vi "Copy of Copy of Sievert_auto_RLC-2.vi"() -> ()   [LabVIEW 2011]
uses:
  <vilib>/Utility/error.llb/DialogType.ctl
  <vilib>/DAQmx/write.llb/DAQmx Write (Digital Bool 1Line 1Point).vi
  <vilib>/DAQmx/create/channels.llb/DAQmx Create Channel (DO-Digital Output).vi
  <vilib>/DAQmx/miscellaneous.llb/DAQmx Fill In Error Info.vi
  <vilib>/Analysis/Matrix/Numeric/Conversions/Array To Matrix - RA.vi
  <vilib>/Analysis/Matrix/Numeric/Conversions/Matrix To Array - RM.vi
  <vilib>/Analysis/NI_AALPro.lvlib
  <vilib>/Analysis/Matrix/NI_Matrix.lvlib
  <vilib>/Analysis/NI_AALBase.lvlib
panel:
  out "Boolean 4":bool
  out "tempo carga":dbl[](array[numeric])
  out "PCh1":dbl[](array[numeric])
  out "output array 2":u32[](array[numeric])
  out "MEASURE C [F ]":dbl
  out "Automatico 2":dynamicdata(graph)
  out "termopar K 2":dbl format="%.3g"
  out "termopar K":string
  out "output NTC":dbl
  out "termopar K":dbl format="%.3g"
  out "path RLC_mean":path
  out "estagio 5":i32
  out "FIM":bool=TRUE
  out "limpo":i32
  in  "N fit":i32=5
  in  "ATM wait":u32
  in  "SET":i32
  in  "time subarray":dbl[](array[numeric])
  out "P cinetica mean 2":dbl format="%0.2f"
  out "T cinetica mean 3":dbl format="%0.2f"
  out "Time cinetica":dbl format="%0.2f"
  in  "T subarray 3":dbl[](array[numeric])
  in  "P T  index 2":i32
  in  "P subarray 2":dbl[](array[numeric])
  in  "Numeric":dbl=4.0
  in  "T subarray 2":dbl[](array[numeric])
  out "T cinetica mean 2":dbl format="%0.2f"
  out "P cinetica mean":dbl format="%0.2f"
  in  "P subarray":dbl[](array[numeric])
  in  "P T  index":i32
  out "T string":string
  out "P string":string
  out "path 2_cinetica":path
  out "Polynomial Coefficients 2":dbl[](array[numeric])
  out "Polynomial Coefficients":dbl[](array[numeric])
  in  "Count SET":i32=-1
  out "Set atual":i32
  out "mean pressure":dbl format="%.4p"
  out "Set number":i32
  in  "Tab Control":T1(tab)
  out "T":bool
  out "ZPf2":bool
  out "Pf2":bool
  out "Pit":bool
  out "ZPit":bool
  out "Camara":dbl(slide) scale=0.0..59.5 scale format="%#_3g"
  in  "Save manual":bool
  in  "Open Button":bool
  out "String 2":string
  in  "ATM":bool
  in  "Câmara":bool
  in  "Vácuo":bool
  in  "Entrada Gás":bool
  in  "Manual Ctrl":bool
  in  "stop":bool
  out "P-manual":dynamicdata(graph)
  in  "Clear":bool
  out "path":path
  in  "Nota":string
  in  "Sample name":string
  in  "File name":string
  out "Linear Model Graph":dbl[][](graph)
  out "Linear Model Graph 2":dbl[][](graph)
  in  "N to fit":i32=60
  out "N":i32
  out "Vácuo":bool
  out "Atm":bool
  out "Câmara":bool
  out "String_cinetica":string
  out "Vol Ref":dbl(slide) scale=0.0..60.0 scale format="%#_4f"
  out "Entrada gás":bool
  in  "Guardar\nCinetica":bool
  out "p fit":dbl format="%#_4g"
  out "T fit":dbl format="%#_4g"
  in  "Open Button 2":bool
  out "x >= y?":bool
  in  "seconds":dbl
  out "Elapsed Time (sec)":dbl format="%.1f"
  out "bar/N":dbl format="%#_4p"
  in  "correção NTC":dbl
  out "mean H2 sensor (V)":dbl format="%#_4p"
  out "Boolean 3":bool
  out "String 3":string
  out "T 2":bool
  out "ZPit 2":bool
  out "Pit 2":bool
  out "Pf2 2":bool
  out "ZPf2 2":bool
  out "Camara 2":dbl(slide) scale=0.0..25.0 scale format="%#_3g"
  out "Vácuo 2":bool
  out "Atm 2":bool
  out "Câmara 2":bool
  out "Vol Ref 3":dbl(slide) scale=0.0..25.0 scale format="%#_4f"
  out "Entrada gás 2":bool
  in  "Auto Ctrl":bool
  in  "Play Button":bool
  out "time stamp":timestamp format="%<%.2X>T"
  out "Time (sec)":dbl format="%.1f"
  in  "clear":bool
  out "Automatico":dynamicdata(graph)
  out "Linear P":T2(graph)
  out "Linear T":T2(graph)
  out "Contador":i32
  in  "STOP (bar/s)":dbl format="%#_5p"
  out "P (bar/s)":dbl format="%#_5p"
  out "bar/s":dbl format="%#_4p"
  out "P fit":dbl format="%#_4g"
  out "T fit":dbl format="%#_4g"
  out "x = y?":bool
  out "teste slope":i32
  in  "Set P auto":dbl
  in  "Step P":dbl=2.0
  in  "P_max":dbl=2.0
  in  "P_max camara":dbl=2.0
  out "Carga":bool=TRUE
  out "Descarga":bool
  out "String":string
  in  "P_min descarga":dbl
  in  "Boolean":bool
  in  "Array":dbl[](array[numeric])
  out "Boolean 2":bool
  out "Desc SET":i32
  in  "ZPf2 time":dbl=24.0
  in  "Ciclos":dbl
  out "Efetuados":dbl
  in  "patamar milliseconds to wait":u32=500
  in  "N fit patamar":i32=100
  in  "Step ZPit":dbl
  out "Read ZPit":bool
  in  "Estagio auto":i32
  out "mean H2 sensor":dbl format="%#_4p"
  in  "Ntest":i32=5
  in  "N fit 2":i32=100
  in  "C50L":bool
  in  "C50N":bool
  in  "C100L":bool
  in  "C100N":bool
  in  "C1KL":bool
  in  "C1KN":bool
  in  "C10KL":bool
  in  "C10KN":bool
  out "String 4":string
  in  "Combo Box":string(combo)
  in  "Refresh Button":bool
  in  "Close RLC 2":bool
  in  "RLC on/off":bool
  out "mean 16":dbl format="%.3p"
  out "mean 15":dbl format="%.3p"
  out "mean 14":dbl format="%.3p"
  out "mean 13":dbl format="%.3p"
  out "mean 12":dbl format="%.3p"
  out "mean 11":dbl format="%.3p"
  out "mean 10":dbl format="%.3p"
  out "mean 9":dbl format="%.3p"
  out "mean 8":dbl format="%.3p"
  out "mean 7":dbl format="%.3p"
  out "mean 6":dbl format="%.3p"
  out "mean 5":dbl format="%.3p"
  out "mean 4":dbl format="%.3p"
  out "mean 3":dbl format="%.3p"
  out "mean 2":dbl format="%.3p"
  out "mean":dbl format="%.3p"
  out "SET 2":dbl
  out "C-50-L":bool
  out "MEASURE B":dbl
  out "MEASURE A":dbl
  out "C-50-N":bool
  out "MEASURE B 2":dbl
  out "MEASURE A 2":dbl
  out "C-100-L":bool
  out "MEASURE B 3":dbl
  out "MEASURE A 3":dbl
  out "C-100-N":bool
  out "MEASURE B 4":dbl
  out "MEASURE A 4":dbl
  out "C-1K-L":bool
  out "MEASURE B 5":dbl
  out "MEASURE A 5":dbl
  out "C-1K-N":bool
  out "MEASURE B 6":dbl
  out "MEASURE A 6":dbl
  out "C-10K-L":bool
  out "MEASURE B 7":dbl
  out "MEASURE A 7":dbl
  out "C-10K-N":bool
  out "MEASURE B 8":dbl
  out "MEASURE A 8":dbl
  out "Z-50-L":bool
  out "MEASURE B 9":dbl
  out "MEASURE A 9":dbl
  out "Z-50-N":bool
  out "MEASURE B 10":dbl
  out "MEASURE A 10":dbl
  out "Z-100-L":bool
  out "MEASURE B 11":dbl
  out "MEASURE A 11":dbl
  out "Z-100-N":bool
  out "MEASURE B 12":dbl
  out "MEASURE A 12":dbl
  out "Z-1K-L":bool
  out "MEASURE B 13":dbl
  out "MEASURE A 13":dbl
  out "Z-1K-N":bool
  out "MEASURE B 14":dbl
  out "MEASURE A 14":dbl
  out "Z-10K-L":bool
  out "MEASURE B 15":dbl
  out "MEASURE A 15":dbl
  out "Z-10K-N":bool
  out "MEASURE B 16":dbl
  out "MEASURE A 16":dbl
  out "RLC300 - digimess":string
  in  "Time RLC":u32=5000
  in  "Ligar RLC":bool
  out "path RLC_completo":path
  out "Waveform Chart P 2":dbl[][](graph)
  out "Waveform Chart":dynamicdata(graph)
  in  "graph RLC":bool
  in  "Refresh Button 2":bool
  in  "Z50L":bool
  in  "Z50N":bool
  in  "Z100L":bool
  in  "Z100N":bool
  in  "Z1KL":bool
  in  "Z1KN":bool
  in  "Z10KL":bool
  in  "Z10KN":bool
  out "Waveform Chart 2":dynamicdata(graph)
  out "XY Graph 2":cluster{"Value":dbl[], "Value":dbl[]}[](graph)
  in  "t-sivert01(s)":dbl
  out "dP/dt (bar/s)":dbl format="%#_5p"
  in  "read - Sievert 01":bool
  # "P vol ref"
  # "P Câmara"
  # "P vol ref"
  # "P Câmara"
  # "C ( F )"
  # "R ( Ohm )"
  # "Z ( Ohm )"
  # "Phase ( deg)"
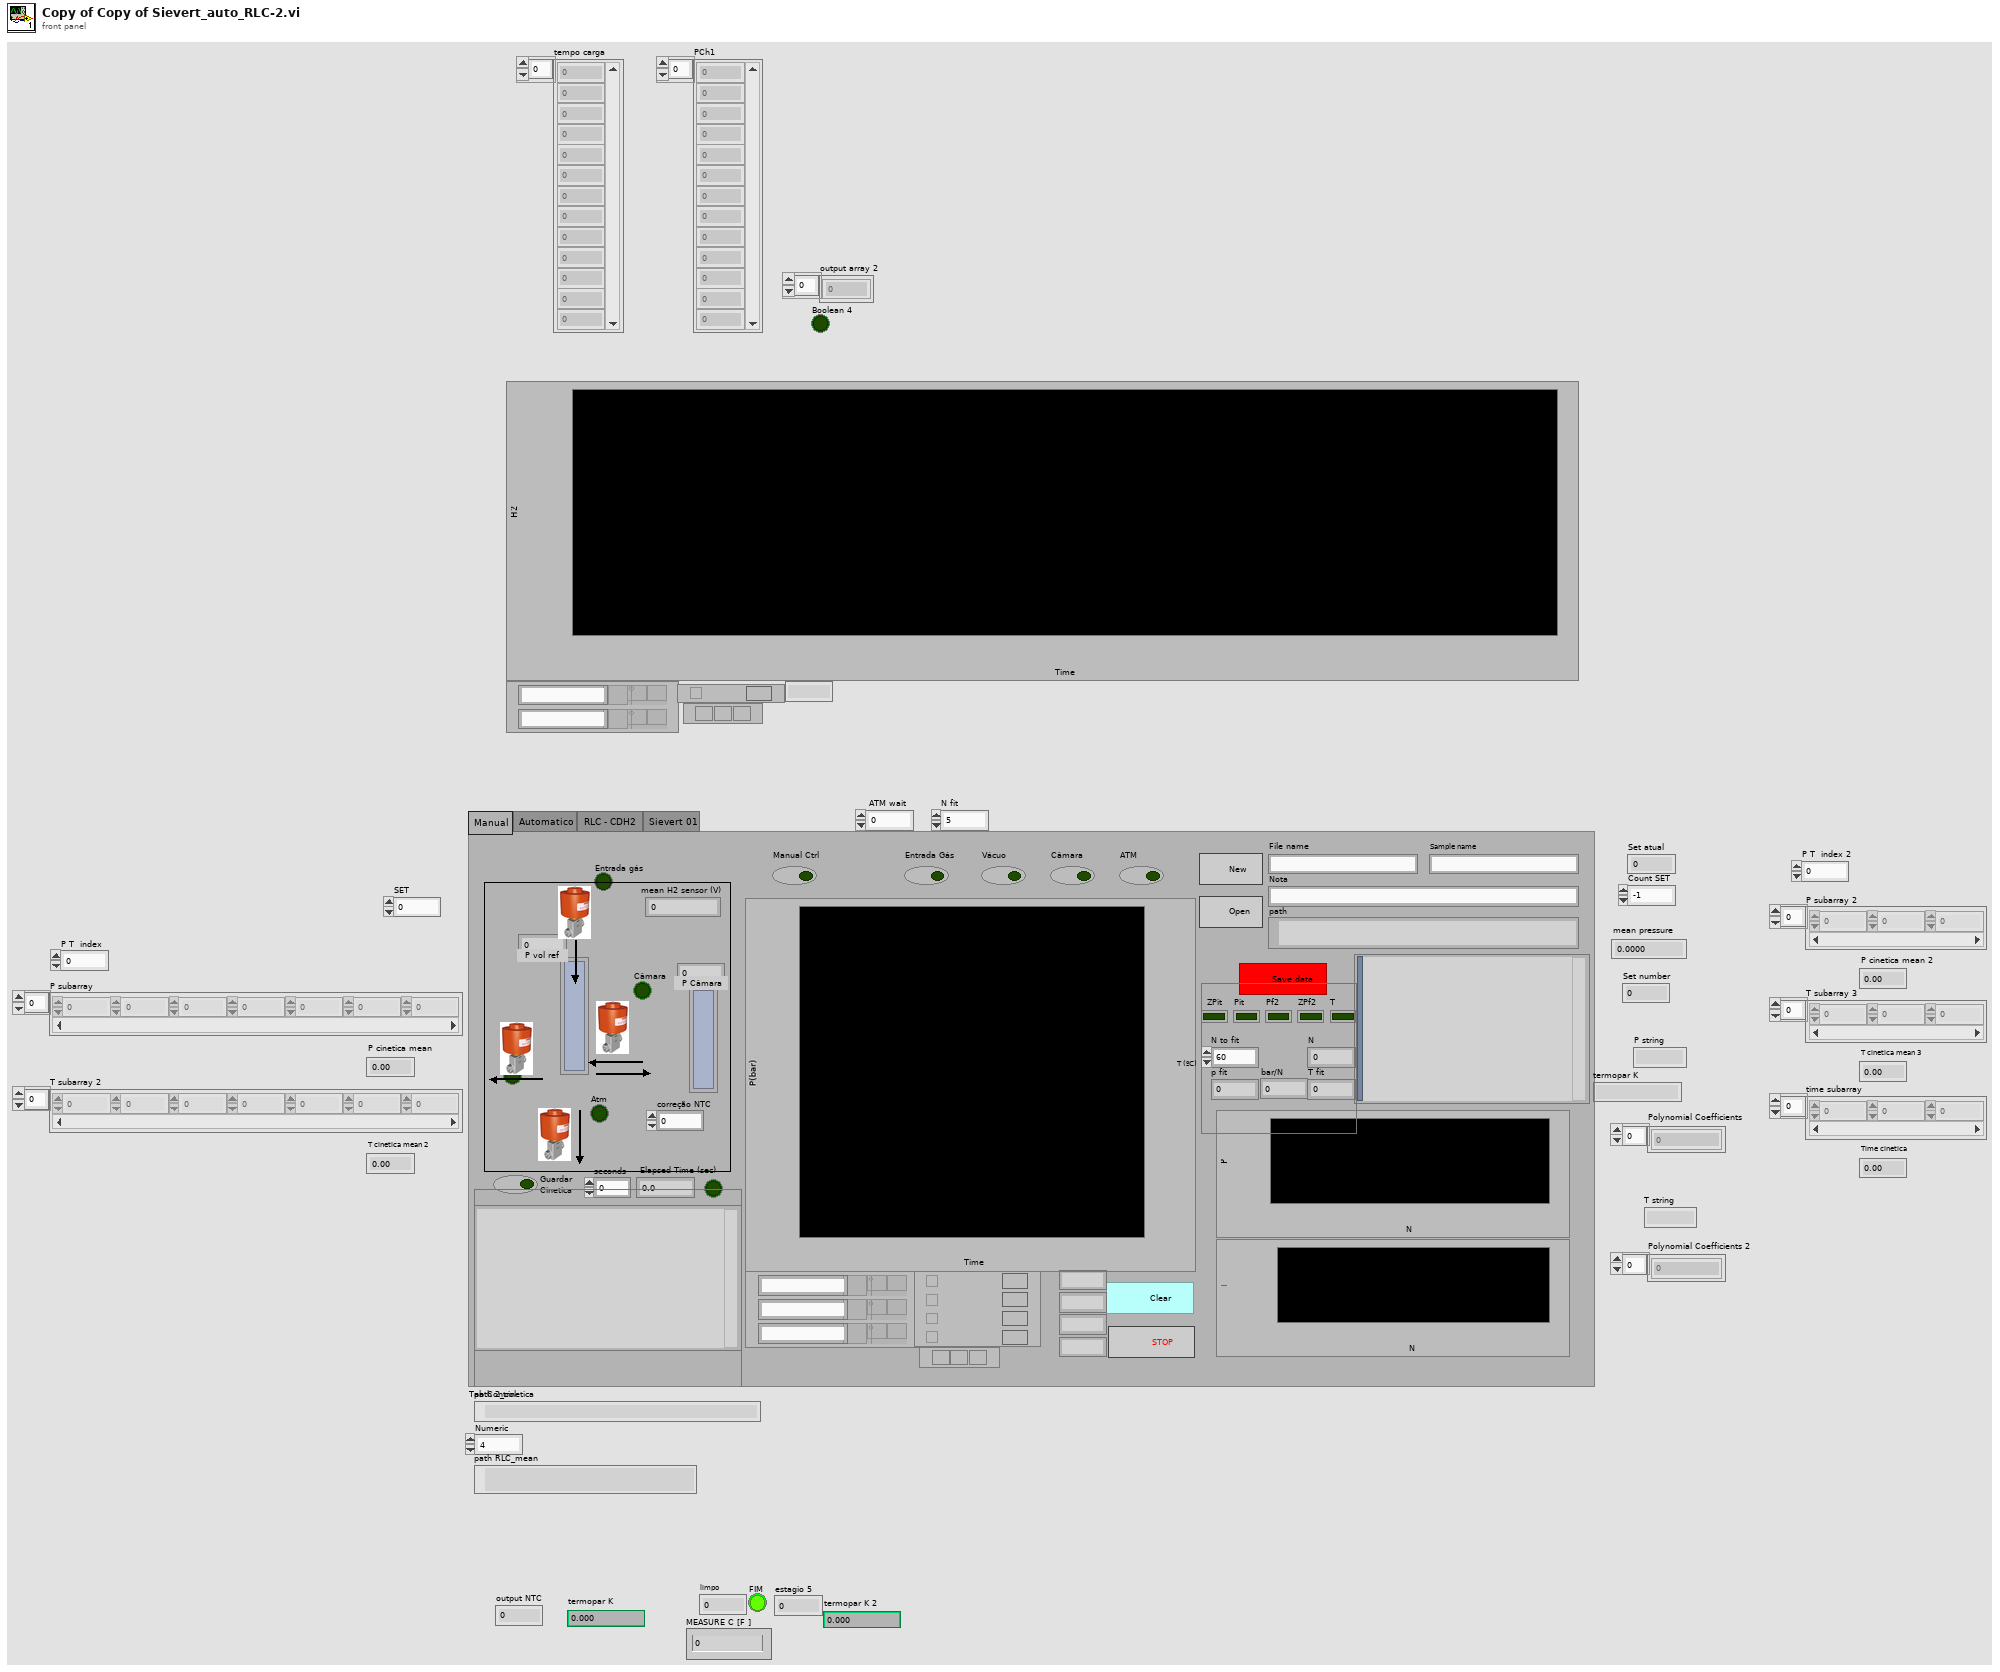
[diagram p1: front panel]
types:
  T1 = enum32{"Manual", "Automatico", "RLC - CDH2", "Sievert 01"}
  T2 = cluster{"Real 2D Array":dbl[], "Best Linear Fit":dbl[]}[]
  T3 = enum16{"open", "replace", "create", "open or create", "replace or create", "replace or create with confirmation"}
  T4 = cluster{"Value":dbl[], "Best Linear Fit":dbl[]}[]
  T5 = typedef "NI_Matrix.lvlib/RealMatrix.ctl" = dbl[][]
  T6 = cluster{"Real 2D Array":dbl[], "Real 2D Array":dbl[]}
  T7 = typedef "DialogType.ctl" = u16
  T8 = cluster{"Real 2D Array":dbl[], "Best Linear Fit":dbl[]}
  T9 = cluster{"Real 2D Array":dbl[], "Best Polynomial Fit":dbl[]}
  T10 = cluster{"Real 2D Array":dbl[], "Best Polynomial Fit":dbl[]}[]
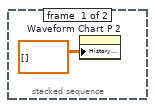
[diagram p5: hidden frame]
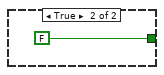
[diagram p10: hidden frame]
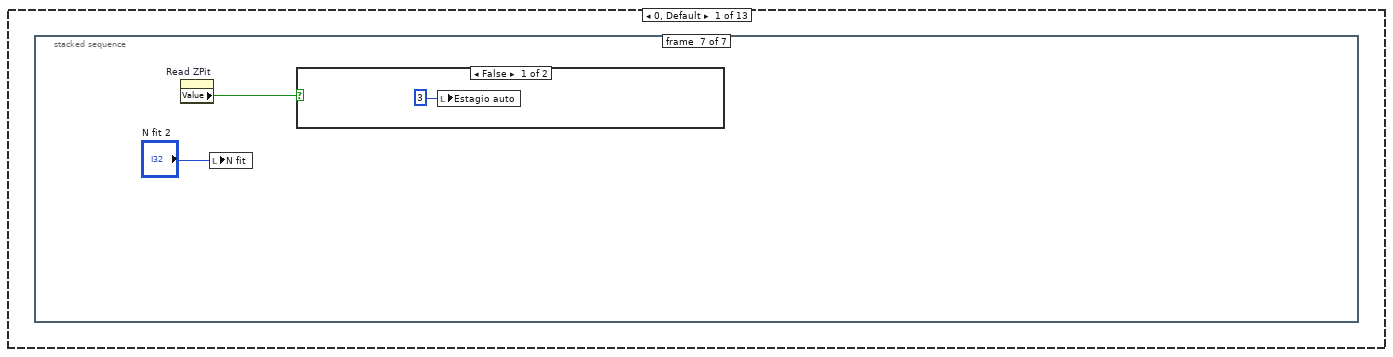
[diagram p15: hidden frame]
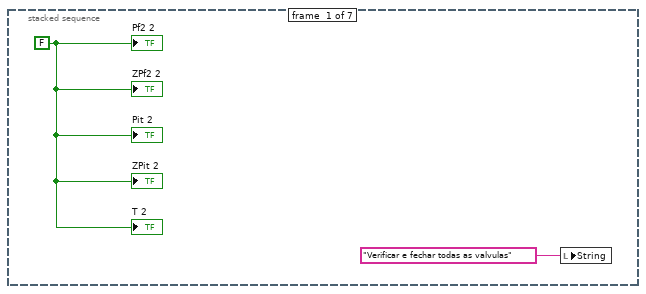
[diagram p16: hidden frame]
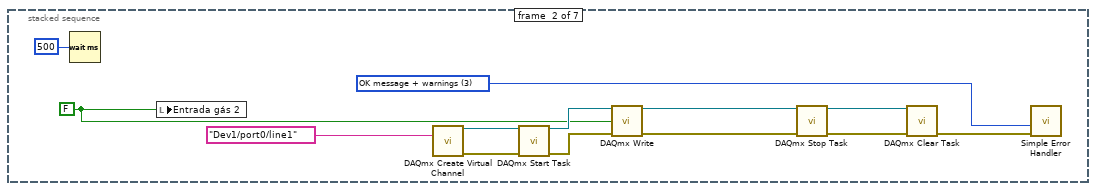
[diagram p17: hidden frame]
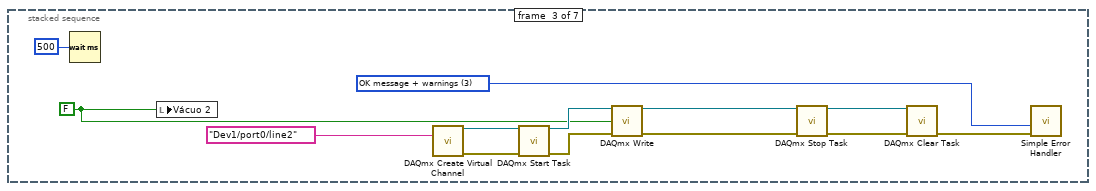
[diagram p18: hidden frame]
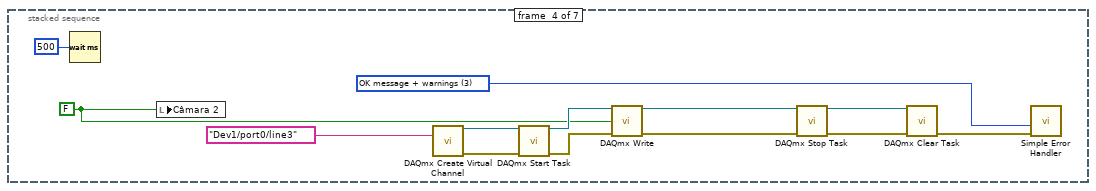
[diagram p19: hidden frame]
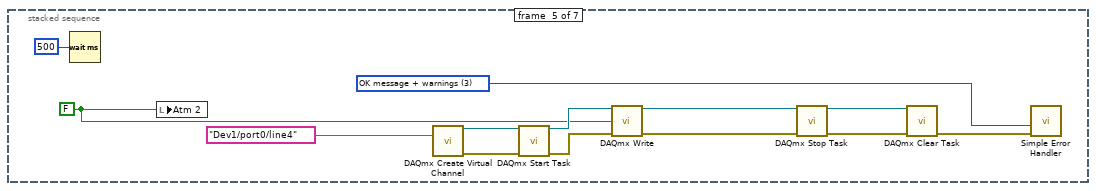
[diagram p20: hidden frame]
diagram:
  w1 = TRUE ("C1KN")
  (unwired) dbl[] [0.5, 1.0, 2.0, 3.0, 4.0, 5.0, 6.0, 7.0, 8.0, 9.0, 10.0, 11.0, 12.0, 13.0, 14.0, 15.0, 16.0, 17.0, 18.0, 19.0, 20.0, 30.0, 40.0, 50.0, 60.0, 70.0] ("Array")
  n1 = local write "N to fit"(5 ("Numeric")) -> ()
  n2 = local write "correção NTC"(0.5 ("correção NTC")) -> ()
  n3 = local write "Step ZPit"(5.0 ("Step ZPit")) -> ()
  n4 = local write "Time RLC"(u32 5 ("Time RLC")) -> ()
  n5 = local write "Ciclos"(0.0 ("Ciclos")) -> ()
  n6 = local write "Desc SET"(0 ("Desc SET")) -> ()
  n7 = local write "Efetuados"(0.0 ("Efetuados")) -> ()
  n8 = local write "estagio 5"(0 ("estagio 5")) -> ()
  n9 = local write "teste slope"(0 ("teste slope")) -> ()
  n10 = local write "SET"(0 ("SET auto")) -> ()
  n11 = local write "limpo"(0 ("limpo")) -> ()
  n12 = local write "N fit"(5 ("N fit")) -> ()
  n13 = local write "ATM wait"(u32 4 ("ATM wait")) -> ()
  n14 = local write "Estagio auto"(0 ("Estagio auto")) -> ()
  n15 = local write "P T  index"(0 ("index")) -> ()
  n16 = local write "seconds"(2.0 ("seconds")) -> ()
  n17 = local write "Read ZPit"(TRUE ("Read ZPit")) -> ()
  n18 = local write "Descarga"(FALSE ("Descarga")) -> ()
  n19 = local write "Carga"(TRUE ("Carga")) -> ()
  n20 = local write "FIM"(FALSE ("FIM")) -> ()
  n21 = local write "P_max"(50.0 ("P_max")) -> ()
  n22 = local write "P_max camara"(25.0 ("P_max camara")) -> ()
  n23 = local write "Set P auto"(0.5 ("Set P auto")) -> ()
  n24 = local write "P_min descarga"(0.025 ("P_min descarga")) -> ()
  n25 = local write "P subarray"(dbl[] [0.0, 1.0] ("subarray")) -> ()
  n26 = local write "T subarray 2"(dbl[] [0.0, 1.0] ("subarray")) -> ()
  n27 = local write "C1KN"(w1) -> ()
  n28 = local write "Z1KN"(w1) -> ()
  n29 = local write "Combo Box"("rlc_read_cCN.py" ("Combo Box")) -> ()
  n30 = local write "t-sivert01(s)"(10.0 ("t-sivert01(s)")) -> ()
  n31 = while {
    tunnel: path "C:/H2_Painel/painel_auto/RLC_CDH" ("Path") -> [w37]
    stop <- w49 stop-if-true
    n32 = property on="FIM" class="Bool (strict)"() -> ("Value"=w47:bool)  [unwired: 2 in, 2 out]
    n33 = property on="path" class="Path"() -> ("Value"=w44:path)  [unwired: 2 in, 2 out]
    n34 = case shown="True" "Ligar RLC" {
      tunnel: w37 -> [_ w224]
      frame False {
      }
      frame True {
        n35 = call "RLC_open.vi"("Path"=w224) -> ("String 2"=w225:string)  [unwired: 9 in, 1 out]
        n36 = local write "RLC300 - digimess"(w225) -> ()
      }
    }
    n37 = case shown="True" "Auto Ctrl" {
      tunnel: w37 -> [_ w230]
      tunnel: "RLC on/off" -> [_ w229]
      tunnel: [_ w228] -> w40
      frame False {
      }
      frame True {
        n38 = local write "P T  index 2"(0 ("P T  index")) -> ()
        n39 = for {
          N: "N fit" -> [w257]
          tunnel: w230 -> [w248]
          tunnel: w229 -> [w247]
          tunnel: [w246] -> w228
          i -> [w259]
          w263 = 0 ("polynomial order")
          w254 = 0 ("polynomial order")
          n40 = case shown="True" "clear" {
            frame False {
            }
            frame True {
              n41 = property on="Automatico 2" class="WFChart (strict)"("History Data"=dynamicdata[] []) -> ()  [unwired: 2 in, 2 out]
              n42 = property on="Linear P" class="XYGraph (strict)"("Value"=T2 [] ("Linear P")) -> ()  [unwired: 2 in, 2 out]
              n43 = property on="Linear T" class="XYGraph (strict)"("Value"=T2 [] ("Linear T")) -> ()  [unwired: 2 in, 2 out]
              n44 = property on="Automatico" class="WFChart (strict)"("History Data"=dynamicdata[] []) -> ()  [unwired: 2 in, 2 out]
            }
          }
          n45 = property on="path 2_cinetica" class="Path"() -> ("Value"=w251:path)  [unwired: 2 in, 2 out]
          n46 = call "Read P T.vi"("correção NTC"="correção NTC") -> ("Sievert01"=w238:dbl, "mean H2 sensor"=w243:dbl, "termopar K"=w240:dbl, "output NTC"=w241:dbl, "P Set 2 Output 2"=w242:dbl)  [unwired: 3 in, 7 out]
          "termopar K 2" <- w240
          "mean H2 sensor" <- w243
          n47 = Increment(x=w259) -> (x+1=w258:i32)
          n48 = Equal?(x=w258, y=w257) -> (x = y?=w260:bool)
          "x = y?" <- w260
          n49 = Merge Signals(w243) -> (→"Automatico 2":dynamicdata)
          n50 = Multiply(x=w242, y=10.0) -> (x*y=w253:dbl)
          n51 = Multiply(x=w238, y=10.0) -> (x*y=w237:dbl)
          n52 = case shown="True" "read - Sievert 01" {
            tunnel: w237 -> [_ w286]
            frame False {
            }
            frame True {
              n53 = Merge Signals(w286) -> (→"Waveform Chart 2":dynamicdata)
              n54 = flat-sequence {
                tunnel: w286 -> [w303]
                tunnel: [w301] -> w288
                frame #0 {
                  n55 = property on="Boolean 4" class="Bool (strict)"() -> ("Value"=w289:bool)  [unwired: 2 in, 2 out]
                  n56 = case shown="True" w289 {
                    frame False {
                    }
                    frame True {
                      n57 = local write "PCh1"(dbl[] [] ("PCh1")) -> ()
                      n58 = local write "tempo carga"(dbl[] [] ("tempo carga")) -> ()
                      n59 = local write "output array 2"(u32[] [] ("output array 2")) -> ()
                    }
                  }
                }
                frame #1 {
                  n60 = Tick Count (ms)() -> (millisecond timer value=w314:u32)
                  n61 = property on="output array 2" class="Arr (strict)"() -> ("Value"=w315:u32[])  [unwired: 2 in, 2 out]
                  n62 = Build Array(w314) -> (w308:u32[])
                  n63 = Insert Into Array(array=w315, new element=w308) -> (w309:u32[])  [unwired: 1 in]
                  "output array 2" <- w309
                  n64 = Array Max & Min(array=w309) -> (max value=w313:u32, min value=w312:u32)  [unwired: 2 out]
                  n65 = Subtract(x=w313, y=w312) -> (x-y=w310:u32)
                  n66 = Divide(x=w310, y=1000.0) -> (x/y=w300:dbl)
                  n67 = property on="PCh1" class="Arr (strict)"() -> ("Value"=w305:dbl[])  [unwired: 2 in, 2 out]
                  n68 = property on="tempo carga" class="Arr (strict)"() -> ("Value"=w306:dbl[])  [unwired: 2 in, 2 out]
                  n69 = Greater?(x=w300, y="t-sivert01(s)") -> (0:w301:bool)
                  n70 = Build Array(w300) -> (w307:dbl[])
                  n71 = Build Array(w303) -> (w304:dbl[])
                  n72 = Insert Into Array(array=w306, new element=w307) -> (w295:dbl[])  [unwired: 1 in]
                  "tempo carga" <- w295
                  n73 = Insert Into Array(array=w305, new element=w304) -> (w294:dbl[])  [unwired: 1 in]
                  "PCh1" <- w294
                  n74 = call <vilib>:"Linear Fit.vi"("Y"=w294, "X"=w295) -> ("Best Linear Fit"=w293:dbl[], "slope"=→"dP/dt (bar/s)":dbl)  [unwired: 9 in, 3 out]
                  n75 = Bundle("Value"=w295, "Value"=w294) -> (w298:cluster{"Value":dbl[], "Value":dbl[]})  [unwired: 1 in]
                  n76 = Bundle("Value"=w295, "Best Linear Fit"=w293) -> (w297:cluster{"Value":dbl[], "Best Linear Fit":dbl[]})  [unwired: 1 in]
                  n77 = Build Array(w298, w297) -> (→"XY Graph 2":T4)
                }
              }
              "Boolean 4" <- w288
            }
          }
          n78 = local write "Vol Ref 3"(w253) -> ()
          n79 = Merge Signals(w253, w241, w240, w237) -> (→"Automatico":dynamicdata)
          n80 = call "Elapsed Time2"("Reset"=w260) -> ("Elapsed Time (s)"=w274:dbl)  [unwired: 11 in, 7 out]
          "Time (sec)" <- w274
          n81 = stacked-sequence {
            tunnel: w253 -> [w1727 _]
            tunnel: w241 -> [w1713 _]
            tunnel: [w1694 _] -> w272
            tunnel: [w1710 _] -> w271
            tunnel: w274 -> [w1697 _]
            tunnel: [w1695 _] -> w268
            tunnel: [w1693 _] -> w250
            tunnel: [w1692 _] -> w249
            frame #0 {
              w1696 = 2 ("y")
              n82 = property on="P subarray 2" class="Arr (strict)"() -> ("Value"=w1729:dbl[])  [unwired: 2 in, 2 out]
              n83 = property on="T subarray 3" class="Arr (strict)"() -> ("Value"=w1719:dbl[])  [unwired: 2 in, 2 out]
              n84 = property on="time subarray" class="Arr (strict)"() -> ("Value"=w1706:dbl[])  [unwired: 2 in, 2 out]
              n85 = property on="P T  index 2" class="DigNum (strict)"() -> ("Value"=w1698:i32)  [unwired: 2 in, 2 out]
              n86 = Replace Array Subset(array=w1706, new element=w1697, index=w1698) -> (w1699:dbl[])
              n87 = Replace Array Subset(array=w1729, new element=w1727, index=w1698) -> (w1712:dbl[])
              n88 = Replace Array Subset(array=w1719, new element=w1713, index=w1698) -> (w1711:dbl[])
              n89 = call-poly <vilib>:"Array To Matrix.vi"("Real 1D Array"=w1699) -> ("Real Matrix (Column Vector)"=w1709:T5)
              n90 = call-poly <vilib>:"Array To Matrix.vi"("Real 1D Array"=w1712) -> ("Real Matrix (Column Vector)"=w1732:T5)
              n91 = call-poly <vilib>:"Array To Matrix.vi"("Real 1D Array"=w1711) -> ("Real Matrix (Column Vector)"=w1722:T5)
              n92 = Matrix Size(0:w1709) -> (1:w1708:i32, 2:w1707:i32)
              n93 = Matrix Size(0:w1732) -> (1:w1731:i32, 2:w1730:i32)
              n94 = Matrix Size(0:w1722) -> (1:w1721:i32, 2:w1720:i32)
              n95 = Increment(x=w1708) -> (x+1=w1700:i32)
              n96 = Increment(x=w1731) -> (x+1=w1723:i32)
              n97 = Increment(x=w1721) -> (x+1=w1714:i32)
              n98 = Subtract(x=w1700, y=w1696) -> (x-y=w1701:i32)
              n99 = Subtract(x=w1723, y=w1696) -> (x-y=w1724:i32)
              n100 = Subtract(x=w1714, y=w1696) -> (x-y=w1715:i32)
              n101 = Resize Matrix(1:w1707, 2:w1700, 4:w1709) -> (0:w1705:T5)
              n102 = Resize Matrix(1:w1730, 2:w1723, 4:w1732) -> (0:w1728:T5)
              n103 = Resize Matrix(1:w1720, 2:w1714, 4:w1722) -> (0:w1718:T5)
              n104 = call-poly <vilib>:"Matrix To Array.vi"("Real Matrix"=w1705) -> ("Real 2D Array"=w1703:dbl[][])
              n105 = call-poly <vilib>:"Matrix To Array.vi"("Real Matrix"=w1728) -> ("Real 2D Array"=w1726:dbl[][])
              n106 = call-poly <vilib>:"Matrix To Array.vi"("Real Matrix"=w1718) -> ("Real 2D Array"=w1717:dbl[][])
              n107 = Reshape Array(w1703, w1700) -> (w1702:dbl[])
              n108 = Reshape Array(w1726, w1723) -> (w1725:dbl[])
              n109 = Reshape Array(w1717, w1714) -> (w1716:dbl[])
              n110 = local write "time subarray"(w1702) -> ()
              n111 = local write "P subarray 2"(w1725) -> ()
              n112 = local write "T subarray 3"(w1716) -> ()
              n113 = Reshape Array(w1702, w1701) -> (w1695:dbl[])
              n114 = Reshape Array(w1725, w1724) -> (w1694:dbl[])
              n115 = Reshape Array(w1716, w1715) -> (w1710:dbl[])
              n116 = call <vilib>:"Mean.vi"("X"=w1695) -> ("mean"=→"Time cinetica":dbl)  [unwired: 1 out]
              n117 = call <vilib>:"Mean.vi"("X"=w1694) -> ("mean"=w1693:dbl)  [unwired: 1 out]
              "P cinetica mean 2" <- w1693
              n118 = call <vilib>:"Mean.vi"("X"=w1710) -> ("mean"=w1692:dbl)  [unwired: 1 out]
              "T cinetica mean 3" <- w1692
            }
            frame #1 {
              n119 = property on="P T  index 2" class="DigNum (strict)"() -> ("Value"=w1734:i32)  [unwired: 2 in, 2 out]
              n120 = Increment(x=w1734) -> (x+1=w1733:i32)
              n121 = local write "P T  index 2"(w1733) -> ()
            }
          }
          n122 = To Time Stamp(1:w274) -> (0:→"time stamp":timestamp)
          n123 = call <vilib>:"Linear Fit.vi"("Y"=w271, "X"=w268) -> ("Best Linear Fit"=w280:dbl[])  [unwired: 9 in, 4 out]
          n124 = Bundle("Real 2D Array"=w268, "Real 2D Array"=w271) -> (w278:T6)  [unwired: 1 in]
          n125 = Bundle("Real 2D Array"=w268, "Real 2D Array"=w272) -> (w277:T6)  [unwired: 1 in]
          n126 = call <vilib>:"General Polynomial Fit.vi"("Y"=w271, "polynomial order"=w254, "X"=w268) -> ("Best Polynomial Fit"=w269:dbl[], "Polynomial Coefficients"=w264:dbl[])  [unwired: 9 in, 2 out]
          n127 = call <vilib>:"General Polynomial Fit.vi"("Y"=w272, "polynomial order"=w254, "X"=w268) -> ("Best Polynomial Fit"=w270:dbl[], "Polynomial Coefficients"=w265:dbl[])  [unwired: 9 in, 2 out]
          n128 = call <vilib>:"Linear Fit.vi"("Y"=w272, "X"=w268) -> ("Best Linear Fit"=w275:dbl[], "slope"=w255:dbl)  [unwired: 9 in, 3 out]
          "bar/s" <- w255
          n129 = property on="path" class="Path"() -> ("Value"=w252:path)  [unwired: 2 in, 2 out]
          n130 = case shown="True" "Play Button" {
            tunnel: w252 -> [_ w324]
            tunnel: w253 -> [_ w323]
            tunnel: w251 -> [_ w322]
            tunnel: w250 -> [_ w321]
            tunnel: w249 -> [_ w320]
            tunnel: w248 -> [_ w319]
            tunnel: w247 -> [_ w318]
            tunnel: [_ w317] -> w246
            tunnel: w240 -> [_ w316]
            frame False {
            }
            frame True {
              n131 = case shown="8" "Estagio auto" {
                tunnel: w324 -> [_ _ _ w416 _ _ w569 _ w725 _ _ w1533 w1602]
                tunnel: w323 -> [_ w390 _ _ w465 w516 _ _ _ w1451 _ _ _]
                tunnel: w322 -> [_ _ _ _ _ _ _ w611 _ _ _ _ _]
                tunnel: w321 -> [_ _ _ _ _ _ _ w610 _ _ _ _ _]
                tunnel: w320 -> [_ _ _ _ _ _ _ w609 _ _ _ _ _]
                tunnel: w319 -> [_ _ _ _ _ _ _ _ w704 _ _ _ _]
                tunnel: w318 -> [_ _ _ _ _ _ _ _ w721 _ _ _ _]
                tunnel: [_ _ _ _ _ _ _ _ w703 _ _ _ _] -> w317
                tunnel: w316 -> [_ _ _ _ _ _ _ _ _ _ _ w1529 _]
                frame 0, Default {
                  n132 = stacked-sequence {
                    frame #0 {
                      w326 = FALSE ("Pit")
                      n133 = local write "String"("Verificar e fechar todas as valvulas" ("String")) -> ()
                      "ZPf2 2" <- w326
                      "Pf2 2" <- w326
                      "Pit 2" <- w326
                      "ZPit 2" <- w326
                      "T 2" <- w326
                    }
                    frame #1 {
                      w329 = FALSE ("Boolean 4")
                      w334 = T7 3 items=["no dialog", "OK message", "continue or stop message", "OK message + warnings", "continue/stop + warnings"] ("type of dialog (OK msg:1)")
                      n134 = Wait (ms)(milliseconds to wait=u32 500) -> ()  [unwired: 1 out]
                      n135 = local write "Entrada gás 2"(w329) -> ()
                      n136 = call-poly <vilib>:"DAQmx Create Virtual Channel.vi"("lines"=tag "Dev1/port0/line1") -> ("task out"=w332:refnum<k21>, "error out"=w333:errorcluster)  [unwired: 13 in]
                      n137 = call <vilib>:"DAQmx Start Task.vi"("task/channels in"=w332, "error in"=w333) -> ("task out"=w335:refnum<k21>, "error out"=w336:errorcluster)  [unwired: 12 in]
                      n138 = call-poly <vilib>:"DAQmx Write.vi"("task/channels in"=w335, "data"=w329, "error in"=w336) -> ("task out"=w340:refnum<k21>, "error out"=w337:errorcluster)  [unwired: 10 in, 1 out]
                      n139 = call <vilib>:"DAQmx Stop Task.vi"("task/channels in"=w340, "error in"=w337) -> ("task out"=w339:refnum<k21>, "error out"=w338:errorcluster)  [unwired: 12 in]
                      n140 = call <vilib>:"DAQmx Clear Task.vi"("task in"=w339, "error in"=w338) -> ("error out"=w331:errorcluster)  [unwired: 13 in]
                      n141 = call <vilib>:"Simple Error Handler.vi"("type of dialog (OK msg:1)"=w334, "error in (no error)"=w331) -> ()  [unwired: 3 in, 5 out]
                    }
                    frame #2 {
                      w342 = FALSE ("Boolean 4")
                      w347 = T7 3 items=["no dialog", "OK message", "continue or stop message", "OK message + warnings", "continue/stop + warnings"] ("type of dialog (OK msg:1)")
                      n142 = Wait (ms)(milliseconds to wait=u32 500) -> ()  [unwired: 1 out]
                      n143 = local write "Vácuo 2"(w342) -> ()
                      n144 = call-poly <vilib>:"DAQmx Create Virtual Channel.vi"("lines"=tag "Dev1/port0/line2") -> ("task out"=w345:refnum<k21>, "error out"=w346:errorcluster)  [unwired: 13 in]
                      n145 = call <vilib>:"DAQmx Start Task.vi"("task/channels in"=w345, "error in"=w346) -> ("task out"=w348:refnum<k21>, "error out"=w349:errorcluster)  [unwired: 12 in]
                      n146 = call-poly <vilib>:"DAQmx Write.vi"("task/channels in"=w348, "data"=w342, "error in"=w349) -> ("task out"=w353:refnum<k21>, "error out"=w350:errorcluster)  [unwired: 10 in, 1 out]
                      n147 = call <vilib>:"DAQmx Stop Task.vi"("task/channels in"=w353, "error in"=w350) -> ("task out"=w352:refnum<k21>, "error out"=w351:errorcluster)  [unwired: 12 in]
                      n148 = call <vilib>:"DAQmx Clear Task.vi"("task in"=w352, "error in"=w351) -> ("error out"=w344:errorcluster)  [unwired: 13 in]
                      n149 = call <vilib>:"Simple Error Handler.vi"("type of dialog (OK msg:1)"=w347, "error in (no error)"=w344) -> ()  [unwired: 3 in, 5 out]
                    }
                    frame #3 {
                      w355 = FALSE ("Boolean 4")
                      w360 = T7 3 items=["no dialog", "OK message", "continue or stop message", "OK message + warnings", "continue/stop + warnings"] ("type of dialog (OK msg:1)")
                      n150 = Wait (ms)(milliseconds to wait=u32 500) -> ()  [unwired: 1 out]
                      n151 = local write "Câmara 2"(w355) -> ()
                      n152 = call-poly <vilib>:"DAQmx Create Virtual Channel.vi"("lines"=tag "Dev1/port0/line3") -> ("task out"=w358:refnum<k21>, "error out"=w359:errorcluster)  [unwired: 13 in]
                      n153 = call <vilib>:"DAQmx Start Task.vi"("task/channels in"=w358, "error in"=w359) -> ("task out"=w361:refnum<k21>, "error out"=w362:errorcluster)  [unwired: 12 in]
                      n154 = call-poly <vilib>:"DAQmx Write.vi"("task/channels in"=w361, "data"=w355, "error in"=w362) -> ("task out"=w366:refnum<k21>, "error out"=w363:errorcluster)  [unwired: 10 in, 1 out]
                      n155 = call <vilib>:"DAQmx Stop Task.vi"("task/channels in"=w366, "error in"=w363) -> ("task out"=w365:refnum<k21>, "error out"=w364:errorcluster)  [unwired: 12 in]
                      n156 = call <vilib>:"DAQmx Clear Task.vi"("task in"=w365, "error in"=w364) -> ("error out"=w357:errorcluster)  [unwired: 13 in]
                      n157 = call <vilib>:"Simple Error Handler.vi"("type of dialog (OK msg:1)"=w360, "error in (no error)"=w357) -> ()  [unwired: 3 in, 5 out]
                    }
                    frame #4 {
                      w368 = FALSE ("Boolean 4")
                      w373 = T7 3 items=["no dialog", "OK message", "continue or stop message", "OK message + warnings", "continue/stop + warnings"] ("type of dialog (OK msg:1)")
                      n158 = Wait (ms)(milliseconds to wait=u32 500) -> ()  [unwired: 1 out]
                      n159 = local write "Atm 2"(w368) -> ()
                      n160 = call-poly <vilib>:"DAQmx Create Virtual Channel.vi"("lines"=tag "Dev1/port0/line4") -> ("task out"=w371:refnum<k21>, "error out"=w372:errorcluster)  [unwired: 13 in]
                      n161 = call <vilib>:"DAQmx Start Task.vi"("task/channels in"=w371, "error in"=w372) -> ("task out"=w374:refnum<k21>, "error out"=w375:errorcluster)  [unwired: 12 in]
                      n162 = call-poly <vilib>:"DAQmx Write.vi"("task/channels in"=w374, "data"=w368, "error in"=w375) -> ("task out"=w379:refnum<k21>, "error out"=w376:errorcluster)  [unwired: 10 in, 1 out]
                      n163 = call <vilib>:"DAQmx Stop Task.vi"("task/channels in"=w379, "error in"=w376) -> ("task out"=w378:refnum<k21>, "error out"=w377:errorcluster)  [unwired: 12 in]
                      n164 = call <vilib>:"DAQmx Clear Task.vi"("task in"=w378, "error in"=w377) -> ("error out"=w370:errorcluster)  [unwired: 13 in]
                      n165 = call <vilib>:"Simple Error Handler.vi"("type of dialog (OK msg:1)"=w373, "error in (no error)"=w370) -> ()  [unwired: 3 in, 5 out]
                    }
                    frame #5 {
                      n166 = Wait (ms)(milliseconds to wait=u32 500) -> ()  [unwired: 1 out]
                    }
                    frame #6 {
                      n167 = property on="Read ZPit" class="Bool (strict)"() -> ("Value"=w382:bool)  [unwired: 2 in, 2 out]
                      n168 = local write "N fit"("N fit 2") -> ()
                      n169 = case shown="False" w382 {
                        frame False {
                          n170 = local write "Estagio auto"(3 ("Estagio auto")) -> ()
                        }
                        frame True {
                          n171 = local write "Estagio auto"(1 ("Estagio auto")) -> ()
                        }
                      }
                    }
                  }
                }
                frame 1 {
                  n172 = Greater?(x=w390, y=1.0) -> (0:w389:bool)
                  n173 = case shown="True" w389 {
                    tunnel: [FALSE ("Boolean") TRUE ("Boolean")] -> w386
                    frame False {
                      w402 = TRUE ("Boolean")
                      n174 = local write "Vácuo 2"(w402) -> ()
                      n175 = call "Controle_vacuo.vi"("time (s) to wait vacuo"=u32 5, "Boolean"=w402) -> ("Vacuo"=w403:bool)  [unwired: 9 in]
                      n176 = local write "Vácuo 2"(w403) -> ()
                      n177 = local write "String"("Limpar volume referencia" ("String")) -> ()
                    }
                    frame True {
                      n178 = call "Controle_ATM.vi"("seconds to wait"="ATM wait") -> ("String 2"=w407:string, "Atm"=w406:bool)  [unwired: 9 in]
                      n179 = local write "Atm 2"(w406) -> ()
                      n180 = local write "String"(w407) -> ()
                    }
                  }
                  n181 = for {
                    N: 1 -> [_]
                    tunnel: [w392] -> w387
                    tunnel: w386 -> [w392]
                    n182 = Wait (ms)(milliseconds to wait=u32 500 ("x")) -> ()  [unwired: 1 out]
                  }
                  n183 = case shown="True" w387 {
                    frame False {
                      n184 = local write "Estagio auto"(2 ("Estagio auto")) -> ()
                    }
                    frame True {
                      w397 = TRUE ("Boolean")
                      n185 = local write "Estagio auto"(2 ("Estagio auto")) -> ()
                      n186 = local write "Vácuo 2"(w397) -> ()
                      n187 = call "Controle_vacuo.vi"("time (s) to wait vacuo"=u32 5, "Boolean"=w397) -> ("Vacuo"=w398:bool)  [unwired: 9 in]
                      n188 = local write "Vácuo 2"(w398) -> ()
                      n189 = local write "String"("Limpar volume referencia" ("String")) -> ()
                    }
                  }
                }
                frame 2 {
                  n190 = property on="Contador" class="DigNum (strict)"() -> ("Value"=w411:i32)  [unwired: 2 in, 2 out]
                  n191 = local write "String"("Ler ZPit" ("String")) -> ()
                  n192 = Increment(x=w411) -> (x+1=w410:i32)
                  n193 = property on="N fit 2" class="DigNum (strict)"() -> ("Value"=w408:i32)  [unwired: 2 in, 2 out]
                  n194 = Equal?(x=w410, y=w408) -> (x = y?=w409:bool)
                  n195 = case shown="True" w409 {
                    frame False {
                    }
                    frame True {
                      n196 = local write "Estagio auto"(3 ("Estagio auto")) -> ()
                    }
                  }
                }
                frame 3 {
                  w419 = "\t"
                  n197 = property on="SET" class="DigNum (strict)"() -> ("Value"=w415:i32)  [unwired: 2 in, 2 out]
                  n198 = property on="Read ZPit" class="Bool (strict)"() -> ("Value"=w414:bool)  [unwired: 2 in, 2 out]
                  n199 = case shown="False" w414 {
                    tunnel: ["  ==>" w426] -> w420
                    frame False {
                    }
                    frame True {
                      n200 = property on="P fit" class="DigNum (strict)"() -> ("Value"=w425:dbl)  [unwired: 2 in, 2 out]
                      n201 = Number To Fractional String(number=w425, precision (6)=i16 3) -> (F-format string=w426:string)  [unwired: 2 in]
                    }
                  }
                  n202 = Number To Decimal String(number=w415) -> (decimal integer string=w418:string)  [unwired: 1 in]
                  n203 = Concatenate Strings(w418, w419, w420, w419) -> (w417:string)
                  n204 = flat-sequence {
                    tunnel: [w430] -> w422
                    tunnel: [w429] -> w421
                    tunnel: w417 -> [w428]
                    tunnel: w416 -> [w427]
                    tunnel: w422 -> [w446]
                    tunnel: w421 -> [w445]
                    frame #0 {
                      n205 = Open/Create/Replace File(file path (use dialog)=w427, operation (0:open)=T3."open") -> (refnum out=w436:refnum<file>, error out=w437:errorcluster)  [unwired: 2 in, 3 out]
                      n206 = Set File Position(refnum=w436, from (0:start)=enum16{"start", "end", "current"}."end", error in=w437) -> (refnum out=w434:refnum<file>, error out=w433:errorcluster)  [unwired: 1 in]
                      n207 = Write to Text File(file (use dialog)=w434, text=w428, error in=w433) -> (refnum out=w438:refnum<file>, error out=w439:errorcluster)  [unwired: 2 out]
                      n208 = Close File(refnum=w438, error in=w439) -> (path=w430:path, error out=w431:errorcluster)
                      n209 = call <vilib>:"Simple Error Handler.vi"("error in (no error)"=w431) -> ("error out"=w429:errorcluster)  [unwired: 1 in, 7 out]
                    }
                    frame #1 {
                      w440 = 0 ("limpo")
                      n210 = local write "Estagio auto"(4 ("Estagio auto")) -> ()
                      n211 = local write "ZPit 2"(TRUE ("ZPit")) -> ()
                      n212 = Wait (ms)(milliseconds to wait=u32 500) -> ()  [unwired: 1 out]
                      n213 = local write "limpo"(w440) -> ()
                      n214 = Read from Text File(file (use dialog)=w446, count=-1 ("Count  3"), error in=w445) -> (refnum out=w447:refnum<file>, text=w451:string, error out=w448:errorcluster)  [unwired: 1 in, 1 out]
                      n215 = local write "String 3"(w451) -> ()
                      n216 = local write "estagio 5"(w440) -> ()
                      n217 = Close File(refnum=w447, error in=w448) -> (error out=w449:errorcluster)  [unwired: 1 out]
                      n218 = call <vilib>:"Simple Error Handler.vi"("error in (no error)"=w449) -> ()  [unwired: 1 in, 8 out]
                      n219 = local write "String"("abrir valvula entrada gas" ("String")) -> ()
                    }
                    frame #2 {
                      w452 = T7 3 items=["no dialog", "OK message", "continue or stop message", "OK message + warnings", "continue/stop + warnings"] ("type of dialog (OK msg:1)")
                      w458 = TRUE ("Boolean 4")
                      n220 = local write "Entrada gás 2"(w458) -> ()
                      n221 = call-poly <vilib>:"DAQmx Create Virtual Channel.vi"("lines"=tag "Dev1/port0/line1") -> ("task out"=w460:refnum<k21>, "error out"=w461:errorcluster)  [unwired: 13 in]
                      n222 = call <vilib>:"DAQmx Start Task.vi"("task/channels in"=w460, "error in"=w461) -> ("task out"=w462:refnum<k21>, "error out"=w463:errorcluster)  [unwired: 12 in]
                      n223 = call-poly <vilib>:"DAQmx Write.vi"("task/channels in"=w462, "data"=w458, "error in"=w463) -> ("task out"=w455:refnum<k21>, "error out"=w454:errorcluster)  [unwired: 10 in, 1 out]
                      n224 = call <vilib>:"DAQmx Stop Task.vi"("task/channels in"=w455, "error in"=w454) -> ("task out"=w456:refnum<k21>, "error out"=w457:errorcluster)  [unwired: 12 in]
                      n225 = call <vilib>:"DAQmx Clear Task.vi"("task in"=w456, "error in"=w457) -> ("error out"=w453:errorcluster)  [unwired: 13 in]
                      n226 = call <vilib>:"Simple Error Handler.vi"("type of dialog (OK msg:1)"=w452, "error in (no error)"=w453) -> ()  [unwired: 3 in, 5 out]
                    }
                  }
                }
                frame 4 {
                  n227 = Greater Or Equal?(x=w465, y="Set P auto") -> (x >= y?=w466:bool)
                  n228 = case shown="True" w466 {
                    tunnel: "Set P auto" -> [_ w481]
                    frame False {
                      w474 = T7 3 items=["no dialog", "OK message", "continue or stop message", "OK message + warnings", "continue/stop + warnings"] ("type of dialog (OK msg:1)")
                      w480 = TRUE ("data")
                      n229 = local write "Estagio auto"(5 ("Estagio auto")) -> ()
                      n230 = Wait (ms)(milliseconds to wait=u32 500) -> ()  [unwired: 1 out]
                      n231 = local write "Entrada gás 2"(w480) -> ()
                      n232 = call-poly <vilib>:"DAQmx Create Virtual Channel.vi"("lines"=tag "Dev1/port0/line1") -> ("task out"=w471:refnum<k21>, "error out"=w470:errorcluster)  [unwired: 13 in]
                      n233 = call <vilib>:"DAQmx Start Task.vi"("task/channels in"=w471, "error in"=w470) -> ("task out"=w469:refnum<k21>, "error out"=w468:errorcluster)  [unwired: 12 in]
                      n234 = call-poly <vilib>:"DAQmx Write.vi"("task/channels in"=w469, "data"=w480, "error in"=w468) -> ("task out"=w477:refnum<k21>, "error out"=w476:errorcluster)  [unwired: 10 in, 1 out]
                      n235 = call <vilib>:"DAQmx Stop Task.vi"("task/channels in"=w477, "error in"=w476) -> ("task out"=w479:refnum<k21>, "error out"=w478:errorcluster)  [unwired: 12 in]
                      n236 = call <vilib>:"DAQmx Clear Task.vi"("task in"=w479, "error in"=w478) -> ("error out"=w475:errorcluster)  [unwired: 13 in]
                      n237 = call <vilib>:"Simple Error Handler.vi"("type of dialog (OK msg:1)"=w474, "error in (no error)"=w475) -> ()  [unwired: 3 in, 5 out]
                    }
                    frame True {
                      n238 = flat-sequence {
                        tunnel: [w484] -> w482
                        tunnel: w481 -> [w484]
                        tunnel: [w499] -> w483
                        tunnel: w482 -> [w498]
                        tunnel: w483 -> [w513]
                        frame #0 {
                          w490 = T7 3 items=["no dialog", "OK message", "continue or stop message", "OK message + warnings", "continue/stop + warnings"] ("type of dialog (OK msg:1)")
                          w497 = FALSE ("data")
                          n239 = Wait (ms)(milliseconds to wait=u32 500) -> ()  [unwired: 1 out]
                          n240 = local write "Entrada gás 2"(w497) -> ()
                          n241 = call-poly <vilib>:"DAQmx Create Virtual Channel.vi"("lines"=tag "Dev1/port0/line1") -> ("task out"=w488:refnum<k21>, "error out"=w489:errorcluster)  [unwired: 13 in]
                          n242 = call <vilib>:"DAQmx Start Task.vi"("task/channels in"=w488, "error in"=w489) -> ("task out"=w486:refnum<k21>, "error out"=w485:errorcluster)  [unwired: 12 in]
                          n243 = call-poly <vilib>:"DAQmx Write.vi"("task/channels in"=w486, "data"=w497, "error in"=w485) -> ("task out"=w494:refnum<k21>, "error out"=w493:errorcluster)  [unwired: 10 in, 1 out]
                          n244 = call <vilib>:"DAQmx Stop Task.vi"("task/channels in"=w494, "error in"=w493) -> ("task out"=w496:refnum<k21>, "error out"=w495:errorcluster)  [unwired: 12 in]
                          n245 = call <vilib>:"DAQmx Clear Task.vi"("task in"=w496, "error in"=w495) -> ("error out"=w491:errorcluster)  [unwired: 13 in]
                          n246 = call <vilib>:"Simple Error Handler.vi"("type of dialog (OK msg:1)"=w490, "error in (no error)"=w491) -> ()  [unwired: 3 in, 5 out]
                        }
                        frame #1 {
                          n247 = stacked-sequence {
                            tunnel: [_ _ _ w510] -> w499
                            tunnel: w498 -> [_ _ w503 _]
                            frame #0 {
                              n248 = call "Controle_ATM.vi"("seconds to wait"=2.0) -> ("Atm"=w501:bool)  [unwired: 9 in, 1 out]
                              n249 = local write "Atm 2"(w501) -> ()
                            }
                            frame #1 {
                              n250 = Wait (ms)(milliseconds to wait=u32 1000) -> ()  [unwired: 1 out]
                            }
                            frame #2 {
                              n251 = Less Or Equal?(x=w503, y=1.5) -> (x <= y?=w505:bool)
                              n252 = case shown="True" w505 {
                                frame False {
                                n253 = call "Controle_ATM.vi"("seconds to wait"=2.0) -> ()  [unwired: 9 in, 2 out]
                                }
                                frame True {
                                w508 = TRUE ("Vácuo")
                                n254 = local write "Vácuo 2"(w508) -> ()
                                n255 = call "Controle_vacuo.vi"("time (s) to wait vacuo"=3.0, "Boolean"=w508) -> ("Vacuo"=w509:bool)  [unwired: 9 in]
                                n256 = local write "Vácuo 2"(w509) -> ()
                                }
                              }
                            }
                            frame #3 {
                              n257 = property on="limpo" class="DigNum (strict)"() -> ("Value"=w511:i32)  [unwired: 2 in, 2 out]
                              n258 = Wait (ms)(milliseconds to wait=u32 1000) -> ()  [unwired: 1 out]
                              n259 = Increment(x=w511) -> (x+1=w510:i32)
                            }
                          }
                        }
                        frame #2 {
                          "limpo" <- w513
                        }
                      }
                    }
                  }
                }
                frame 5 {
                  n260 = property on="Set P auto" class="DigNum (strict)"() -> ("Value"=w515:dbl)  [unwired: 2 in, 2 out]
                  n261 = Greater Or Equal?(x=w516, y=w515) -> (x >= y?=w514:bool)
                  n262 = case shown="True" w514 {
                    selector: w514 -> [_ w538]
                    frame False {
                      n263 = flat-sequence {
                        tunnel: [w518] -> w517
                        tunnel: w517 -> [w534]
                        frame #0 {
                          w521 = T7 3 items=["no dialog", "OK message", "continue or stop message", "OK message + warnings", "continue/stop + warnings"] ("type of dialog (OK msg:1)")
                          w531 = TRUE ("Boolean 4")
                          n264 = property on="estagio 5" class="DigNum (strict)"() -> ("Value"=w519:i32)  [unwired: 2 in, 2 out]
                          n265 = local write "Entrada gás 2"(w531) -> ()
                          n266 = Increment(x=w519) -> (x+1=w518:i32)
                          n267 = call-poly <vilib>:"DAQmx Create Virtual Channel.vi"("lines"=tag "Dev1/port0/line1") -> ("task out"=w525:refnum<k21>, "error out"=w524:errorcluster)  [unwired: 13 in]
                          n268 = call <vilib>:"DAQmx Start Task.vi"("task/channels in"=w525, "error in"=w524) -> ("task out"=w523:refnum<k21>, "error out"=w522:errorcluster)  [unwired: 12 in]
                          n269 = call-poly <vilib>:"DAQmx Write.vi"("task/channels in"=w523, "data"=w531, "error in"=w522) -> ("task out"=w528:refnum<k21>, "error out"=w527:errorcluster)  [unwired: 10 in, 1 out]
                          n270 = call <vilib>:"DAQmx Stop Task.vi"("task/channels in"=w528, "error in"=w527) -> ("task out"=w529:refnum<k21>, "error out"=w530:errorcluster)  [unwired: 12 in]
                          n271 = call <vilib>:"DAQmx Clear Task.vi"("task in"=w529, "error in"=w530) -> ("error out"=w520:errorcluster)  [unwired: 13 in]
                          n272 = call <vilib>:"Simple Error Handler.vi"("type of dialog (OK msg:1)"=w521, "error in (no error)"=w520) -> ()  [unwired: 3 in, 5 out]
                        }
                        frame #1 {
                          n273 = Less?(x=w534, y=6) -> (x < y?=w532:bool)
                          n274 = case shown="False" w532 {
                            frame False {
                              n275 = local write "Estagio auto"(5 ("Estagio auto")) -> ()
                            }
                            frame True {
                              n276 = local write "Estagio auto"(4 ("Estagio auto")) -> ()
                            }
                          }
                          "estagio 5" <- w534
                        }
                      }
                    }
                    frame True {
                      n277 = flat-sequence {
                        tunnel: w538 -> [w539]
                        tunnel: [w539] -> w537
                        tunnel: w537 -> [w555]
                        frame #0 {
                          w540 = FALSE ("Boolean 4")
                          w545 = T7 3 items=["no dialog", "OK message", "continue or stop message", "OK message + warnings", "continue/stop + warnings"] ("type of dialog (OK msg:1)")
                          n278 = local write "Entrada gás 2"(w540) -> ()
                          n279 = call-poly <vilib>:"DAQmx Create Virtual Channel.vi"("lines"=tag "Dev1/port0/line1") -> ("task out"=w543:refnum<k21>, "error out"=w544:errorcluster)  [unwired: 13 in]
                          n280 = call <vilib>:"DAQmx Start Task.vi"("task/channels in"=w543, "error in"=w544) -> ("task out"=w546:refnum<k21>, "error out"=w547:errorcluster)  [unwired: 12 in]
                          n281 = call-poly <vilib>:"DAQmx Write.vi"("task/channels in"=w546, "data"=w540, "error in"=w547) -> ("task out"=w551:refnum<k21>, "error out"=w548:errorcluster)  [unwired: 10 in, 1 out]
                          n282 = call <vilib>:"DAQmx Stop Task.vi"("task/channels in"=w551, "error in"=w548) -> ("task out"=w550:refnum<k21>, "error out"=w549:errorcluster)  [unwired: 12 in]
                          n283 = call <vilib>:"DAQmx Clear Task.vi"("task in"=w550, "error in"=w549) -> ("error out"=w542:errorcluster)  [unwired: 13 in]
                          n284 = call <vilib>:"Simple Error Handler.vi"("type of dialog (OK msg:1)"=w545, "error in (no error)"=w542) -> ()  [unwired: 3 in, 5 out]
                        }
                        frame #1 {
                          n285 = property on="estagio 5" class="DigNum (strict)"() -> ("Value"=w553:i32)  [unwired: 2 in, 2 out]
                          n286 = Greater?(x=w553, y=5) -> (0:w556:bool)
                          n287 = And(x=w555, y=w556) -> (x .and. y?=w554:bool)
                          n288 = case shown="True" w554 {
                            frame False {
                              n289 = local write "Estagio auto"(4 ("Estagio auto")) -> ()
                              n290 = Wait (ms)(milliseconds to wait=u32 500) -> ()  [unwired: 1 out]
                            }
                            frame True {
                              n291 = property on="Contador" class="DigNum (strict)"() -> ("Value"=w560:i32)  [unwired: 2 in, 2 out]
                              n292 = local write "String"("Ler Pit" ("String")) -> ()
                              n293 = Increment(x=w560) -> (x+1=w562:i32)
                              n294 = property on="N fit 2" class="DigNum (strict)"() -> ("Value"=w559:i32)  [unwired: 2 in, 2 out]
                              n295 = Equal?(x=w562, y=w559) -> (x = y?=w561:bool)
                              n296 = case shown="True" w561 {
                                frame False {
                                }
                                frame True {
                                n297 = local write "Estagio auto"(6 ("Estagio auto")) -> ()
                                }
                              }
                            }
                          }
                        }
                      }
                    }
                  }
                }
                frame 6 {
                  n298 = property on="Contador" class="DigNum (strict)"() -> ("Value"=w566:i32)  [unwired: 2 in, 2 out]
                  n299 = Increment(x=w566) -> (x+1=w568:i32)
                  n300 = property on="N fit 2" class="DigNum (strict)"() -> ("Value"=w565:i32)  [unwired: 2 in, 2 out]
                  n301 = Equal?(x=w568, y=w565) -> (x = y?=w567:bool)
                  n302 = case shown="True" w567 {
                    tunnel: w569 -> [_ w570]
                    frame False {
                    }
                    frame True {
                      n303 = property on="P fit" class="DigNum (strict)"() -> ("Value"=w571:dbl)  [unwired: 2 in, 2 out]
                      n304 = Number To Fractional String(number=w571, precision (6)=i16 3) -> (F-format string=w575:string)  [unwired: 2 in]
                      n305 = Concatenate Strings(w575, "\t") -> (w573:string)
                      n306 = flat-sequence {
                        tunnel: [w581] -> w577
                        tunnel: [w580] -> w576
                        tunnel: w573 -> [w579]
                        tunnel: w570 -> [w578]
                        tunnel: w577 -> [w597]
                        tunnel: w576 -> [w596]
                        frame #0 {
                          n307 = Open/Create/Replace File(file path (use dialog)=w578, operation (0:open)=T3."open") -> (refnum out=w587:refnum<file>, error out=w588:errorcluster)  [unwired: 2 in, 3 out]
                          n308 = Set File Position(refnum=w587, from (0:start)=enum16{"start", "end", "current"}."end", error in=w588) -> (refnum out=w585:refnum<file>, error out=w584:errorcluster)  [unwired: 1 in]
                          n309 = Write to Text File(file (use dialog)=w585, text=w579, error in=w584) -> (refnum out=w589:refnum<file>, error out=w590:errorcluster)  [unwired: 2 out]
                          n310 = Close File(refnum=w589, error in=w590) -> (path=w581:path, error out=w582:errorcluster)
                          n311 = call <vilib>:"Simple Error Handler.vi"("error in (no error)"=w582) -> ("error out"=w580:errorcluster)  [unwired: 1 in, 7 out]
                        }
                        frame #1 {
                          n312 = local write "Estagio auto"(7 ("Estagio auto")) -> ()
                          n313 = local write "teste slope"(0 ("teste slope")) -> ()
                          n314 = local write "Pit 2"(TRUE ("ZPit")) -> ()
                          n315 = Wait (ms)(milliseconds to wait=u32 500) -> ()  [unwired: 1 out]
                          n316 = Read from Text File(file (use dialog)=w597, count=-1 ("Count  3"), error in=w596) -> (refnum out=w598:refnum<file>, text=w602:string, error out=w599:errorcluster)  [unwired: 1 in, 1 out]
                          n317 = local write "String 3"(w602) -> ()
                          n318 = Close File(refnum=w598, error in=w599) -> (error out=w600:errorcluster)  [unwired: 1 out]
                          n319 = call <vilib>:"Simple Error Handler.vi"("error in (no error)"=w600) -> ()  [unwired: 1 in, 8 out]
                          n320 = local write "String"("abrir valvula entrada camara" ("String")) -> ()
                        }
                      }
                    }
                  }
                }
                frame 7 {
                  n321 = flat-sequence {
                    tunnel: w609 -> [w613]
                    tunnel: w610 -> [w614]
                    tunnel: w611 -> [w615]
                    tunnel: [w615] -> w608
                    tunnel: [w614] -> w606
                    tunnel: [w613] -> w604
                    tunnel: w608 -> [w618]
                    tunnel: [w618] -> w607
                    tunnel: w606 -> [w616]
                    tunnel: [w616] -> w605
                    tunnel: w604 -> [w617]
                    tunnel: [w617] -> w603
                    tunnel: w607 -> [_]
                    tunnel: w605 -> [_]
                    tunnel: w603 -> [_]
                    frame #0 {
                      n322 = local write "N fit"("N fit patamar") -> ()
                    }
                    frame #1 {
                      n323 = flat-sequence {
                        tunnel: w618 -> [w623]
                        tunnel: w616 -> [w622]
                        tunnel: w617 -> [w621]
                        frame #0 {
                          (unwired) i16 6 ("precision (6)")
                          w620 = "\t"
                          w640 = i16 4 ("precision (6)")
                          n324 = Number To Fractional String(number=w622, precision (6)=w640) -> (F-format string=w635:string)  [unwired: 2 in]
                          n325 = Number To Fractional String(number=w621, precision (6)=w640) -> (F-format string=w634:string)  [unwired: 2 in]
                          n326 = Get Date/Time String(date format (0)=enum16{"short", "long", "abbreviated"}."short", want seconds? (F)=TRUE) -> (date string=w637:string, time string=w636:string)  [unwired: 1 in]
                          n327 = Open/Create/Replace File(file path (use dialog)=w623, operation (0:open)=T3."open") -> (refnum out=w631:refnum<file>, error out=w624:errorcluster)  [unwired: 2 in, 3 out]
                          n328 = Concatenate Strings(w637, w620, w636, w620, w635, w620, w634, w620, w620, "\r\n") -> (w625:string)
                          n329 = Set File Position(refnum=w631, from (0:start)=enum16{"start", "end", "current"}."end", error in=w624) -> (refnum out=w629:refnum<file>, error out=w628:errorcluster)  [unwired: 1 in]
                          n330 = Write to Text File(file (use dialog)=w629, text=w625, error in=w628) -> (refnum out=w632:refnum<file>, error out=w633:errorcluster)  [unwired: 2 out]
                          n331 = Close File(refnum=w632, error in=w633) -> (error out=w626:errorcluster)  [unwired: 1 out]
                          n332 = call <vilib>:"Simple Error Handler.vi"("error in (no error)"=w626) -> ()  [unwired: 1 in, 8 out]
                        }
                      }
                    }
                    frame #2 {
                      n333 = property on="Contador" class="DigNum (strict)"() -> ("Value"=w649:i32)  [unwired: 2 in, 2 out]
                      n334 = Increment(x=w649) -> (x+1=w648:i32)
                      n335 = property on="N fit patamar" class="DigNum (strict)"() -> ("Value"=w641:i32)  [unwired: 2 in, 2 out]
                      n336 = Equal?(x=w648, y=w641) -> (x = y?=w650:bool)
                      n337 = case shown="True" w650 {
                        tunnel: [FALSE w655] -> w647
                        tunnel: [_ w654] -> w646
                        frame False {
                        }
                        frame True {
                          n338 = property on="P (bar/s)" class="DigNum (strict)"() -> ("Value"=w657:dbl)  [unwired: 2 in, 2 out]
                          n339 = Absolute Value(x=w657) -> (abs(x)=w656:dbl)
                          n340 = Less Or Equal?(x=w656, y="STOP (bar/s)") -> (x <= y?=w655:bool)
                          n341 = case shown="True" w655 {
                            tunnel: [_ w659] -> w654
                            frame False {
                            }
                            frame True {
                              n342 = property on="teste slope" class="DigNum (strict)"() -> ("Value"=w660:i32)  [unwired: 2 in, 2 out]
                              n343 = local write "Estagio auto"(7 ("Estagio auto")) -> ()
                              n344 = Increment(x=w660) -> (x+1=w659:i32)
                              "teste slope" <- w659
                            }
                          }
                        }
                      }
                      n345 = Greater Or Equal?(x=w646, y="Ntest") -> (x >= y?=w644:bool)
                      n346 = And(x=w650, y=w644) -> (x .and. y?=w643:bool)
                      n347 = case shown="True" w643 {
                        tunnel: [TRUE ("Boolean") FALSE ("Boolean")] -> w642
                        frame False {
                        }
                        frame True {
                        }
                      }
                      n348 = case shown="True" w643 {
                        frame False {
                        }
                        frame True {
                          n349 = flat-sequence {
                            frame #0 {
                              n350 = property on="N fit 2" class="DigNum (strict)"() -> ("Value"=w694:i32)  [unwired: 2 in, 2 out]
                              n351 = Wait (ms)(milliseconds to wait=u32 500) -> ()  [unwired: 1 out]
                              n352 = local write "N fit"(w694) -> ()
                            }
                            frame #1 {
                              n353 = local write "Estagio auto"(8 ("Estagio auto")) -> ()
                            }
                          }
                        }
                      }
                      n354 = case shown="False" w647 {
                        tunnel: w642 -> [_ w678]
                        frame False {
                          w674 = T7 3 items=["no dialog", "OK message", "continue or stop message", "OK message + warnings", "continue/stop + warnings"] ("type of dialog (OK msg:1)")
                          w662 = TRUE ("Boolean")
                          n355 = call-poly <vilib>:"DAQmx Create Virtual Channel.vi"("lines"=tag "Dev1/port0/line3") -> ("task out"=w664:refnum<k21>, "error out"=w665:errorcluster)  [unwired: 13 in]
                          n356 = Wait (ms)(milliseconds to wait="patamar milliseconds to wait") -> ()  [unwired: 1 out]
                          n357 = local write "Câmara 2"(w662) -> ()
                          n358 = call <vilib>:"DAQmx Start Task.vi"("task/channels in"=w664, "error in"=w665) -> ("task out"=w666:refnum<k21>, "error out"=w667:errorcluster)  [unwired: 12 in]
                          n359 = call-poly <vilib>:"DAQmx Write.vi"("task/channels in"=w666, "data"=w662, "error in"=w667) -> ("task out"=w671:refnum<k21>, "error out"=w672:errorcluster)  [unwired: 10 in, 1 out]
                          n360 = case shown="True" w662 {
                            frame False {
                            }
                            frame True {
                              n361 = property on="Vol Ref 3" class="Slide (strict)"() -> ("Value"=w675:dbl)  [unwired: 2 in, 2 out]
                              n362 = local write "Camara 2"(w675) -> ()
                            }
                          }
                          n363 = call <vilib>:"DAQmx Stop Task.vi"("task/channels in"=w671, "error in"=w672) -> ("task out"=w669:refnum<k21>, "error out"=w668:errorcluster)  [unwired: 12 in]
                          n364 = call <vilib>:"DAQmx Clear Task.vi"("task in"=w669, "error in"=w668) -> ("error out"=w673:errorcluster)  [unwired: 13 in]
                          n365 = call <vilib>:"Simple Error Handler.vi"("type of dialog (OK msg:1)"=w674, "error in (no error)"=w673) -> ()  [unwired: 3 in, 5 out]
                        }
                        frame True {
                          n366 = flat-sequence {
                            tunnel: w678 -> [w679]
                            tunnel: [w679] -> w676
                            tunnel: [w680] -> w677
                            tunnel: w676 -> [w680]
                            tunnel: w677 -> [w681]
                            frame #0 {
                            }
                            frame #1 {
                            }
                            frame #2 {
                              w683 = T7 3 items=["no dialog", "OK message", "continue or stop message", "OK message + warnings", "continue/stop + warnings"] ("type of dialog (OK msg:1)")
                              n367 = local write "Câmara 2"(w681) -> ()
                              n368 = call-poly <vilib>:"DAQmx Create Virtual Channel.vi"("lines"=tag "Dev1/port0/line3") -> ("task out"=w692:refnum<k21>, "error out"=w691:errorcluster)  [unwired: 13 in]
                              n369 = call <vilib>:"DAQmx Start Task.vi"("task/channels in"=w692, "error in"=w691) -> ("task out"=w690:refnum<k21>, "error out"=w689:errorcluster)  [unwired: 12 in]
                              n370 = call-poly <vilib>:"DAQmx Write.vi"("task/channels in"=w690, "data"=w681, "error in"=w689) -> ("task out"=w685:refnum<k21>, "error out"=w684:errorcluster)  [unwired: 10 in, 1 out]
                              n371 = call <vilib>:"DAQmx Stop Task.vi"("task/channels in"=w685, "error in"=w684) -> ("task out"=w687:refnum<k21>, "error out"=w688:errorcluster)  [unwired: 12 in]
                              n372 = call <vilib>:"DAQmx Clear Task.vi"("task in"=w687, "error in"=w688) -> ("error out"=w682:errorcluster)  [unwired: 13 in]
                              n373 = call <vilib>:"Simple Error Handler.vi"("type of dialog (OK msg:1)"=w683, "error in (no error)"=w682) -> ()  [unwired: 3 in, 5 out]
                            }
                            frame #3 {
                              n374 = Wait (ms)(milliseconds to wait=u32 2000) -> ()  [unwired: 1 out]
                            }
                          }
                        }
                      }
                    }
                  }
                }
                frame 8 {
                  n375 = property on="Contador" class="DigNum (strict)"() -> ("Value"=w723:i32)  [unwired: 2 in, 2 out]
                  n376 = Increment(x=w723) -> (x+1=w724:i32)
                  n377 = property on="N fit 2" class="DigNum (strict)"() -> ("Value"=w697:i32)  [unwired: 2 in, 2 out]
                  n378 = Equal?(x=w724, y=w697) -> (x = y?=w722:bool)
                  n379 = case shown="False" w721 {
                    tunnel: [FALSE ("Save manual") w1414] -> w701
                    tunnel: w722 -> [_ w1414]
                    frame False {
                    }
                    frame True {
                    }
                  }
                  n380 = case shown="True" w722 {
                    tunnel: w725 -> [_ w1415]
                    frame False {
                    }
                    frame True {
                      n381 = property on="P fit" class="DigNum (strict)"() -> ("Value"=w1416:dbl)  [unwired: 2 in, 2 out]
                      n382 = Number To Fractional String(number=w1416, precision (6)=i16 3) -> (F-format string=w1420:string)  [unwired: 2 in]
                      n383 = Concatenate Strings(w1420, "\t") -> (w1418:string)
                      n384 = flat-sequence {
                        tunnel: [w1427] -> w1422
                        tunnel: [w1426] -> w1421
                        tunnel: w1418 -> [w1425]
                        tunnel: w1415 -> [w1424]
                        tunnel: w1422 -> [w1442]
                        tunnel: w1421 -> [w1441]
                        frame #0 {
                          n385 = Wait (ms)(milliseconds to wait=u32 500) -> ()  [unwired: 1 out]
                          n386 = Open/Create/Replace File(file path (use dialog)=w1424, operation (0:open)=T3."open") -> (refnum out=w1433:refnum<file>, error out=w1434:errorcluster)  [unwired: 2 in, 3 out]
                          n387 = Set File Position(refnum=w1433, from (0:start)=enum16{"start", "end", "current"}."end", error in=w1434) -> (refnum out=w1431:refnum<file>, error out=w1430:errorcluster)  [unwired: 1 in]
                          n388 = Write to Text File(file (use dialog)=w1431, text=w1425, error in=w1430) -> (refnum out=w1435:refnum<file>, error out=w1436:errorcluster)  [unwired: 2 out]
                          n389 = Close File(refnum=w1435, error in=w1436) -> (path=w1427:path, error out=w1428:errorcluster)
                          n390 = call <vilib>:"Simple Error Handler.vi"("error in (no error)"=w1428) -> ("error out"=w1426:errorcluster)  [unwired: 1 in, 7 out]
                        }
                        frame #1 {
                          n391 = local write "Estagio auto"(9 ("Estagio auto")) -> ()
                          n392 = local write "Pf2 2"(TRUE ("ZPit")) -> ()
                          n393 = Wait (ms)(milliseconds to wait=u32 500) -> ()  [unwired: 1 out]
                          n394 = Read from Text File(file (use dialog)=w1442, count=-1 ("Count  3"), error in=w1441) -> (refnum out=w1443:refnum<file>, text=w1447:string, error out=w1444:errorcluster)  [unwired: 1 in, 1 out]
                          n395 = local write "String 3"(w1447) -> ()
                          n396 = Close File(refnum=w1443, error in=w1444) -> (error out=w1445:errorcluster)  [unwired: 1 out]
                          n397 = local write "String"("abrir valvula vacuo" ("String")) -> ()
                          n398 = call <vilib>:"Simple Error Handler.vi"("error in (no error)"=w1445) -> ()  [unwired: 1 in, 8 out]
                        }
                      }
                    }
                  }
                  n399 = flat-sequence {
                    tunnel: w701 -> [w727]
                    tunnel: w704 -> [w728]
                    tunnel: [w728] -> w699
                    tunnel: [w727] -> w698
                    tunnel: [w730] -> w720
                    tunnel: [w732] -> w719
                    tunnel: [w733] -> w718
                    tunnel: [w734] -> w717
                    tunnel: [w735] -> w716
                    tunnel: [w736] -> w715
                    tunnel: [w737] -> w714
                    tunnel: [w738] -> w713
                    tunnel: [w739] -> w712
                    tunnel: [w740] -> w711
                    tunnel: [w741] -> w710
                    tunnel: [w742] -> w709
                    tunnel: [w743] -> w708
                    tunnel: [w744] -> w707
                    tunnel: [w745] -> w706
                    tunnel: [w731] -> w705
                    tunnel: [w729] -> w702
                    tunnel: w699 -> [w747]
                    tunnel: w698 -> [w746]
                    tunnel: w720 -> [w1364]
                    tunnel: w719 -> [w1363]
                    tunnel: w718 -> [w1362]
                    tunnel: w717 -> [w1361]
                    tunnel: w716 -> [w1360]
                    tunnel: w715 -> [w1359]
                    tunnel: w714 -> [w1358]
                    tunnel: w713 -> [w1357]
                    tunnel: w712 -> [w1356]
                    tunnel: w711 -> [w1355]
                    tunnel: w710 -> [w1354]
                    tunnel: w709 -> [w1353]
                    tunnel: w708 -> [w1352]
                    tunnel: w707 -> [w1351]
                    tunnel: w706 -> [w1350]
                    tunnel: w705 -> [w1349]
                    tunnel: [w1347] -> w703
                    tunnel: w702 -> [w1347]
                    tunnel: [TRUE ("graph RLC")] -> w700
                    frame #0 {
                      n400 = local write "graph RLC"(FALSE) -> ()
                    }
                    frame #1 {
                      n401 = case shown="True" w746 {
                        tunnel: [FALSE w784] -> w729
                        tunnel: w747 -> [_ w766]
                        tunnel: [_ w764] -> w730
                        tunnel: [_ w763] -> w731
                        tunnel: [_ w762] -> w732
                        tunnel: [_ w761] -> w733
                        tunnel: [_ w760] -> w734
                        tunnel: [_ w759] -> w735
                        tunnel: [_ w758] -> w736
                        tunnel: [_ w757] -> w737
                        tunnel: [_ w756] -> w738
                        tunnel: [_ w755] -> w739
                        tunnel: [_ w754] -> w740
                        tunnel: [_ w753] -> w741
                        tunnel: [_ w752] -> w742
                        tunnel: [_ w751] -> w743
                        tunnel: [_ w750] -> w744
                        tunnel: [_ w749] -> w745
                        frame False {
                        }
                        frame True {
                          n402 = property on="path RLC_completo" class="Path"() -> ("Value"=w765:path)  [unwired: 2 in, 2 out]
                          n403 = for {
                            N: 5 -> [_]
                            tunnel: TRUE -> [w807]
                            tunnel: FALSE -> [w806]
                            tunnel: [w805] -> w784
                            tunnel: [w804] -> w782 mode=indexing
                            tunnel: [w803] -> w781 mode=indexing
                            tunnel: [w802] -> w780 mode=indexing
                            tunnel: [w801] -> w779 mode=indexing
                            tunnel: [w800] -> w778 mode=indexing
                            tunnel: [w799] -> w777 mode=indexing
                            tunnel: [w798] -> w776 mode=indexing
                            tunnel: [w797] -> w775 mode=indexing
                            tunnel: [w796] -> w774 mode=indexing
                            tunnel: [w795] -> w773 mode=indexing
                            tunnel: [w794] -> w772 mode=indexing
                            tunnel: [w793] -> w771 mode=indexing
                            tunnel: [w792] -> w770 mode=indexing
                            tunnel: [w791] -> w769 mode=indexing
                            tunnel: [w790] -> w768 mode=indexing
                            tunnel: [w789] -> w767 mode=indexing
                            tunnel: w766 -> [w788]
                            tunnel: w765 -> [w787]
                            n404 = stacked-sequence {
                              tunnel: w807 -> [_ w834 w868 w900 w932 w964 w996 w1028 w1060 w1092 w1124 w1156 w1188 w1220 w1252 w1284 w1316 _]
                              tunnel: w806 -> [w829 _ _ _ _ _ _ _ _ _ _ _ _ _ _ _ _ w1346]
                              tunnel: [_ _ _ _ _ _ _ _ _ _ _ _ _ _ _ _ _ TRUE] -> w805
                              tunnel: [_ w833 _ _ _ _ _ _ _ _ _ _ _ _ _ _ _ _] -> w804
                              tunnel: [_ _ w867 _ _ _ _ _ _ _ _ _ _ _ _ _ _ _] -> w803
                              tunnel: [_ _ _ w899 _ _ _ _ _ _ _ _ _ _ _ _ _ _] -> w802
                              tunnel: [_ _ _ _ w931 _ _ _ _ _ _ _ _ _ _ _ _ _] -> w801
                              tunnel: [_ _ _ _ _ w963 _ _ _ _ _ _ _ _ _ _ _ _] -> w800
                              tunnel: [_ _ _ _ _ _ w995 _ _ _ _ _ _ _ _ _ _ _] -> w799
                              tunnel: [_ _ _ _ _ _ _ w1027 _ _ _ _ _ _ _ _ _ _] -> w798
                              tunnel: [_ _ _ _ _ _ _ _ w1059 _ _ _ _ _ _ _ _ _] -> w797
                              tunnel: [_ _ _ _ _ _ _ _ _ w1091 _ _ _ _ _ _ _ _] -> w796
                              tunnel: [_ _ _ _ _ _ _ _ _ _ w1123 _ _ _ _ _ _ _] -> w795
                              tunnel: [_ _ _ _ _ _ _ _ _ _ _ w1155 _ _ _ _ _ _] -> w794
                              tunnel: [_ _ _ _ _ _ _ _ _ _ _ _ w1187 _ _ _ _ _] -> w793
                              tunnel: [_ _ _ _ _ _ _ _ _ _ _ _ _ w1219 _ _ _ _] -> w792
                              tunnel: [_ _ _ _ _ _ _ _ _ _ _ _ _ _ w1251 _ _ _] -> w791
                              tunnel: [_ _ _ _ _ _ _ _ _ _ _ _ _ _ _ w1283 _ _] -> w790
                              tunnel: [_ _ _ _ _ _ _ _ _ _ _ _ _ _ _ _ w1315 _] -> w789
                              tunnel: w788 -> [_ w832 w866 w898 w930 w962 w994 w1026 w1058 w1090 w1122 w1154 w1186 w1218 w1250 w1282 w1314 _]
                              tunnel: w787 -> [w808 w831 w865 w897 w929 w961 w993 w1025 w1057 w1089 w1121 w1153 w1185 w1217 w1249 w1281 w1313 _]
                              frame #0 {
                                w809 = "\t"
                                n405 = local write "C-50-L"(w829) -> ()
                                n406 = local write "C-50-N"(w829) -> ()
                                n407 = local write "Z-50-L"(w829) -> ()
                                n408 = local write "C-1K-N"(w829) -> ()
                                n409 = local write "C-1K-L"(w829) -> ()
                                n410 = local write "Z-50-N"(w829) -> ()
                                n411 = local write "Z-1K-N"(w829) -> ()
                                n412 = local write "Z-1K-L"(w829) -> ()
                                n413 = local write "C-10K-L"(w829) -> ()
                                n414 = local write "C-100-N"(w829) -> ()
                                n415 = local write "C-10K-N"(w829) -> ()
                                n416 = local write "Z-100-L"(w829) -> ()
                                n417 = local write "Z-10K-L"(w829) -> ()
                                n418 = local write "Z-100-N"(w829) -> ()
                                n419 = local write "Z-10K-N"(w829) -> ()
                                n420 = local write "C-100-L"(w829) -> ()
                                n421 = Open/Create/Replace File(file path (use dialog)=w808, operation (0:open)=T3."open") -> (refnum out=w823:refnum<file>, error out=w822:errorcluster)  [unwired: 2 in, 3 out]
                                n422 = Get Date/Time String(date format (0)=enum16{"short", "long", "abbreviated"}."short", want seconds? (F)=TRUE) -> (date string=w815:string, time string=w814:string)  [unwired: 1 in]
                                n423 = feedback #1() -> (w813:dbl)  [unwired: 1 in]
                                "SET 2" <- w813
                                n424 = Set File Position(refnum=w823, from (0:start)=enum16{"start", "end", "current"}."end", error in=w822) -> (refnum out=w825:refnum<file>, error out=w826:errorcluster)  [unwired: 1 in]
                                n425 = Number To Fractional String(number=w813, precision (6)=i16 2) -> (F-format string=w812:string)  [unwired: 2 in]
                                n426 = Add(x=w813, y=0.2) -> (x+y=w819:dbl)
                                n427 = feedback-in #1(w819) -> ()
                                n428 = Concatenate Strings(w812, w809, w815, w809, w814, w809) -> (w811:string)
                                n429 = Write to Text File(file (use dialog)=w825, text=w811, error in=w826) -> (refnum out=w821:refnum<file>, error out=w820:errorcluster)  [unwired: 1 in, 1 out]
                                n430 = Close File(refnum=w821, error in=w820) -> (error out=w828:errorcluster)  [unwired: 1 out]
                                n431 = call <vilib>:"Simple Error Handler.vi"("error in (no error)"=w828) -> ()  [unwired: 1 in, 8 out]
                              }
                              frame #1 {
                                n432 = case shown="False" "C50L" {
                                tunnel: w834 -> [_ w861]
                                tunnel: [0.0 ("MEASURE A") w841] -> w833
                                tunnel: w832 -> [_ w840]
                                tunnel: w831 -> [_ w836]
                                frame False {
                                }
                                frame True {
                                w842 = "\t"
                                w860 = i16 4 ("width (-)")
                                n433 = Open/Create/Replace File(file path (use dialog)=w836, operation (0:open)=T3."open") -> (refnum out=w851:refnum<file>, error out=w850:errorcluster)  [unwired: 2 in, 3 out]
                                n434 = Multiply(x="Time RLC", y=u32 1000) -> (x*y=w839:u32)
                                n435 = Wait (ms)(milliseconds to wait=w839) -> ()  [unwired: 1 out]
                                n436 = Set File Position(refnum=w851, from (0:start)=enum16{"start", "end", "current"}."end", error in=w850) -> (refnum out=w853:refnum<file>, error out=w854:errorcluster)  [unwired: 1 in]
                                n437 = call "RLC_read.vi"("Path"=w840, "String"="cmd /c rlc_read_cAL.py") -> ("MEASURE A"=w841:dbl, "MEASURE V [V]"=w858:dbl, "concatenated string"=w862:string, "MEASURE B"=w859:dbl, "MEASURE I [A]"=w857:dbl)  [unwired: 1 out]
                                "MEASURE A" <- w841
                                "MEASURE B" <- w859
                                n438 = Number To Engineering String(2:w860, 4:w857) -> (0:w843:string)  [unwired: 2 in]
                                n439 = local write "RLC300 - digimess"(w862) -> ()
                                n440 = Number To Engineering String(2:w860, 4:w858) -> (0:w844:string)  [unwired: 2 in]
                                n441 = Number To Engineering String(2:w860, 4:w841) -> (0:w846:string)  [unwired: 2 in]
                                n442 = Number To Engineering String(2:w860, 4:w859) -> (0:w845:string)  [unwired: 2 in]
                                n443 = Concatenate Strings(w846, w842, w845, w842, w844, w842, w843, w842) -> (w847:string)
                                n444 = Write to Text File(file (use dialog)=w853, text=w847, error in=w854) -> (refnum out=w849:refnum<file>, error out=w848:errorcluster)  [unwired: 1 in, 1 out]
                                n445 = Close File(refnum=w849, error in=w848) -> (error out=w856:errorcluster)  [unwired: 1 out]
                                n446 = call <vilib>:"Simple Error Handler.vi"("error in (no error)"=w856) -> ()  [unwired: 1 in, 8 out]
                                "C-50-L" <- w861
                                }
                                }
                              }
                              frame #2 {
                                n447 = case shown="False" "C50N" {
                                tunnel: w868 -> [_ w893]
                                tunnel: [0.0 ("MEASURE A") w873] -> w867
                                tunnel: w866 -> [_ w872]
                                tunnel: w865 -> [_ w870]
                                frame False {
                                }
                                frame True {
                                w877 = "\t"
                                w892 = i16 4 ("width (-)")
                                n448 = property on="Time RLC" class="DigNum (strict)"() -> ("Value"=w871:u32)  [unwired: 2 in, 2 out]
                                n449 = Wait (ms)(milliseconds to wait=w871) -> ()  [unwired: 1 out]
                                n450 = Open/Create/Replace File(file path (use dialog)=w870, operation (0:open)=T3."open") -> (refnum out=w886:refnum<file>, error out=w885:errorcluster)  [unwired: 2 in, 3 out]
                                n451 = Set File Position(refnum=w886, from (0:start)=enum16{"start", "end", "current"}."end", error in=w885) -> (refnum out=w888:refnum<file>, error out=w889:errorcluster)  [unwired: 1 in]
                                n452 = call "RLC_read.vi"("Path"=w872, "String"="cmd /c rlc_read_cAN.py") -> ("MEASURE A"=w873:dbl, "MEASURE V [V]"=w875:dbl, "concatenated string"=w895:string, "MEASURE B"=w876:dbl, "MEASURE I [A]"=w874:dbl)  [unwired: 1 out]
                                "MEASURE A 2" <- w873
                                "MEASURE B 2" <- w876
                                n453 = Number To Engineering String(2:w892, 4:w874) -> (0:w878:string)  [unwired: 2 in]
                                n454 = local write "RLC300 - digimess"(w895) -> ()
                                n455 = Number To Engineering String(2:w892, 4:w875) -> (0:w879:string)  [unwired: 2 in]
                                n456 = Number To Engineering String(2:w892, 4:w873) -> (0:w881:string)  [unwired: 2 in]
                                n457 = Number To Engineering String(2:w892, 4:w876) -> (0:w880:string)  [unwired: 2 in]
                                n458 = Concatenate Strings(w881, w877, w880, w877, w879, w877, w878, w877) -> (w882:string)
                                n459 = Write to Text File(file (use dialog)=w888, text=w882, error in=w889) -> (refnum out=w884:refnum<file>, error out=w883:errorcluster)  [unwired: 1 in, 1 out]
                                n460 = Close File(refnum=w884, error in=w883) -> (error out=w891:errorcluster)  [unwired: 1 out]
                                n461 = call <vilib>:"Simple Error Handler.vi"("error in (no error)"=w891) -> ()  [unwired: 1 in, 8 out]
                                "C-50-N" <- w893
                                }
                                }
                              }
                              frame #3 {
                                n462 = case shown="False" "C100L" {
                                tunnel: w900 -> [_ w926]
                                tunnel: [0.0 ("MEASURE A") w905] -> w899
                                tunnel: w898 -> [_ w904]
                                tunnel: w897 -> [_ w902]
                                frame False {
                                }
                                frame True {
                                w909 = "\t"
                                w924 = i16 4 ("width (-)")
                                n463 = property on="Time RLC" class="DigNum (strict)"() -> ("Value"=w903:u32)  [unwired: 2 in, 2 out]
                                n464 = Wait (ms)(milliseconds to wait=w903) -> ()  [unwired: 1 out]
                                n465 = Open/Create/Replace File(file path (use dialog)=w902, operation (0:open)=T3."open") -> (refnum out=w918:refnum<file>, error out=w917:errorcluster)  [unwired: 2 in, 3 out]
                                n466 = Set File Position(refnum=w918, from (0:start)=enum16{"start", "end", "current"}."end", error in=w917) -> (refnum out=w920:refnum<file>, error out=w921:errorcluster)  [unwired: 1 in]
                                n467 = call "RLC_read.vi"("Path"=w904, "String"="cmd /c rlc_read_cBL.py") -> ("MEASURE A"=w905:dbl, "MEASURE V [V]"=w907:dbl, "concatenated string"=w927:string, "MEASURE B"=w908:dbl, "MEASURE I [A]"=w906:dbl)  [unwired: 1 out]
                                "MEASURE A 3" <- w905
                                "MEASURE B 3" <- w908
                                n468 = Number To Engineering String(2:w924, 4:w906) -> (0:w910:string)  [unwired: 2 in]
                                n469 = local write "RLC300 - digimess"(w927) -> ()
                                n470 = Number To Engineering String(2:w924, 4:w907) -> (0:w911:string)  [unwired: 2 in]
                                n471 = Number To Engineering String(2:w924, 4:w905) -> (0:w913:string)  [unwired: 2 in]
                                n472 = Number To Engineering String(2:w924, 4:w908) -> (0:w912:string)  [unwired: 2 in]
                                n473 = Concatenate Strings(w913, w909, w912, w909, w911, w909, w910, w909) -> (w914:string)
                                n474 = Write to Text File(file (use dialog)=w920, text=w914, error in=w921) -> (refnum out=w916:refnum<file>, error out=w915:errorcluster)  [unwired: 1 in, 1 out]
                                n475 = Close File(refnum=w916, error in=w915) -> (error out=w923:errorcluster)  [unwired: 1 out]
                                n476 = call <vilib>:"Simple Error Handler.vi"("error in (no error)"=w923) -> ()  [unwired: 1 in, 8 out]
                                "C-100-L" <- w926
                                }
                                }
                              }
                              frame #4 {
                                n477 = case shown="False" "C100N" {
                                tunnel: w932 -> [_ w957]
                                tunnel: [0.0 ("MEASURE A") w937] -> w931
                                tunnel: w930 -> [_ w936]
                                tunnel: w929 -> [_ w934]
                                frame False {
                                }
                                frame True {
                                w941 = "\t"
                                w956 = i16 4 ("width (-)")
                                n478 = property on="Time RLC" class="DigNum (strict)"() -> ("Value"=w935:u32)  [unwired: 2 in, 2 out]
                                n479 = Wait (ms)(milliseconds to wait=w935) -> ()  [unwired: 1 out]
                                n480 = Open/Create/Replace File(file path (use dialog)=w934, operation (0:open)=T3."open") -> (refnum out=w950:refnum<file>, error out=w949:errorcluster)  [unwired: 2 in, 3 out]
                                n481 = Set File Position(refnum=w950, from (0:start)=enum16{"start", "end", "current"}."end", error in=w949) -> (refnum out=w952:refnum<file>, error out=w953:errorcluster)  [unwired: 1 in]
                                n482 = call "RLC_read.vi"("Path"=w936, "String"="cmd /c rlc_read_cBN.py") -> ("MEASURE A"=w937:dbl, "MEASURE V [V]"=w939:dbl, "concatenated string"=w959:string, "MEASURE B"=w940:dbl, "MEASURE I [A]"=w938:dbl)  [unwired: 1 out]
                                "MEASURE A 4" <- w937
                                "MEASURE B 4" <- w940
                                n483 = Number To Engineering String(2:w956, 4:w938) -> (0:w942:string)  [unwired: 2 in]
                                n484 = local write "RLC300 - digimess"(w959) -> ()
                                n485 = Number To Engineering String(2:w956, 4:w939) -> (0:w943:string)  [unwired: 2 in]
                                n486 = Number To Engineering String(2:w956, 4:w937) -> (0:w945:string)  [unwired: 2 in]
                                n487 = Number To Engineering String(2:w956, 4:w940) -> (0:w944:string)  [unwired: 2 in]
                                n488 = Concatenate Strings(w945, w941, w944, w941, w943, w941, w942, w941) -> (w946:string)
                                n489 = Write to Text File(file (use dialog)=w952, text=w946, error in=w953) -> (refnum out=w948:refnum<file>, error out=w947:errorcluster)  [unwired: 1 in, 1 out]
                                n490 = Close File(refnum=w948, error in=w947) -> (error out=w955:errorcluster)  [unwired: 1 out]
                                n491 = call <vilib>:"Simple Error Handler.vi"("error in (no error)"=w955) -> ()  [unwired: 1 in, 8 out]
                                "C-100-N" <- w957
                                }
                                }
                              }
                              frame #5 {
                                n492 = case shown="False" "C1KL" {
                                tunnel: w964 -> [_ w990]
                                tunnel: [0.0 ("MEASURE A") w969] -> w963
                                tunnel: w962 -> [_ w968]
                                tunnel: w961 -> [_ w966]
                                frame False {
                                }
                                frame True {
                                w988 = "\t"
                                w973 = i16 4 ("width (-)")
                                n493 = property on="Time RLC" class="DigNum (strict)"() -> ("Value"=w967:u32)  [unwired: 2 in, 2 out]
                                n494 = Wait (ms)(milliseconds to wait=w967) -> ()  [unwired: 1 out]
                                n495 = Open/Create/Replace File(file path (use dialog)=w966, operation (0:open)=T3."open") -> (refnum out=w979:refnum<file>, error out=w980:errorcluster)  [unwired: 2 in, 3 out]
                                n496 = Set File Position(refnum=w979, from (0:start)=enum16{"start", "end", "current"}."end", error in=w980) -> (refnum out=w977:refnum<file>, error out=w976:errorcluster)  [unwired: 1 in]
                                n497 = call "RLC_read.vi"("Path"=w968, "String"="cmd /c rlc_read_cCL.py") -> ("MEASURE A"=w969:dbl, "MEASURE V [V]"=w971:dbl, "concatenated string"=w991:string, "MEASURE B"=w972:dbl, "MEASURE I [A]"=w970:dbl)  [unwired: 1 out]
                                "MEASURE A 5" <- w969
                                "MEASURE B 5" <- w972
                                n498 = Number To Engineering String(2:w973, 4:w970) -> (0:w987:string)  [unwired: 2 in]
                                n499 = local write "RLC300 - digimess"(w991) -> ()
                                n500 = Number To Engineering String(2:w973, 4:w971) -> (0:w986:string)  [unwired: 2 in]
                                n501 = Number To Engineering String(2:w973, 4:w969) -> (0:w984:string)  [unwired: 2 in]
                                n502 = Number To Engineering String(2:w973, 4:w972) -> (0:w985:string)  [unwired: 2 in]
                                n503 = Concatenate Strings(w984, w988, w985, w988, w986, w988, w987, w988) -> (w983:string)
                                n504 = Write to Text File(file (use dialog)=w977, text=w983, error in=w976) -> (refnum out=w981:refnum<file>, error out=w982:errorcluster)  [unwired: 1 in, 1 out]
                                n505 = Close File(refnum=w981, error in=w982) -> (error out=w974:errorcluster)  [unwired: 1 out]
                                n506 = call <vilib>:"Simple Error Handler.vi"("error in (no error)"=w974) -> ()  [unwired: 1 in, 8 out]
                                "C-1K-L" <- w990
                                }
                                }
                              }
                              frame #6 {
                                n507 = case shown="True" "C1KN" {
                                tunnel: w996 -> [_ w1021]
                                tunnel: [0.0 ("MEASURE A") w1001] -> w995
                                tunnel: w994 -> [_ w1000]
                                tunnel: w993 -> [_ w998]
                                frame False {
                                }
                                frame True {
                                w1020 = "\t"
                                w1005 = i16 4 ("width (-)")
                                n508 = property on="Time RLC" class="DigNum (strict)"() -> ("Value"=w999:u32)  [unwired: 2 in, 2 out]
                                n509 = Wait (ms)(milliseconds to wait=w999) -> ()  [unwired: 1 out]
                                n510 = Open/Create/Replace File(file path (use dialog)=w998, operation (0:open)=T3."open") -> (refnum out=w1011:refnum<file>, error out=w1012:errorcluster)  [unwired: 2 in, 3 out]
                                n511 = Set File Position(refnum=w1011, from (0:start)=enum16{"start", "end", "current"}."end", error in=w1012) -> (refnum out=w1009:refnum<file>, error out=w1008:errorcluster)  [unwired: 1 in]
                                n512 = call "RLC_read.vi"("Path"=w1000, "String"="cmd /c rlc_read_cCN.py") -> ("MEASURE A"=w1001:dbl, "MEASURE V [V]"=w1003:dbl, "concatenated string"=w1023:string, "MEASURE B"=w1004:dbl, "MEASURE I [A]"=w1002:dbl)  [unwired: 1 out]
                                "MEASURE A 6" <- w1001
                                "MEASURE B 6" <- w1004
                                n513 = Number To Engineering String(2:w1005, 4:w1002) -> (0:w1019:string)  [unwired: 2 in]
                                n514 = local write "RLC300 - digimess"(w1023) -> ()
                                n515 = Number To Engineering String(2:w1005, 4:w1003) -> (0:w1018:string)  [unwired: 2 in]
                                n516 = Number To Engineering String(2:w1005, 4:w1001) -> (0:w1016:string)  [unwired: 2 in]
                                n517 = Number To Engineering String(2:w1005, 4:w1004) -> (0:w1017:string)  [unwired: 2 in]
                                n518 = Concatenate Strings(w1016, w1020, w1017, w1020, w1018, w1020, w1019, w1020) -> (w1015:string)
                                n519 = Write to Text File(file (use dialog)=w1009, text=w1015, error in=w1008) -> (refnum out=w1013:refnum<file>, error out=w1014:errorcluster)  [unwired: 1 in, 1 out]
                                n520 = Close File(refnum=w1013, error in=w1014) -> (error out=w1006:errorcluster)  [unwired: 1 out]
                                n521 = call <vilib>:"Simple Error Handler.vi"("error in (no error)"=w1006) -> ()  [unwired: 1 in, 8 out]
                                "C-1K-N" <- w1021
                                }
                                }
                              }
                              frame #7 {
                                n522 = case shown="False" "C10KL" {
                                tunnel: w1028 -> [_ w1054]
                                tunnel: [0.0 ("MEASURE A") w1033] -> w1027
                                tunnel: w1026 -> [_ w1032]
                                tunnel: w1025 -> [_ w1030]
                                frame False {
                                }
                                frame True {
                                w1037 = "\t"
                                w1052 = i16 4 ("width (-)")
                                n523 = property on="Time RLC" class="DigNum (strict)"() -> ("Value"=w1031:u32)  [unwired: 2 in, 2 out]
                                n524 = Wait (ms)(milliseconds to wait=w1031) -> ()  [unwired: 1 out]
                                n525 = Open/Create/Replace File(file path (use dialog)=w1030, operation (0:open)=T3."open") -> (refnum out=w1046:refnum<file>, error out=w1045:errorcluster)  [unwired: 2 in, 3 out]
                                n526 = Set File Position(refnum=w1046, from (0:start)=enum16{"start", "end", "current"}."end", error in=w1045) -> (refnum out=w1048:refnum<file>, error out=w1049:errorcluster)  [unwired: 1 in]
                                n527 = call "RLC_read.vi"("Path"=w1032, "String"="cmd /c rlc_read_cDL.py") -> ("MEASURE A"=w1033:dbl, "MEASURE V [V]"=w1035:dbl, "concatenated string"=w1055:string, "MEASURE B"=w1036:dbl, "MEASURE I [A]"=w1034:dbl)  [unwired: 1 out]
                                "MEASURE A 7" <- w1033
                                "MEASURE B 7" <- w1036
                                n528 = Number To Engineering String(2:w1052, 4:w1034) -> (0:w1038:string)  [unwired: 2 in]
                                n529 = local write "RLC300 - digimess"(w1055) -> ()
                                n530 = Number To Engineering String(2:w1052, 4:w1035) -> (0:w1039:string)  [unwired: 2 in]
                                n531 = Number To Engineering String(2:w1052, 4:w1033) -> (0:w1041:string)  [unwired: 2 in]
                                n532 = Number To Engineering String(2:w1052, 4:w1036) -> (0:w1040:string)  [unwired: 2 in]
                                n533 = Concatenate Strings(w1041, w1037, w1040, w1037, w1039, w1037, w1038, w1037) -> (w1042:string)
                                n534 = Write to Text File(file (use dialog)=w1048, text=w1042, error in=w1049) -> (refnum out=w1044:refnum<file>, error out=w1043:errorcluster)  [unwired: 1 in, 1 out]
                                n535 = Close File(refnum=w1044, error in=w1043) -> (error out=w1051:errorcluster)  [unwired: 1 out]
                                n536 = call <vilib>:"Simple Error Handler.vi"("error in (no error)"=w1051) -> ()  [unwired: 1 in, 8 out]
                                "C-10K-L" <- w1054
                                }
                                }
                              }
                              frame #8 {
                                n537 = case shown="False" "C10KN" {
                                tunnel: w1060 -> [_ w1086]
                                tunnel: [0.0 ("MEASURE A") w1065] -> w1059
                                tunnel: w1058 -> [_ w1064]
                                tunnel: w1057 -> [_ w1062]
                                frame False {
                                }
                                frame True {
                                w1069 = "\t"
                                w1084 = i16 4 ("width (-)")
                                n538 = property on="Time RLC" class="DigNum (strict)"() -> ("Value"=w1063:u32)  [unwired: 2 in, 2 out]
                                n539 = Wait (ms)(milliseconds to wait=w1063) -> ()  [unwired: 1 out]
                                n540 = Open/Create/Replace File(file path (use dialog)=w1062, operation (0:open)=T3."open") -> (refnum out=w1078:refnum<file>, error out=w1077:errorcluster)  [unwired: 2 in, 3 out]
                                n541 = Set File Position(refnum=w1078, from (0:start)=enum16{"start", "end", "current"}."end", error in=w1077) -> (refnum out=w1080:refnum<file>, error out=w1081:errorcluster)  [unwired: 1 in]
                                n542 = call "RLC_read.vi"("Path"=w1064, "String"="cmd /c rlc_read_cDN.py") -> ("MEASURE A"=w1065:dbl, "MEASURE V [V]"=w1067:dbl, "concatenated string"=w1087:string, "MEASURE B"=w1068:dbl, "MEASURE I [A]"=w1066:dbl)  [unwired: 1 out]
                                "MEASURE A 8" <- w1065
                                "MEASURE B 8" <- w1068
                                n543 = Number To Engineering String(2:w1084, 4:w1066) -> (0:w1070:string)  [unwired: 2 in]
                                n544 = local write "RLC300 - digimess"(w1087) -> ()
                                n545 = Number To Engineering String(2:w1084, 4:w1067) -> (0:w1071:string)  [unwired: 2 in]
                                n546 = Number To Engineering String(2:w1084, 4:w1065) -> (0:w1073:string)  [unwired: 2 in]
                                n547 = Number To Engineering String(2:w1084, 4:w1068) -> (0:w1072:string)  [unwired: 2 in]
                                n548 = Concatenate Strings(w1073, w1069, w1072, w1069, w1071, w1069, w1070, w1069) -> (w1074:string)
                                n549 = Write to Text File(file (use dialog)=w1080, text=w1074, error in=w1081) -> (refnum out=w1076:refnum<file>, error out=w1075:errorcluster)  [unwired: 1 in, 1 out]
                                n550 = Close File(refnum=w1076, error in=w1075) -> (error out=w1083:errorcluster)  [unwired: 1 out]
                                n551 = call <vilib>:"Simple Error Handler.vi"("error in (no error)"=w1083) -> ()  [unwired: 1 in, 8 out]
                                "C-10K-N" <- w1086
                                }
                                }
                              }
                              frame #9 {
                                n552 = case shown="False" "Z50L" {
                                tunnel: w1092 -> [_ w1117]
                                tunnel: [0.0 ("MEASURE A") w1097] -> w1091
                                tunnel: w1090 -> [_ w1096]
                                tunnel: w1089 -> [_ w1094]
                                frame False {
                                }
                                frame True {
                                w1101 = "\t"
                                w1116 = i16 4 ("width (-)")
                                n553 = property on="Time RLC" class="DigNum (strict)"() -> ("Value"=w1095:u32)  [unwired: 2 in, 2 out]
                                n554 = Wait (ms)(milliseconds to wait=w1095) -> ()  [unwired: 1 out]
                                n555 = Open/Create/Replace File(file path (use dialog)=w1094, operation (0:open)=T3."open") -> (refnum out=w1110:refnum<file>, error out=w1109:errorcluster)  [unwired: 2 in, 3 out]
                                n556 = Set File Position(refnum=w1110, from (0:start)=enum16{"start", "end", "current"}."end", error in=w1109) -> (refnum out=w1112:refnum<file>, error out=w1113:errorcluster)  [unwired: 1 in]
                                n557 = call "RLC_read.vi"("Path"=w1096, "String"="cmd /c rlc_read_ZAL.py") -> ("MEASURE A"=w1097:dbl, "MEASURE V [V]"=w1099:dbl, "concatenated string"=w1118:string, "MEASURE B"=w1100:dbl, "MEASURE I [A]"=w1098:dbl)  [unwired: 1 out]
                                "MEASURE A 9" <- w1097
                                "MEASURE B 9" <- w1100
                                n558 = Number To Engineering String(2:w1116, 4:w1098) -> (0:w1102:string)  [unwired: 2 in]
                                n559 = local write "RLC300 - digimess"(w1118) -> ()
                                n560 = Number To Engineering String(2:w1116, 4:w1099) -> (0:w1103:string)  [unwired: 2 in]
                                n561 = Number To Engineering String(2:w1116, 4:w1097) -> (0:w1105:string)  [unwired: 2 in]
                                n562 = Number To Engineering String(2:w1116, 4:w1100) -> (0:w1104:string)  [unwired: 2 in]
                                n563 = Concatenate Strings(w1105, w1101, w1104, w1101, w1103, w1101, w1102, w1101) -> (w1106:string)
                                n564 = Write to Text File(file (use dialog)=w1112, text=w1106, error in=w1113) -> (refnum out=w1108:refnum<file>, error out=w1107:errorcluster)  [unwired: 1 in, 1 out]
                                n565 = Close File(refnum=w1108, error in=w1107) -> (error out=w1115:errorcluster)  [unwired: 1 out]
                                n566 = call <vilib>:"Simple Error Handler.vi"("error in (no error)"=w1115) -> ()  [unwired: 1 in, 8 out]
                                "Z-50-L" <- w1117
                                }
                                }
                              }
                              frame #10 {
                                n567 = case shown="False" "Z50N" {
                                tunnel: w1124 -> [_ w1149]
                                tunnel: [0.0 ("MEASURE A") w1129] -> w1123
                                tunnel: w1122 -> [_ w1128]
                                tunnel: w1121 -> [_ w1126]
                                frame False {
                                }
                                frame True {
                                w1133 = "\t"
                                w1148 = i16 4 ("width (-)")
                                n568 = property on="Time RLC" class="DigNum (strict)"() -> ("Value"=w1127:u32)  [unwired: 2 in, 2 out]
                                n569 = Wait (ms)(milliseconds to wait=w1127) -> ()  [unwired: 1 out]
                                n570 = Open/Create/Replace File(file path (use dialog)=w1126, operation (0:open)=T3."open") -> (refnum out=w1142:refnum<file>, error out=w1141:errorcluster)  [unwired: 2 in, 3 out]
                                n571 = Set File Position(refnum=w1142, from (0:start)=enum16{"start", "end", "current"}."end", error in=w1141) -> (refnum out=w1144:refnum<file>, error out=w1145:errorcluster)  [unwired: 1 in]
                                n572 = call "RLC_read.vi"("Path"=w1128, "String"="cmd /c rlc_read_ZAN.py") -> ("MEASURE A"=w1129:dbl, "MEASURE V [V]"=w1131:dbl, "concatenated string"=w1150:string, "MEASURE B"=w1132:dbl, "MEASURE I [A]"=w1130:dbl)  [unwired: 1 out]
                                "MEASURE A 10" <- w1129
                                "MEASURE B 10" <- w1132
                                n573 = Number To Engineering String(2:w1148, 4:w1130) -> (0:w1134:string)  [unwired: 2 in]
                                n574 = local write "RLC300 - digimess"(w1150) -> ()
                                n575 = Number To Engineering String(2:w1148, 4:w1131) -> (0:w1135:string)  [unwired: 2 in]
                                n576 = Number To Engineering String(2:w1148, 4:w1129) -> (0:w1137:string)  [unwired: 2 in]
                                n577 = Number To Engineering String(2:w1148, 4:w1132) -> (0:w1136:string)  [unwired: 2 in]
                                n578 = Concatenate Strings(w1137, w1133, w1136, w1133, w1135, w1133, w1134, w1133) -> (w1138:string)
                                n579 = Write to Text File(file (use dialog)=w1144, text=w1138, error in=w1145) -> (refnum out=w1140:refnum<file>, error out=w1139:errorcluster)  [unwired: 1 in, 1 out]
                                n580 = Close File(refnum=w1140, error in=w1139) -> (error out=w1147:errorcluster)  [unwired: 1 out]
                                n581 = call <vilib>:"Simple Error Handler.vi"("error in (no error)"=w1147) -> ()  [unwired: 1 in, 8 out]
                                "Z-50-N" <- w1149
                                }
                                }
                              }
                              frame #11 {
                                n582 = case shown="False" "Z100L" {
                                tunnel: w1156 -> [_ w1181]
                                tunnel: [0.0 ("MEASURE A") w1161] -> w1155
                                tunnel: w1154 -> [_ w1160]
                                tunnel: w1153 -> [_ w1158]
                                frame False {
                                }
                                frame True {
                                w1165 = "\t"
                                w1180 = i16 4 ("width (-)")
                                n583 = property on="Time RLC" class="DigNum (strict)"() -> ("Value"=w1159:u32)  [unwired: 2 in, 2 out]
                                n584 = Wait (ms)(milliseconds to wait=w1159) -> ()  [unwired: 1 out]
                                n585 = Open/Create/Replace File(file path (use dialog)=w1158, operation (0:open)=T3."open") -> (refnum out=w1174:refnum<file>, error out=w1173:errorcluster)  [unwired: 2 in, 3 out]
                                n586 = Set File Position(refnum=w1174, from (0:start)=enum16{"start", "end", "current"}."end", error in=w1173) -> (refnum out=w1176:refnum<file>, error out=w1177:errorcluster)  [unwired: 1 in]
                                n587 = call "RLC_read.vi"("Path"=w1160, "String"="cmd /c rlc_read_ZBL.py") -> ("MEASURE A"=w1161:dbl, "MEASURE V [V]"=w1163:dbl, "concatenated string"=w1182:string, "MEASURE B"=w1164:dbl, "MEASURE I [A]"=w1162:dbl)  [unwired: 1 out]
                                "MEASURE A 11" <- w1161
                                "MEASURE B 11" <- w1164
                                n588 = Number To Engineering String(2:w1180, 4:w1162) -> (0:w1166:string)  [unwired: 2 in]
                                n589 = local write "RLC300 - digimess"(w1182) -> ()
                                n590 = Number To Engineering String(2:w1180, 4:w1163) -> (0:w1167:string)  [unwired: 2 in]
                                n591 = Number To Engineering String(2:w1180, 4:w1161) -> (0:w1169:string)  [unwired: 2 in]
                                n592 = Number To Engineering String(2:w1180, 4:w1164) -> (0:w1168:string)  [unwired: 2 in]
                                n593 = Concatenate Strings(w1169, w1165, w1168, w1165, w1167, w1165, w1166, w1165) -> (w1170:string)
                                n594 = Write to Text File(file (use dialog)=w1176, text=w1170, error in=w1177) -> (refnum out=w1172:refnum<file>, error out=w1171:errorcluster)  [unwired: 1 in, 1 out]
                                n595 = Close File(refnum=w1172, error in=w1171) -> (error out=w1179:errorcluster)  [unwired: 1 out]
                                n596 = call <vilib>:"Simple Error Handler.vi"("error in (no error)"=w1179) -> ()  [unwired: 1 in, 8 out]
                                "Z-100-L" <- w1181
                                }
                                }
                              }
                              frame #12 {
                                n597 = case shown="False" "Z100N" {
                                tunnel: w1188 -> [_ w1213]
                                tunnel: [0.0 ("MEASURE A") w1193] -> w1187
                                tunnel: w1186 -> [_ w1192]
                                tunnel: w1185 -> [_ w1190]
                                frame False {
                                }
                                frame True {
                                w1197 = "\t"
                                w1212 = i16 4 ("width (-)")
                                n598 = property on="Time RLC" class="DigNum (strict)"() -> ("Value"=w1191:u32)  [unwired: 2 in, 2 out]
                                n599 = Wait (ms)(milliseconds to wait=w1191) -> ()  [unwired: 1 out]
                                n600 = Open/Create/Replace File(file path (use dialog)=w1190, operation (0:open)=T3."open") -> (refnum out=w1206:refnum<file>, error out=w1205:errorcluster)  [unwired: 2 in, 3 out]
                                n601 = Set File Position(refnum=w1206, from (0:start)=enum16{"start", "end", "current"}."end", error in=w1205) -> (refnum out=w1208:refnum<file>, error out=w1209:errorcluster)  [unwired: 1 in]
                                n602 = call "RLC_read.vi"("Path"=w1192, "String"="cmd /c rlc_read_ZBN.py") -> ("MEASURE A"=w1193:dbl, "MEASURE V [V]"=w1195:dbl, "concatenated string"=w1214:string, "MEASURE B"=w1196:dbl, "MEASURE I [A]"=w1194:dbl)  [unwired: 1 out]
                                "MEASURE A 12" <- w1193
                                "MEASURE B 12" <- w1196
                                n603 = Number To Engineering String(2:w1212, 4:w1194) -> (0:w1198:string)  [unwired: 2 in]
                                n604 = local write "RLC300 - digimess"(w1214) -> ()
                                n605 = Number To Engineering String(2:w1212, 4:w1195) -> (0:w1199:string)  [unwired: 2 in]
                                n606 = Number To Engineering String(2:w1212, 4:w1193) -> (0:w1201:string)  [unwired: 2 in]
                                n607 = Number To Engineering String(2:w1212, 4:w1196) -> (0:w1200:string)  [unwired: 2 in]
                                n608 = Concatenate Strings(w1201, w1197, w1200, w1197, w1199, w1197, w1198, w1197) -> (w1202:string)
                                n609 = Write to Text File(file (use dialog)=w1208, text=w1202, error in=w1209) -> (refnum out=w1204:refnum<file>, error out=w1203:errorcluster)  [unwired: 1 in, 1 out]
                                n610 = Close File(refnum=w1204, error in=w1203) -> (error out=w1211:errorcluster)  [unwired: 1 out]
                                n611 = call <vilib>:"Simple Error Handler.vi"("error in (no error)"=w1211) -> ()  [unwired: 1 in, 8 out]
                                "Z-100-N" <- w1213
                                }
                                }
                              }
                              frame #13 {
                                n612 = case shown="False" "Z1KL" {
                                tunnel: w1220 -> [_ w1245]
                                tunnel: [0.0 ("MEASURE A") w1225] -> w1219
                                tunnel: w1218 -> [_ w1224]
                                tunnel: w1217 -> [_ w1222]
                                frame False {
                                }
                                frame True {
                                w1229 = "\t"
                                w1244 = i16 4 ("width (-)")
                                n613 = property on="Time RLC" class="DigNum (strict)"() -> ("Value"=w1223:u32)  [unwired: 2 in, 2 out]
                                n614 = Wait (ms)(milliseconds to wait=w1223) -> ()  [unwired: 1 out]
                                n615 = Open/Create/Replace File(file path (use dialog)=w1222, operation (0:open)=T3."open") -> (refnum out=w1238:refnum<file>, error out=w1237:errorcluster)  [unwired: 2 in, 3 out]
                                n616 = Set File Position(refnum=w1238, from (0:start)=enum16{"start", "end", "current"}."end", error in=w1237) -> (refnum out=w1240:refnum<file>, error out=w1241:errorcluster)  [unwired: 1 in]
                                n617 = call "RLC_read.vi"("Path"=w1224, "String"="cmd /c rlc_read_ZCL.py") -> ("MEASURE A"=w1225:dbl, "MEASURE V [V]"=w1227:dbl, "concatenated string"=w1246:string, "MEASURE B"=w1228:dbl, "MEASURE I [A]"=w1226:dbl)  [unwired: 1 out]
                                "MEASURE A 13" <- w1225
                                "MEASURE B 13" <- w1228
                                n618 = Number To Engineering String(2:w1244, 4:w1226) -> (0:w1230:string)  [unwired: 2 in]
                                n619 = local write "RLC300 - digimess"(w1246) -> ()
                                n620 = Number To Engineering String(2:w1244, 4:w1227) -> (0:w1231:string)  [unwired: 2 in]
                                n621 = Number To Engineering String(2:w1244, 4:w1225) -> (0:w1233:string)  [unwired: 2 in]
                                n622 = Number To Engineering String(2:w1244, 4:w1228) -> (0:w1232:string)  [unwired: 2 in]
                                n623 = Concatenate Strings(w1233, w1229, w1232, w1229, w1231, w1229, w1230, w1229) -> (w1234:string)
                                n624 = Write to Text File(file (use dialog)=w1240, text=w1234, error in=w1241) -> (refnum out=w1236:refnum<file>, error out=w1235:errorcluster)  [unwired: 1 in, 1 out]
                                n625 = Close File(refnum=w1236, error in=w1235) -> (error out=w1243:errorcluster)  [unwired: 1 out]
                                n626 = call <vilib>:"Simple Error Handler.vi"("error in (no error)"=w1243) -> ()  [unwired: 1 in, 8 out]
                                "Z-1K-L" <- w1245
                                }
                                }
                              }
                              frame #14 {
                                n627 = case shown="False" "Z1KN" {
                                tunnel: w1252 -> [_ w1277]
                                tunnel: [0.0 ("MEASURE A") w1257] -> w1251
                                tunnel: w1250 -> [_ w1256]
                                tunnel: w1249 -> [_ w1254]
                                frame False {
                                }
                                frame True {
                                w1261 = "\t"
                                w1276 = i16 4 ("width (-)")
                                n628 = property on="Time RLC" class="DigNum (strict)"() -> ("Value"=w1255:u32)  [unwired: 2 in, 2 out]
                                n629 = Wait (ms)(milliseconds to wait=w1255) -> ()  [unwired: 1 out]
                                n630 = Open/Create/Replace File(file path (use dialog)=w1254, operation (0:open)=T3."open") -> (refnum out=w1270:refnum<file>, error out=w1269:errorcluster)  [unwired: 2 in, 3 out]
                                n631 = Set File Position(refnum=w1270, from (0:start)=enum16{"start", "end", "current"}."end", error in=w1269) -> (refnum out=w1272:refnum<file>, error out=w1273:errorcluster)  [unwired: 1 in]
                                n632 = call "RLC_read.vi"("Path"=w1256, "String"="cmd /c rlc_read_ZCN.py") -> ("MEASURE A"=w1257:dbl, "MEASURE V [V]"=w1259:dbl, "concatenated string"=w1278:string, "MEASURE B"=w1260:dbl, "MEASURE I [A]"=w1258:dbl)  [unwired: 1 out]
                                "MEASURE A 14" <- w1257
                                "MEASURE B 14" <- w1260
                                n633 = Number To Engineering String(2:w1276, 4:w1258) -> (0:w1262:string)  [unwired: 2 in]
                                n634 = local write "RLC300 - digimess"(w1278) -> ()
                                n635 = Number To Engineering String(2:w1276, 4:w1259) -> (0:w1263:string)  [unwired: 2 in]
                                n636 = Number To Engineering String(2:w1276, 4:w1257) -> (0:w1265:string)  [unwired: 2 in]
                                n637 = Number To Engineering String(2:w1276, 4:w1260) -> (0:w1264:string)  [unwired: 2 in]
                                n638 = Concatenate Strings(w1265, w1261, w1264, w1261, w1263, w1261, w1262, w1261) -> (w1266:string)
                                n639 = Write to Text File(file (use dialog)=w1272, text=w1266, error in=w1273) -> (refnum out=w1268:refnum<file>, error out=w1267:errorcluster)  [unwired: 1 in, 1 out]
                                n640 = Close File(refnum=w1268, error in=w1267) -> (error out=w1275:errorcluster)  [unwired: 1 out]
                                n641 = call <vilib>:"Simple Error Handler.vi"("error in (no error)"=w1275) -> ()  [unwired: 1 in, 8 out]
                                "Z-1K-N" <- w1277
                                }
                                }
                              }
                              frame #15 {
                                n642 = case shown="False" "Z10KL" {
                                tunnel: w1284 -> [_ w1309]
                                tunnel: [0.0 ("MEASURE A") w1289] -> w1283
                                tunnel: w1282 -> [_ w1288]
                                tunnel: w1281 -> [_ w1286]
                                frame False {
                                }
                                frame True {
                                w1293 = "\t"
                                w1308 = i16 4 ("width (-)")
                                n643 = property on="Time RLC" class="DigNum (strict)"() -> ("Value"=w1287:u32)  [unwired: 2 in, 2 out]
                                n644 = Wait (ms)(milliseconds to wait=w1287) -> ()  [unwired: 1 out]
                                n645 = Open/Create/Replace File(file path (use dialog)=w1286, operation (0:open)=T3."open") -> (refnum out=w1302:refnum<file>, error out=w1301:errorcluster)  [unwired: 2 in, 3 out]
                                n646 = Set File Position(refnum=w1302, from (0:start)=enum16{"start", "end", "current"}."end", error in=w1301) -> (refnum out=w1304:refnum<file>, error out=w1305:errorcluster)  [unwired: 1 in]
                                n647 = call "RLC_read.vi"("Path"=w1288, "String"="cmd /c rlc_read_ZDL.py") -> ("MEASURE A"=w1289:dbl, "MEASURE V [V]"=w1291:dbl, "concatenated string"=w1310:string, "MEASURE B"=w1292:dbl, "MEASURE I [A]"=w1290:dbl)  [unwired: 1 out]
                                "MEASURE A 15" <- w1289
                                "MEASURE B 15" <- w1292
                                n648 = Number To Engineering String(2:w1308, 4:w1290) -> (0:w1294:string)  [unwired: 2 in]
                                n649 = local write "RLC300 - digimess"(w1310) -> ()
                                n650 = Number To Engineering String(2:w1308, 4:w1291) -> (0:w1295:string)  [unwired: 2 in]
                                n651 = Number To Engineering String(2:w1308, 4:w1289) -> (0:w1297:string)  [unwired: 2 in]
                                n652 = Number To Engineering String(2:w1308, 4:w1292) -> (0:w1296:string)  [unwired: 2 in]
                                n653 = Concatenate Strings(w1297, w1293, w1296, w1293, w1295, w1293, w1294, w1293) -> (w1298:string)
                                n654 = Write to Text File(file (use dialog)=w1304, text=w1298, error in=w1305) -> (refnum out=w1300:refnum<file>, error out=w1299:errorcluster)  [unwired: 1 in, 1 out]
                                n655 = Close File(refnum=w1300, error in=w1299) -> (error out=w1307:errorcluster)  [unwired: 1 out]
                                n656 = call <vilib>:"Simple Error Handler.vi"("error in (no error)"=w1307) -> ()  [unwired: 1 in, 8 out]
                                "Z-10K-L" <- w1309
                                }
                                }
                              }
                              frame #16 {
                                n657 = case shown="False" "Z10KN" {
                                tunnel: w1316 -> [_ w1342]
                                tunnel: [0.0 ("MEASURE A") w1321] -> w1315
                                tunnel: w1314 -> [_ w1320]
                                tunnel: w1313 -> [_ w1318]
                                frame False {
                                }
                                frame True {
                                w1326 = "\t"
                                w1341 = i16 4 ("width (-)")
                                n658 = property on="Time RLC" class="DigNum (strict)"() -> ("Value"=w1319:u32)  [unwired: 2 in, 2 out]
                                n659 = Wait (ms)(milliseconds to wait=w1319) -> ()  [unwired: 1 out]
                                n660 = Open/Create/Replace File(file path (use dialog)=w1318, operation (0:open)=T3."open") -> (refnum out=w1335:refnum<file>, error out=w1334:errorcluster)  [unwired: 2 in, 3 out]
                                n661 = Set File Position(refnum=w1335, from (0:start)=enum16{"start", "end", "current"}."end", error in=w1334) -> (refnum out=w1337:refnum<file>, error out=w1338:errorcluster)  [unwired: 1 in]
                                n662 = call "RLC_read.vi"("Path"=w1320, "String"="cmd /c rlc_read_ZDN.py") -> ("MEASURE A"=w1321:dbl, "MEASURE V [V]"=w1324:dbl, "concatenated string"=w1343:string, "MEASURE B"=w1325:dbl, "MEASURE I [A]"=w1323:dbl)  [unwired: 1 out]
                                "MEASURE A 16" <- w1321
                                "MEASURE B 16" <- w1325
                                n663 = Number To Engineering String(2:w1341, 4:w1323) -> (0:w1327:string)  [unwired: 2 in]
                                n664 = local write "RLC300 - digimess"(w1343) -> ()
                                n665 = Number To Engineering String(2:w1341, 4:w1324) -> (0:w1328:string)  [unwired: 2 in]
                                n666 = Number To Engineering String(2:w1341, 4:w1321) -> (0:w1330:string)  [unwired: 2 in]
                                n667 = Number To Engineering String(2:w1341, 4:w1325) -> (0:w1329:string)  [unwired: 2 in]
                                n668 = Concatenate Strings(w1330, w1326, w1329, w1326, w1328, w1326, w1327, w1326, "\r\n") -> (w1331:string)
                                n669 = Write to Text File(file (use dialog)=w1337, text=w1331, error in=w1338) -> (refnum out=w1333:refnum<file>, error out=w1332:errorcluster)  [unwired: 1 in, 1 out]
                                n670 = Close File(refnum=w1333, error in=w1332) -> (error out=w1340:errorcluster)  [unwired: 1 out]
                                n671 = call <vilib>:"Simple Error Handler.vi"("error in (no error)"=w1340) -> ()  [unwired: 1 in, 8 out]
                                "Z-10K-N" <- w1342
                                }
                                }
                              }
                              frame #17 {
                                n672 = local write "Z-50-L"(w1346) -> ()
                                n673 = local write "Z-1K-L"(w1346) -> ()
                                n674 = local write "Z-1K-N"(w1346) -> ()
                                n675 = local write "C-50-N"(w1346) -> ()
                                n676 = local write "C-50-L"(w1346) -> ()
                                n677 = local write "Z-50-N"(w1346) -> ()
                                n678 = local write "C-1K-N"(w1346) -> ()
                                n679 = local write "C-1K-L"(w1346) -> ()
                                n680 = local write "Z-100-L"(w1346) -> ()
                                n681 = local write "Z-100-N"(w1346) -> ()
                                n682 = local write "Z-10K-L"(w1346) -> ()
                                n683 = local write "Z-10K-N"(w1346) -> ()
                                n684 = local write "C-10K-N"(w1346) -> ()
                                n685 = local write "C-10K-L"(w1346) -> ()
                                n686 = local write "C-100-N"(w1346) -> ()
                                n687 = local write "C-100-L"(w1346) -> ()
                              }
                            }
                          }
                          n688 = call <vilib>:"Mean.vi"("X"=w781) -> ("mean"=w763:dbl)  [unwired: 1 out]
                          "mean 2" <- w763
                          n689 = call <vilib>:"Mean.vi"("X"=w780) -> ("mean"=w762:dbl)  [unwired: 1 out]
                          "mean 3" <- w762
                          n690 = call <vilib>:"Mean.vi"("X"=w779) -> ("mean"=w761:dbl)  [unwired: 1 out]
                          "mean 4" <- w761
                          n691 = call <vilib>:"Mean.vi"("X"=w778) -> ("mean"=w760:dbl)  [unwired: 1 out]
                          "mean 5" <- w760
                          n692 = call <vilib>:"Mean.vi"("X"=w777) -> ("mean"=w759:dbl)  [unwired: 1 out]
                          "mean 6" <- w759
                          n693 = call <vilib>:"Mean.vi"("X"=w776) -> ("mean"=w758:dbl)  [unwired: 1 out]
                          "mean 7" <- w758
                          n694 = call <vilib>:"Mean.vi"("X"=w775) -> ("mean"=w757:dbl)  [unwired: 1 out]
                          "mean 8" <- w757
                          n695 = call <vilib>:"Mean.vi"("X"=w774) -> ("mean"=w756:dbl)  [unwired: 1 out]
                          "mean 9" <- w756
                          n696 = call <vilib>:"Mean.vi"("X"=w773) -> ("mean"=w755:dbl)  [unwired: 1 out]
                          "mean 10" <- w755
                          n697 = call <vilib>:"Mean.vi"("X"=w772) -> ("mean"=w754:dbl)  [unwired: 1 out]
                          "mean 11" <- w754
                          n698 = call <vilib>:"Mean.vi"("X"=w771) -> ("mean"=w753:dbl)  [unwired: 1 out]
                          "mean 12" <- w753
                          n699 = call <vilib>:"Mean.vi"("X"=w770) -> ("mean"=w752:dbl)  [unwired: 1 out]
                          "mean 13" <- w752
                          n700 = call <vilib>:"Mean.vi"("X"=w769) -> ("mean"=w751:dbl)  [unwired: 1 out]
                          "mean 14" <- w751
                          n701 = call <vilib>:"Mean.vi"("X"=w768) -> ("mean"=w750:dbl)  [unwired: 1 out]
                          "mean 15" <- w750
                          n702 = call <vilib>:"Mean.vi"("X"=w782) -> ("mean"=w764:dbl)  [unwired: 1 out]
                          "mean" <- w764
                          n703 = call <vilib>:"Mean.vi"("X"=w767) -> ("mean"=w749:dbl)  [unwired: 1 out]
                          "mean 16" <- w749
                        }
                      }
                    }
                    frame #2 {
                      n704 = case shown="True" w1347 {
                        tunnel: w1364 -> [_ w1380]
                        tunnel: w1363 -> [_ w1379]
                        tunnel: w1362 -> [_ w1378]
                        tunnel: w1361 -> [_ w1377]
                        tunnel: w1360 -> [_ w1376]
                        tunnel: w1359 -> [_ w1375]
                        tunnel: w1358 -> [_ w1374]
                        tunnel: w1357 -> [_ w1373]
                        tunnel: w1356 -> [_ w1372]
                        tunnel: w1355 -> [_ w1371]
                        tunnel: w1354 -> [_ w1370]
                        tunnel: w1353 -> [_ w1369]
                        tunnel: w1352 -> [_ w1368]
                        tunnel: w1351 -> [_ w1367]
                        tunnel: w1350 -> [_ w1366]
                        tunnel: w1349 -> [_ w1365]
                        frame False {
                        }
                        frame True {
                          w1394 = "\t"
                          w1411 = i16 4 ("precision (6)")
                          n705 = property on="SET" class="DigNum (strict)"() -> ("Value"=w1412:i32)  [unwired: 2 in, 2 out]
                          n706 = Number To Engineering String(2:w1411, 4:w1365) -> (0:w1408:string)  [unwired: 2 in]
                          n707 = Number To Engineering String(2:w1411, 4:w1379) -> (0:w1407:string)  [unwired: 2 in]
                          n708 = Number To Engineering String(2:w1411, 4:w1378) -> (0:w1406:string)  [unwired: 2 in]
                          n709 = Number To Engineering String(2:w1411, 4:w1377) -> (0:w1405:string)  [unwired: 2 in]
                          n710 = Number To Engineering String(2:w1411, 4:w1376) -> (0:w1404:string)  [unwired: 2 in]
                          n711 = Number To Engineering String(2:w1411, 4:w1375) -> (0:w1403:string)  [unwired: 2 in]
                          n712 = Number To Engineering String(2:w1411, 4:w1374) -> (0:w1402:string)  [unwired: 2 in]
                          n713 = Number To Engineering String(2:w1411, 4:w1373) -> (0:w1401:string)  [unwired: 2 in]
                          n714 = Number To Engineering String(2:w1411, 4:w1372) -> (0:w1400:string)  [unwired: 2 in]
                          n715 = Number To Engineering String(2:w1411, 4:w1371) -> (0:w1399:string)  [unwired: 2 in]
                          n716 = Number To Engineering String(2:w1411, 4:w1370) -> (0:w1398:string)  [unwired: 2 in]
                          n717 = Number To Engineering String(2:w1411, 4:w1369) -> (0:w1397:string)  [unwired: 2 in]
                          n718 = Number To Engineering String(2:w1411, 4:w1368) -> (0:w1396:string)  [unwired: 2 in]
                          n719 = Number To Engineering String(2:w1411, 4:w1367) -> (0:w1395:string)  [unwired: 2 in]
                          n720 = Number To Engineering String(2:w1411, 4:w1380) -> (0:w1409:string)  [unwired: 2 in]
                          n721 = Number To Engineering String(2:w1411, 4:w1366) -> (0:w1393:string)  [unwired: 2 in]
                          n722 = Number To Decimal String(number=w1412) -> (decimal integer string=w1410:string)  [unwired: 1 in]
                          n723 = property on="path RLC_mean" class="Path"() -> ("Value"=w1381:path)  [unwired: 2 in, 2 out]
                          n724 = Open/Create/Replace File(file path (use dialog)=w1381, operation (0:open)=T3."open") -> (refnum out=w1386:refnum<file>, error out=w1385:errorcluster)  [unwired: 2 in, 3 out]
                          n725 = Concatenate Strings(w1410, w1394, w1409, w1394, w1408, w1394, w1407, w1394, w1406, w1394, w1405, w1394, w1404, w1394, w1403, w1394, w1402, w1394, w1401, w1394, w1400, w1394, w1399, w1394, w1398, w1394, w1397, w1394, w1396, w1394, w1395, w1394, w1393, "\r\n") -> (w1382:string)
                          n726 = Set File Position(refnum=w1386, from (0:start)=enum16{"start", "end", "current"}."end", error in=w1385) -> (refnum out=w1388:refnum<file>, error out=w1389:errorcluster)  [unwired: 1 in]
                          n727 = Write to Text File(file (use dialog)=w1388, text=w1382, error in=w1389) -> (refnum out=w1384:refnum<file>, error out=w1383:errorcluster)  [unwired: 1 in, 1 out]
                          n728 = Close File(refnum=w1384, error in=w1383) -> (error out=w1391:errorcluster)  [unwired: 1 out]
                          n729 = call <vilib>:"Simple Error Handler.vi"("error in (no error)"=w1391) -> ()  [unwired: 1 in, 8 out]
                        }
                      }
                    }
                  }
                  n730 = local write "graph RLC"(w700) -> ()
                }
                frame 9 {
                  n731 = flat-sequence {
                    tunnel: w1451 -> [w1462]
                    tunnel: [w1462] -> w1450
                    tunnel: [w1456] -> w1449
                    tunnel: [w1455] -> w1448
                    tunnel: w1450 -> [w1487]
                    tunnel: w1449 -> [_]
                    tunnel: w1448 -> [w1484]
                    frame #0 {
                      n732 = property on="SET" class="DigNum (strict)"() -> ("Value"=w1460:i32)  [unwired: 2 in, 2 out]
                      n733 = Increment(x=w1460) -> (x+1=w1455:i32)
                      n734 = property on="P_max camara" class="DigNum (strict)"() -> ("Value"=w1453:dbl)  [unwired: 2 in, 2 out]
                      n735 = local write "SET"(w1455) -> ()
                      n736 = property on="Camara 2" class="Slide (strict)"() -> ("Value"=w1454:dbl)  [unwired: 2 in, 2 out]
                      n737 = case shown="False" "Boolean" {
                        selector: "Boolean" -> [w1468 w1473]
                        tunnel: [w1470 w1477] -> w1457
                        tunnel: w1455 -> [w1471 _]
                        frame False {
                          n738 = local write "Boolean 2"(w1468) -> ()
                          n739 = Index Array(array="Array", index=w1471) -> (element=w1470:dbl)
                          n740 = Not(x=w1468) -> (.not. x?=→"Boolean 3":bool)
                        }
                        frame True {
                          n741 = property on="Set P auto" class="DigNum (strict)"() -> ("Value"=w1475:dbl)  [unwired: 2 in, 2 out]
                          n742 = Add(x="Step P", y=w1475) -> (x+y=w1477:dbl)
                          n743 = Not(x=w1473) -> (.not. x?=w1474:bool)
                          n744 = local write "Boolean 3"(w1474) -> ()
                          "Boolean 2" <- w1473
                        }
                      }
                      n745 = Greater?(x=w1454, y=w1453) -> (0:w1452:bool)
                      n746 = case shown="True" w1452 {
                        frame False {
                        }
                        frame True {
                          n747 = property on="Desc SET" class="DigNum (strict)"() -> ("Value"=w1464:i32)  [unwired: 2 in, 2 out]
                          n748 = local write "Descarga"(TRUE ("Descarga")) -> ()
                          n749 = Increment(x=w1464) -> (x+1=w1463:i32)
                          n750 = local write "Desc SET"(w1463) -> ()
                        }
                      }
                      n751 = Greater?(x=w1457, y="P_max") -> (0:w1459:bool)
                      n752 = case shown="True" w1459 {
                        tunnel: [w1466 w1467] -> w1456
                        tunnel: "P_max" -> [_ w1467]
                        tunnel: w1457 -> [w1466 _]
                        frame False {
                        }
                        frame True {
                        }
                      }
                      n753 = local write "Set P auto"(w1456) -> ()
                    }
                    frame #1 {
                      n754 = property on="Desc SET" class="DigNum (strict)"() -> ("Value"=w1479:i32)  [unwired: 2 in, 2 out]
                      n755 = Quotient & Remainder(x=w1484, y="Step ZPit") -> (x-y*floor(x/y)=w1485:dbl)  [unwired: 1 out]
                      n756 = Greater Than 0?(x=w1479) -> (x > 0?=w1481:bool)
                      n757 = Equal To 0?(x=w1485) -> (x = 0?=w1483:bool)
                      "Read ZPit" <- w1483
                      n758 = property on="Descarga" class="Bool (strict)"() -> ("Value"=w1478:bool)  [unwired: 2 in, 2 out]
                      n759 = And(x=w1481, y=w1478) -> (x .and. y?=w1480:bool)
                      n760 = case shown="True" w1480 {
                        tunnel: w1483 -> [w1488 _]
                        tunnel: [w1488 w1489] -> w1482
                        frame False {
                        }
                        frame True {
                          w1489 = TRUE
                          n761 = local write "Read ZPit"(w1489) -> ()
                        }
                      }
                      n762 = case shown="True" w1482 {
                        tunnel: w1487 -> [_ w1491]
                        frame False {
                          n763 = local write "Estagio auto"(11 ("Estagio auto")) -> ()
                        }
                        frame True {
                          n764 = Greater?(x=w1491, y=1.0) -> (0:w1496:bool)
                          n765 = case shown="True" w1496 {
                            tunnel: [FALSE ("Boolean") TRUE ("Boolean")] -> w1494
                            frame False {
                              w1516 = TRUE ("Boolean")
                              n766 = local write "Vácuo 2"(w1516) -> ()
                              n767 = Multiply(x="ZPf2 time", y=0.0741) -> (x*y=w1511:dbl)
                              n768 = local write "String"("Limpar volume referencia" ("String")) -> ()
                              n769 = Add(x=w1511, y=1.9801) -> (x+y=w1509:dbl)
                              n770 = call "Controle_vacuo.vi"("time (s) to wait vacuo"=w1509, "Boolean"=w1516) -> ("Vacuo"=w1517:bool)  [unwired: 9 in]
                              n771 = local write "Vácuo 2"(w1517) -> ()
                            }
                            frame True {
                              n772 = property on="ATM wait" class="DigNum (strict)"() -> ("Value"=w1518:u32)  [unwired: 2 in, 2 out]
                              n773 = call "Controle_ATM.vi"("seconds to wait"=w1518) -> ("String 2"=w1521:string, "Atm"=w1520:bool)  [unwired: 9 in]
                              n774 = local write "Atm 2"(w1520) -> ()
                              n775 = local write "String"(w1521) -> ()
                            }
                          }
                          n776 = for {
                            N: 1 -> [_]
                            tunnel: [w1498] -> w1493
                            tunnel: w1494 -> [w1498]
                            n777 = Wait (ms)(milliseconds to wait=u32 500 ("x")) -> ()  [unwired: 1 out]
                          }
                          n778 = case shown="True" w1493 {
                            frame False {
                              n779 = local write "Estagio auto"(10 ("Estagio auto")) -> ()
                            }
                            frame True {
                              w1507 = TRUE ("Boolean")
                              n780 = property on="ZPf2 time" class="DigNum (strict)"() -> ("Value"=w1501:dbl)  [unwired: 2 in, 2 out]
                              n781 = local write "Estagio auto"(10 ("Estagio auto")) -> ()
                              n782 = Multiply(x=w1501, y=0.0741) -> (x*y=w1503:dbl)
                              n783 = local write "Vácuo 2"(w1507) -> ()
                              n784 = local write "String"("Limpar volume referencia" ("String")) -> ()
                              n785 = Add(x=w1503, y=1.9801) -> (x+y=w1500:dbl)
                              n786 = call "Controle_vacuo.vi"("time (s) to wait vacuo"=w1500, "Boolean"=w1507) -> ("Vacuo"=w1508:bool)  [unwired: 9 in]
                              n787 = local write "Vácuo 2"(w1508) -> ()
                            }
                          }
                        }
                      }
                    }
                  }
                }
                frame 10 {
                  n788 = property on="Contador" class="DigNum (strict)"() -> ("Value"=w1523:i32)  [unwired: 2 in, 2 out]
                  n789 = Increment(x=w1523) -> (x+1=w1525:i32)
                  n790 = property on="N fit 2" class="DigNum (strict)"() -> ("Value"=w1522:i32)  [unwired: 2 in, 2 out]
                  n791 = local write "String"("Ler ZPf2 e T" ("String")) -> ()
                  n792 = Equal?(x=w1525, y=w1522) -> (x = y?=w1524:bool)
                  n793 = case shown="True" w1524 {
                    frame False {
                    }
                    frame True {
                      n794 = local write "Estagio auto"(11 ("Estagio auto")) -> ()
                    }
                  }
                }
                frame 11 {
                  n795 = property on="Contador" class="DigNum (strict)"() -> ("Value"=w1531:i32)  [unwired: 2 in, 2 out]
                  n796 = Increment(x=w1531) -> (x+1=w1532:i32)
                  n797 = property on="N fit 2" class="DigNum (strict)"() -> ("Value"=w1528:i32)  [unwired: 2 in, 2 out]
                  n798 = Equal?(x=w1532, y=w1528) -> (x = y?=w1530:bool)
                  n799 = case shown="True" w1530 {
                    tunnel: w1533 -> [_ w1544]
                    tunnel: w1529 -> [_ w1534]
                    frame False {
                    }
                    frame True {
                      w1535 = i16 3 ("precision (6)")
                      w1538 = "\t"
                      n800 = property on="Read ZPit" class="Bool (strict)"() -> ("Value"=w1539:bool)  [unwired: 2 in, 2 out]
                      n801 = property on="T fit" class="DigNum (strict)"() -> ("Value"=w1540:dbl)  [unwired: 2 in, 2 out]
                      n802 = case shown="False" w1539 {
                        tunnel: ["  ==>" w1550] -> w1543
                        tunnel: w1535 -> [_ w1549]
                        frame False {
                        }
                        frame True {
                          n803 = property on="P fit" class="DigNum (strict)"() -> ("Value"=w1548:dbl)  [unwired: 2 in, 2 out]
                          n804 = Number To Fractional String(number=w1548, precision (6)=w1549) -> (F-format string=w1550:string)  [unwired: 2 in]
                        }
                      }
                      n805 = Number To Fractional String(number=w1540, precision (6)=w1535) -> (F-format string=w1542:string)  [unwired: 2 in]
                      n806 = Number To Fractional String(number=w1534, precision (6)=w1535) -> (F-format string=w1537:string)  [unwired: 2 in]
                      n807 = Concatenate Strings(w1543, w1538, w1542, w1538, w1537, "\r\n") -> (w1541:string)
                      n808 = flat-sequence {
                        tunnel: [w1554] -> w1546
                        tunnel: [w1553] -> w1545
                        tunnel: w1541 -> [w1552]
                        tunnel: w1544 -> [w1551]
                        tunnel: w1546 -> [w1568]
                        tunnel: w1545 -> [w1567]
                        frame #0 {
                          n809 = Open/Create/Replace File(file path (use dialog)=w1551, operation (0:open)=T3."open") -> (refnum out=w1560:refnum<file>, error out=w1561:errorcluster)  [unwired: 2 in, 3 out]
                          n810 = Set File Position(refnum=w1560, from (0:start)=enum16{"start", "end", "current"}."end", error in=w1561) -> (refnum out=w1558:refnum<file>, error out=w1557:errorcluster)  [unwired: 1 in]
                          n811 = Write to Text File(file (use dialog)=w1558, text=w1552, error in=w1557) -> (refnum out=w1562:refnum<file>, error out=w1563:errorcluster)  [unwired: 2 out]
                          n812 = Close File(refnum=w1562, error in=w1563) -> (path=w1554:path, error out=w1555:errorcluster)
                          n813 = call <vilib>:"Simple Error Handler.vi"("error in (no error)"=w1555) -> ("error out"=w1553:errorcluster)  [unwired: 1 in, 7 out]
                        }
                        frame #1 {
                          w1564 = TRUE ("ZPit")
                          n814 = Wait (ms)(milliseconds to wait=u32 500) -> ()  [unwired: 1 out]
                          n815 = local write "T 2"(w1564) -> ()
                          n816 = local write "ZPf2 2"(w1564) -> ()
                          n817 = Read from Text File(file (use dialog)=w1568, count=-1 ("Count  3"), error in=w1567) -> (refnum out=w1569:refnum<file>, text=w1573:string, error out=w1570:errorcluster)  [unwired: 1 in, 1 out]
                          n818 = local write "String 3"(w1573) -> ()
                          n819 = Close File(refnum=w1569, error in=w1570) -> (error out=w1571:errorcluster)  [unwired: 1 out]
                          n820 = local write "String"("abrir valvula entrada gas" ("String")) -> ()
                          n821 = call <vilib>:"Simple Error Handler.vi"("error in (no error)"=w1571) -> ()  [unwired: 1 in, 8 out]
                        }
                        frame #2 {
                          n822 = property on="Desc SET" class="DigNum (strict)"() -> ("Value"=w1575:i32)  [unwired: 2 in, 2 out]
                          n823 = Greater Than 0?(x=w1575) -> (x > 0?=w1574:bool)
                          n824 = property on="Camara 2" class="Slide (strict)"() -> ("Value"=w1582:dbl)  [unwired: 2 in, 2 out]
                          n825 = Greater?(x=w1582, y="P_max camara") -> (0:w1580:bool)
                          n826 = property on="Carga" class="Bool (strict)"() -> ("Value"=w1579:bool)  [unwired: 2 in, 2 out]
                          n827 = And(x=w1580, y=w1579) -> (x .and. y?=w1577:bool)
                          n828 = case shown="False" w1574 {
                            tunnel: w1577 -> [w1583 _]
                            tunnel: [w1583 TRUE] -> w1576
                            frame False {
                            }
                            frame True {
                            }
                          }
                          n829 = case shown="True" w1576 {
                            tunnel: [5 ("N fit") w1589] -> w1578
                            frame False {
                              n830 = local write "Estagio auto"(0 ("Estagio auto")) -> ()
                              "Carga" <- TRUE
                              "Descarga" <- FALSE
                            }
                            frame True {
                              n831 = local write "teste slope"(0 ("teste slope")) -> ()
                              n832 = local write "Carga"(FALSE ("Carga")) -> ()
                              n833 = local write "Descarga"(TRUE ("Descarga")) -> ()
                              n834 = local write "Estagio auto"(12 ("Estagio auto")) -> ()
                              n835 = property on="N fit 2" class="DigNum (strict)"() -> ("Value"=w1589:i32)  [unwired: 2 in, 2 out]
                            }
                          }
                          n836 = local write "N fit"(w1578) -> ()
                        }
                      }
                    }
                  }
                }
                frame 12 {
                  w1599 = "\t"
                  n837 = property on="SET" class="DigNum (strict)"() -> ("Value"=w1603:i32)  [unwired: 2 in, 2 out]
                  n838 = Number To Decimal String(number=w1603) -> (decimal integer string=w1606:string)  [unwired: 1 in]
                  n839 = Number To Fractional String(number=0.0, precision (6)=i16 3) -> (F-format string=w1600:string)  [unwired: 2 in]
                  n840 = Concatenate Strings(w1606, w1599, w1600, w1599, w1600, w1599) -> (w1605:string)
                  n841 = flat-sequence {
                    tunnel: w1602 -> [w1611]
                    tunnel: w1605 -> [w1612]
                    tunnel: [w1612] -> w1598
                    tunnel: [w1611] -> w1597
                    tunnel: [w1616] -> w1608
                    tunnel: [w1615] -> w1607
                    tunnel: w1598 -> [w1614]
                    tunnel: w1597 -> [w1613]
                    tunnel: [w1613] -> w1596
                    tunnel: w1608 -> [w1632]
                    tunnel: w1607 -> [w1631]
                    tunnel: w1596 -> [w1626]
                    tunnel: [w1626] -> w1595
                    tunnel: w1595 -> [w1640]
                    tunnel: [w1639] -> w1594
                    tunnel: w1594 -> [w1677]
                    frame #0 {
                      w1610 = FALSE ("ZPit 2")
                      n842 = Wait (ms)(milliseconds to wait=u32 1000) -> ()  [unwired: 1 out]
                      n843 = local write "ZPit 2"(w1610) -> ()
                      n844 = local write "Pit 2"(w1610) -> ()
                      n845 = local write "Pf2 2"(w1610) -> ()
                      n846 = local write "ZPf2 2"(w1610) -> ()
                      n847 = local write "T 2"(w1610) -> ()
                    }
                    frame #1 {
                      n848 = Open/Create/Replace File(file path (use dialog)=w1613, operation (0:open)=T3."open") -> (refnum out=w1622:refnum<file>, error out=w1623:errorcluster)  [unwired: 2 in, 3 out]
                      n849 = Set File Position(refnum=w1622, from (0:start)=enum16{"start", "end", "current"}."end", error in=w1623) -> (refnum out=w1620:refnum<file>, error out=w1619:errorcluster)  [unwired: 1 in]
                      n850 = Write to Text File(file (use dialog)=w1620, text=w1614, error in=w1619) -> (refnum out=w1624:refnum<file>, error out=w1625:errorcluster)  [unwired: 2 out]
                      n851 = Close File(refnum=w1624, error in=w1625) -> (path=w1616:path, error out=w1617:errorcluster)
                      n852 = call <vilib>:"Simple Error Handler.vi"("error in (no error)"=w1617) -> ("error out"=w1615:errorcluster)  [unwired: 1 in, 7 out]
                    }
                    frame #2 {
                      w1627 = TRUE ("ZPit")
                      n853 = local write "Estagio auto"(7 ("Estagio auto")) -> ()
                      n854 = Wait (ms)(milliseconds to wait=u32 500) -> ()  [unwired: 1 out]
                      n855 = local write "ZPit 2"(w1627) -> ()
                      n856 = local write "Pit 2"(w1627) -> ()
                      n857 = Read from Text File(file (use dialog)=w1632, count=-1 ("Count  3"), error in=w1631) -> (refnum out=w1633:refnum<file>, text=w1637:string, error out=w1634:errorcluster)  [unwired: 1 in, 1 out]
                      n858 = local write "String 3"(w1637) -> ()
                      n859 = Close File(refnum=w1633, error in=w1634) -> (error out=w1635:errorcluster)  [unwired: 1 out]
                      n860 = call <vilib>:"Simple Error Handler.vi"("error in (no error)"=w1635) -> ()  [unwired: 1 in, 8 out]
                      n861 = local write "String"("abrir valvula camara" ("String")) -> ()
                    }
                    frame #3 {
                      n862 = property on="Camara 2" class="Slide (strict)"() -> ("Value"=w1643:dbl)  [unwired: 2 in, 2 out]
                      n863 = Less?(x=w1643, y="P_min descarga") -> (x < y?=w1638:bool)
                      n864 = property on="Efetuados" class="DigNum (strict)"() -> ("Value"=w1641:dbl)  [unwired: 2 in, 2 out]
                      n865 = case shown="True" w1638 {
                        tunnel: w1641 -> [_ w1672]
                        tunnel: w1640 -> [_ w1661]
                        tunnel: [TRUE ("data") FALSE ("data")] -> w1639
                        tunnel: w1638 -> [_ w1650]
                        frame False {
                          n866 = property on="Desc SET" class="DigNum (strict)"() -> ("Value"=w1645:i32)  [unwired: 2 in, 2 out]
                          n867 = Increment(x=w1645) -> (x+1=→"Desc SET":i32)
                        }
                        frame True {
                          w1659 = "\r\n"
                          n868 = Increment(x=w1672) -> (x+1=w1647:dbl)
                          "Efetuados" <- w1647
                          n869 = local write "Estagio auto"(0 ("Estagio auto")) -> ()
                          n870 = local write "SET"(0 ("SET")) -> ()
                          n871 = local write "Desc SET"(0 ("Desc SET")) -> ()
                          n872 = local write "Descarga"(FALSE ("Descarga")) -> ()
                          n873 = local write "Carga"(TRUE ("Carga")) -> ()
                          n874 = local write "Set P auto"(0.5 ("Set P auto")) -> ()
                          n875 = Open/Create/Replace File(file path (use dialog)=w1661, operation (0:open)=T3."open") -> (refnum out=w1667:refnum<file>, error out=w1668:errorcluster)  [unwired: 2 in, 3 out]
                          n876 = Less Or Equal?(x="Ciclos", y=w1647) -> (x <= y?=w1648:bool)
                          n877 = And(x=w1650, y=w1648) -> (x .and. y?=w1651:bool)
                          n878 = Set File Position(refnum=w1667, from (0:start)=enum16{"start", "end", "current"}."end", error in=w1668) -> (refnum out=w1665:refnum<file>, error out=w1664:errorcluster)  [unwired: 1 in]
                          n879 = case shown="False" w1651 {
                            frame False {
                              n880 = local write "FIM"(FALSE ("FIM")) -> ()
                            }
                            frame True {
                              w1676 = 1 ("N fit")
                              n881 = local write "Auto Ctrl"(FALSE ("Auto Ctrl")) -> ()
                              n882 = local write "N fit"(w1676) -> ()
                              n883 = local write "N to fit"(w1676) -> ()
                              "FIM" <- TRUE ("stop")
                            }
                          }
                          n884 = Concatenate Strings(w1659, ">>>>>>>>>>>>>>" ("string"), w1659, w1659) -> (w1658:string)
                          n885 = Write to Text File(file (use dialog)=w1665, text=w1658, error in=w1664) -> (refnum out=w1669:refnum<file>, error out=w1670:errorcluster)  [unwired: 2 out]
                          n886 = Close File(refnum=w1669, error in=w1670) -> (error out=w1662:errorcluster)  [unwired: 1 out]
                          n887 = call <vilib>:"Simple Error Handler.vi"("error in (no error)"=w1662) -> ()  [unwired: 1 in, 8 out]
                        }
                      }
                    }
                    frame #4 {
                      w1679 = T7 3 items=["no dialog", "OK message", "continue or stop message", "OK message + warnings", "continue/stop + warnings"] ("type of dialog (OK msg:1)")
                      n888 = local write "Câmara 2"(w1677) -> ()
                      n889 = call-poly <vilib>:"DAQmx Create Virtual Channel.vi"("lines"=tag "Dev1/port0/line3") -> ("task out"=w1688:refnum<k21>, "error out"=w1687:errorcluster)  [unwired: 13 in]
                      n890 = call <vilib>:"DAQmx Start Task.vi"("task/channels in"=w1688, "error in"=w1687) -> ("task out"=w1686:refnum<k21>, "error out"=w1685:errorcluster)  [unwired: 12 in]
                      n891 = call-poly <vilib>:"DAQmx Write.vi"("task/channels in"=w1686, "data"=w1677, "error in"=w1685) -> ("task out"=w1681:refnum<k21>, "error out"=w1680:errorcluster)  [unwired: 10 in, 1 out]
                      n892 = call <vilib>:"DAQmx Stop Task.vi"("task/channels in"=w1681, "error in"=w1680) -> ("task out"=w1683:refnum<k21>, "error out"=w1684:errorcluster)  [unwired: 12 in]
                      n893 = call <vilib>:"DAQmx Clear Task.vi"("task in"=w1683, "error in"=w1684) -> ("error out"=w1678:errorcluster)  [unwired: 13 in]
                      n894 = call <vilib>:"Simple Error Handler.vi"("type of dialog (OK msg:1)"=w1679, "error in (no error)"=w1678) -> ()  [unwired: 3 in, 5 out]
                    }
                  }
                }
              }
            }
          }
          n895 = Index Array(array=w265, index=w263) -> (element=w262:dbl)
          n896 = Index Array(array=w264, index=w263) -> (element=w261:dbl)
          n897 = Bundle("Real 2D Array"=w268, "Best Linear Fit"=w280) -> (w279:T8)  [unwired: 1 in]
          n898 = Bundle("Real 2D Array"=w268, "Best Polynomial Fit"=w269) -> (w266:T9)  [unwired: 1 in]
          n899 = Bundle("Real 2D Array"=w268, "Best Polynomial Fit"=w270) -> (w267:T9)  [unwired: 1 in]
          n900 = case shown="True" w260 {
            tunnel: w262 -> [_ w1691]
            tunnel: w261 -> [_ w1690]
            tunnel: w255 -> [_ w1689]
            frame False {
            }
            frame True {
              "P fit" <- w1691
              "T fit" <- w1690
              "P (bar/s)" <- w1689
            }
          }
          n901 = Build Array(w278, w279, w266) -> (→"Linear T":T10)
          n902 = Bundle("Real 2D Array"=w268, "Best Linear Fit"=w275) -> (w276:T8)  [unwired: 1 in]
          n903 = Build Array(w277, w276, w267) -> (→"Linear P":T10)
          "Contador" <- w259
        }
        n904 = local write "P subarray 2"(dbl[] [0.0, 1.0] ("subarray")) -> ()
        n905 = local write "T subarray 3"(dbl[] [0.0, 1.0] ("subarray")) -> ()
        n906 = local write "time subarray"(dbl[] [0.0, 1.0] ("subarray")) -> ()
      }
    }
    n907 = case shown="False" "Auto Ctrl" {
      tunnel: [TRUE ("Auto Ctrl") FALSE ("Auto Ctrl")] -> w50
      frame False {
      }
      frame True {
      }
    }
    n908 = Exclusive Or(1:w47, 2:"stop") -> (0:w49:bool)
    n909 = case shown="True" "Ligar RLC" {
      tunnel: w44 -> [_ w169]
      frame False {
      }
      frame True {
        w177 = "\t"
        w198 = "\t"
        w181 = "\r"
        w174 = "\r\n"
        w214 = "\r"
        w204 = "\t"
        n910 = Strip Path(path=w169) -> (stripped path=w170:path, name=w173:string)
        n911 = Get Date/Time String(date format (0)=enum16{"short", "long", "abbreviated"}."short", want seconds? (F)=TRUE) -> (date string=w221:string, time string=w220:string)  [unwired: 1 in]
        n912 = Concatenate Strings("SET" ("Nota 4"), w177, "DATE" ("Nota 4"), w177, "TIME" ("Nota 4"), w177, w198, "P (BAR)" ("Nota 4"), w198, "T (ºC)" ("Nota 4"), w198, "C-50-L" ("Nota 4"), w198, "C-50-N" ("Nota 4"), w198, "C-100-L" ("Nota 4"), w198, "C-100-N" ("Nota 4"), w198, "C-1K-L" ("Nota 4"), w198, "C-1K-N" ("Nota 4"), w198, "C-10K-L" ("Nota 4"), w198, "C-10K-N" ("Nota 4"), w198, "Z-50-L" ("Nota 4"), w198, "Z-50-N" ("Nota 4"), w198, "Z-100-L" ("Nota 4"), w198, "Z-100-N" ("Nota 4"), w198, "Z-1K-L" ("Nota 4"), w198, "Z-1K-N" ("Nota 4"), w198, "Z-10K-L" ("Nota 4"), w198, "Z-10K-N" ("Nota 4")) -> (w182:string)
        n913 = Concatenate Strings(w221, w204, w220) -> (w216:string)
        n914 = Concatenate Strings(w173, "_RLC_CDH completo" ("string")) -> (w171:string)
        n915 = Concatenate Strings("Sievert RLC - CDH:" ("string"), w204, w174, w174) -> (w202:string)
        n916 = Concatenate Strings("Data Table" ("string"), w181, "==========" ("string"), w181, w182, w181) -> (w215:string)
        n917 = File Dialog(6:".txt" ("pattern label"), 9:w171, 11:w170) -> (0:w212:errorcluster, 3:w213:path)  [unwired: 2 in, 4 out]
        n918 = Open/Create/Replace File(file path (use dialog)=w213, error in=w212, operation (0:open)=T3."replace or create with confirmation", access (0:read/write)=enum16{"read/write", "read-only", "write-only"}."read/write") -> (refnum out=w209:refnum<file>, error out=w208:errorcluster)  [unwired: 3 out]
        n919 = Concatenate Strings(w216, w214, w214, w202, w214, w214, "Nota 01: MEDIDAS COM RLC 300 - MULTILEITURA" ("Nota 4"), w214, w214, w215) -> (w219:string)
        n920 = Write to Text File(file (use dialog)=w209, text=w219, error in=w208) -> (refnum out=w207:refnum<file>, error out=w205:errorcluster)  [unwired: 1 in, 1 out]
        n921 = Close File(refnum=w207, error in=w205) -> (path=w201:path)  [unwired: 1 out]
        n922 = local write "path RLC_completo"(w201) -> ()
      }
    }
    n923 = case shown="True" "Ligar RLC" {
      tunnel: w44 -> [_ w112]
      frame False {
      }
      frame True {
        w121 = "\t"
        w142 = "\t"
        w125 = "\r"
        w118 = "\r\n"
        w157 = "\r"
        w147 = "\t"
        n924 = Strip Path(path=w112) -> (stripped path=w114:path, name=w117:string)
        n925 = Get Date/Time String(date format (0)=enum16{"short", "long", "abbreviated"}."short", want seconds? (F)=TRUE) -> (date string=w164:string, time string=w163:string)  [unwired: 1 in]
        n926 = Concatenate Strings("SET" ("Nota 4"), w121, "DATE" ("Nota 4"), w121, "TIME" ("Nota 4"), w121, w142, "P (BAR)" ("Nota 4"), w142, "T (ºC)" ("Nota 4"), w142, "C-50-L" ("Nota 4"), w142, "C-50-N" ("Nota 4"), w142, "C-100-L" ("Nota 4"), w142, "C-100-N" ("Nota 4"), w142, "C-1K-L" ("Nota 4"), w142, "C-1K-N" ("Nota 4"), w142, "C-10K-L" ("Nota 4"), w142, "C-10K-N" ("Nota 4"), w142, "Z-50-L" ("Nota 4"), w142, "Z-50-N" ("Nota 4"), w142, "Z-100-L" ("Nota 4"), w142, "Z-100-N" ("Nota 4"), w142, "Z-1K-L" ("Nota 4"), w142, "Z-1K-N" ("Nota 4"), w142, "Z-10K-L" ("Nota 4"), w142, "Z-10K-N" ("Nota 4")) -> (w126:string)
        n927 = Concatenate Strings(w164, w147, w163) -> (w159:string)
        n928 = Concatenate Strings(w117, "_RLC_CDH mean" ("string")) -> (w115:string)
        n929 = Concatenate Strings("Sievert RLC - CDH:" ("string"), w147, w118, w118) -> (w145:string)
        n930 = Concatenate Strings("Data Table" ("string"), w125, "==========" ("string"), w125, w126, w125) -> (w158:string)
        n931 = File Dialog(6:".txt" ("pattern label"), 9:w115, 11:w114) -> (0:w155:errorcluster, 3:w156:path)  [unwired: 2 in, 4 out]
        n932 = Open/Create/Replace File(file path (use dialog)=w156, error in=w155, operation (0:open)=T3."replace or create with confirmation", access (0:read/write)=enum16{"read/write", "read-only", "write-only"}."read/write") -> (refnum out=w152:refnum<file>, error out=w151:errorcluster)  [unwired: 3 out]
        n933 = Concatenate Strings(w159, w157, w157, w145, w157, w157, "Nota 01: MEDIDAS COM RLC 300 - MULTILEITURA" ("Nota 4"), w157, w157, w158) -> (w162:string)
        n934 = Write to Text File(file (use dialog)=w152, text=w162, error in=w151) -> (refnum out=w150:refnum<file>, error out=w148:errorcluster)  [unwired: 1 in, 1 out]
        n935 = Close File(refnum=w150, error in=w148) -> (path=w113:path)  [unwired: 1 out]
        n936 = local write "path RLC_mean"(w113) -> ()
      }
    }
    n937 = case shown="True" "RLC on/off" {
      tunnel: w37 -> [_ w55]
      frame False {
      }
      frame True {
        n938 = call "RLC READ DINAMICO.vi"("Boolean"="graph RLC", "Path"=w55, "String"="Combo Box") -> ("MEASURE R [Ohm ]"=w59:dbl, "MEASURE C [F ]"=w58:dbl)  [unwired: 7 in]
        "MEASURE C [F ]" <- w58
        n939 = Merge Signals(w58, w59) -> (→"Waveform Chart":dynamicdata)
        "String 4" <- "Combo Box"
      }
    }
    n940 = case shown="True" "Manual Ctrl" {
      tunnel: w37 -> [_ w1773]
      tunnel: "RLC on/off" -> [_ w1772]
      tunnel: [FALSE w1775] -> w39
      frame False {
      }
      frame True {
        w1787 = 0 ("polynomial order")
        n941 = for {
          N: "N to fit" -> [_]
          tunnel: [w2460] -> w1762 mode=indexing
          tunnel: [w2465] -> w1780 mode=indexing
          tunnel: [w2465] -> w1766 mode=indexing
          tunnel: [w2453] -> w1771 mode=indexing
          i -> [w2465]
          n942 = case shown="False" "Clear" {
            frame False {
            }
            frame True {
              n943 = property on="P-manual" class="WFChart (strict)"("History Data"=dynamicdata[] []) -> ()  [unwired: 2 in, 2 out]
            }
          }
          n944 = case shown="True" "Câmara" {
            frame False {
            }
            frame True {
              n945 = property on="Vol Ref" class="Slide (strict)"() -> ("Value"=w2512:dbl)  [unwired: 2 in, 2 out]
              n946 = local write "Camara"(w2512) -> ()
            }
          }
          n947 = case shown="True" "Guardar\nCinetica" {
            frame False {
            }
            frame True {
              n948 = feedback #2() -> (w2467:bool)  [unwired: 1 in]
              "x >= y?" <- w2467
              n949 = call "Elapsed Time"("Reset"=w2467) -> ("Elapsed Time (s)"=w2469:dbl)  [unwired: 11 in, 7 out]
              "Elapsed Time (sec)" <- w2469
              n950 = case shown="True" w2467 {
                frame False {
                }
                frame True {
                  n951 = flat-sequence {
                    tunnel: [w2484] -> w2472
                    tunnel: [w2483] -> w2471
                    tunnel: w2472 -> [w2502]
                    tunnel: w2471 -> [w2501]
                    frame #0 {
                      w2477 = "\t"
                      w2474 = i16 4 ("precision (6)")
                      n952 = property on="MEASURE C [F ]" class="DigNum (strict)"() -> ("Value"=w2473:dbl)  [unwired: 2 in, 2 out]
                      n953 = property on="termopar K" class="DigNum (strict)"() -> ("Value"=w2478:dbl)  [unwired: 2 in, 2 out]
                      n954 = Number To Fractional String(number=w2478, precision (6)=w2474) -> (F-format string=w2479:string)  [unwired: 2 in]
                      n955 = property on="P cinetica mean" class="DigNum (strict)"() -> ("Value"=w2481:dbl)  [unwired: 2 in, 2 out]
                      n956 = property on="T cinetica mean 2" class="DigNum (strict)"() -> ("Value"=w2480:dbl)  [unwired: 2 in, 2 out]
                      n957 = property on="path 2_cinetica" class="Path"() -> ("Value"=w2482:path)  [unwired: 2 in, 2 out]
                      n958 = Get Date/Time String(date format (0)=enum16{"short", "long", "abbreviated"}."short", want seconds? (F)=TRUE) -> (date string=w2498:string, time string=w2497:string)  [unwired: 1 in]
                      n959 = Number To Exponential String(number=w2473, precision (6)=w2474) -> (E-format string=w2476:string)  [unwired: 2 in]
                      n960 = Number To Fractional String(number=w2481, precision (6)=w2474) -> (F-format string=w2496:string)  [unwired: 2 in]
                      n961 = Number To Fractional String(number=w2480, precision (6)=w2474) -> (F-format string=w2495:string)  [unwired: 2 in]
                      n962 = Open/Create/Replace File(file path (use dialog)=w2482, operation (0:open)=T3."open") -> (refnum out=w2491:refnum<file>, error out=w2492:errorcluster)  [unwired: 2 in, 3 out]
                      n963 = Concatenate Strings(w2498, w2477, w2497, w2477, w2496, w2477, w2495, w2477, w2479, w2477, w2476, "\r\n") -> (w2485:string)
                      n964 = Set File Position(refnum=w2491, from (0:start)=enum16{"start", "end", "current"}."end", error in=w2492) -> (refnum out=w2489:refnum<file>, error out=w2488:errorcluster)  [unwired: 1 in]
                      n965 = Write to Text File(file (use dialog)=w2489, text=w2485, error in=w2488) -> (refnum out=w2493:refnum<file>, error out=w2494:errorcluster)  [unwired: 2 out]
                      n966 = Close File(refnum=w2493, error in=w2494) -> (path=w2484:path, error out=w2486:errorcluster)
                      n967 = call <vilib>:"Simple Error Handler.vi"("error in (no error)"=w2486) -> ("error out"=w2483:errorcluster)  [unwired: 1 in, 7 out]
                    }
                    frame #1 {
                      n968 = Read from Text File(file (use dialog)=w2502, count=-1 ("Count  3"), error in=w2501) -> (refnum out=w2503:refnum<file>, text=w2507:string, error out=w2504:errorcluster)  [unwired: 1 in, 1 out]
                      n969 = local write "String_cinetica"(w2507) -> ()
                      n970 = Close File(refnum=w2503, error in=w2504) -> (error out=w2505:errorcluster)  [unwired: 1 out]
                      n971 = call <vilib>:"Simple Error Handler.vi"("error in (no error)"=w2505) -> ()  [unwired: 1 in, 8 out]
                    }
                    frame #2 {
                      n972 = local write "P T  index"(0 ("P T  index")) -> ()
                      n973 = local write "T subarray 2"(dbl[] [0.0, 1.0] ("subarray")) -> ()
                      n974 = local write "P subarray"(dbl[] [0.0, 1.0] ("subarray")) -> ()
                    }
                  }
                }
              }
              n975 = Greater Or Equal?(x=w2469, y="seconds") -> (x >= y?=w2470:bool)
              n976 = feedback-in #2(w2470) -> ()
            }
          }
          n977 = property on="correção NTC" class="DigNum (strict)"() -> ("Value"=w2456:dbl)  [unwired: 2 in, 2 out]
          n978 = call "Read P T.vi"("correção NTC"=w2456) -> ("Sievert01"=w2449:dbl, "mean H2 sensor"=→"mean H2 sensor (V)":dbl, "termopar K"=w2454:dbl, "output NTC"=w2453:dbl, "P Set 2 Output 2"=w2452:dbl)  [unwired: 3 in, 7 out]
          "termopar K" <- w2454
          "output NTC" <- w2453
          n979 = stacked-sequence {
            tunnel: "Entrada Gás" -> [w2543 _ _ _]
            tunnel: "Vácuo" -> [_ w2555 _ _]
            tunnel: "Câmara" -> [_ _ w2567 _]
            tunnel: "ATM" -> [_ _ _ w2579]
            frame #0 {
              w2548 = T7 3 items=["no dialog", "OK message", "continue or stop message", "OK message + warnings", "continue/stop + warnings"] ("type of dialog (OK msg:1)")
              n980 = property on="Entrada gás" class="Bool (strict)"("Value"=w2543) -> ()  [unwired: 2 in, 2 out]
              n981 = call-poly <vilib>:"DAQmx Create Virtual Channel.vi"("lines"=tag "Dev1/port0/line1") -> ("task out"=w2546:refnum<k21>, "error out"=w2547:errorcluster)  [unwired: 13 in]
              n982 = call <vilib>:"DAQmx Start Task.vi"("task/channels in"=w2546, "error in"=w2547) -> ("task out"=w2549:refnum<k21>, "error out"=w2550:errorcluster)  [unwired: 12 in]
              n983 = call-poly <vilib>:"DAQmx Write.vi"("task/channels in"=w2549, "data"=w2543, "error in"=w2550) -> ("task out"=w2554:refnum<k21>, "error out"=w2551:errorcluster)  [unwired: 10 in, 1 out]
              n984 = call <vilib>:"DAQmx Stop Task.vi"("task/channels in"=w2554, "error in"=w2551) -> ("task out"=w2553:refnum<k21>, "error out"=w2552:errorcluster)  [unwired: 12 in]
              n985 = call <vilib>:"DAQmx Clear Task.vi"("task in"=w2553, "error in"=w2552) -> ("error out"=w2545:errorcluster)  [unwired: 13 in]
              n986 = call <vilib>:"Simple Error Handler.vi"("type of dialog (OK msg:1)"=w2548, "error in (no error)"=w2545) -> ()  [unwired: 3 in, 5 out]
            }
            frame #1 {
              w2560 = T7 3 items=["no dialog", "OK message", "continue or stop message", "OK message + warnings", "continue/stop + warnings"] ("type of dialog (OK msg:1)")
              n987 = property on="Vácuo" class="Bool (strict)"("Value"=w2555) -> ()  [unwired: 2 in, 2 out]
              n988 = call-poly <vilib>:"DAQmx Create Virtual Channel.vi"("lines"=tag "Dev1/port0/line2") -> ("task out"=w2558:refnum<k21>, "error out"=w2559:errorcluster)  [unwired: 13 in]
              n989 = call <vilib>:"DAQmx Start Task.vi"("task/channels in"=w2558, "error in"=w2559) -> ("task out"=w2561:refnum<k21>, "error out"=w2562:errorcluster)  [unwired: 12 in]
              n990 = call-poly <vilib>:"DAQmx Write.vi"("task/channels in"=w2561, "data"=w2555, "error in"=w2562) -> ("task out"=w2566:refnum<k21>, "error out"=w2563:errorcluster)  [unwired: 10 in, 1 out]
              n991 = call <vilib>:"DAQmx Stop Task.vi"("task/channels in"=w2566, "error in"=w2563) -> ("task out"=w2565:refnum<k21>, "error out"=w2564:errorcluster)  [unwired: 12 in]
              n992 = call <vilib>:"DAQmx Clear Task.vi"("task in"=w2565, "error in"=w2564) -> ("error out"=w2557:errorcluster)  [unwired: 13 in]
              n993 = call <vilib>:"Simple Error Handler.vi"("type of dialog (OK msg:1)"=w2560, "error in (no error)"=w2557) -> ()  [unwired: 3 in, 5 out]
            }
            frame #2 {
              w2572 = T7 3 items=["no dialog", "OK message", "continue or stop message", "OK message + warnings", "continue/stop + warnings"] ("type of dialog (OK msg:1)")
              n994 = property on="Câmara" class="Bool (strict)"("Value"=w2567) -> ()  [unwired: 2 in, 2 out]
              n995 = call-poly <vilib>:"DAQmx Create Virtual Channel.vi"("lines"=tag "Dev1/port0/line3") -> ("task out"=w2570:refnum<k21>, "error out"=w2571:errorcluster)  [unwired: 13 in]
              n996 = call <vilib>:"DAQmx Start Task.vi"("task/channels in"=w2570, "error in"=w2571) -> ("task out"=w2573:refnum<k21>, "error out"=w2574:errorcluster)  [unwired: 12 in]
              n997 = call-poly <vilib>:"DAQmx Write.vi"("task/channels in"=w2573, "data"=w2567, "error in"=w2574) -> ("task out"=w2578:refnum<k21>, "error out"=w2575:errorcluster)  [unwired: 10 in, 1 out]
              n998 = call <vilib>:"DAQmx Stop Task.vi"("task/channels in"=w2578, "error in"=w2575) -> ("task out"=w2577:refnum<k21>, "error out"=w2576:errorcluster)  [unwired: 12 in]
              n999 = call <vilib>:"DAQmx Clear Task.vi"("task in"=w2577, "error in"=w2576) -> ("error out"=w2569:errorcluster)  [unwired: 13 in]
              n1000 = call <vilib>:"Simple Error Handler.vi"("type of dialog (OK msg:1)"=w2572, "error in (no error)"=w2569) -> ()  [unwired: 3 in, 5 out]
            }
            frame #3 {
              w2584 = T7 3 items=["no dialog", "OK message", "continue or stop message", "OK message + warnings", "continue/stop + warnings"] ("type of dialog (OK msg:1)")
              n1001 = property on="Atm" class="Bool (strict)"("Value"=w2579) -> ()  [unwired: 2 in, 2 out]
              n1002 = call-poly <vilib>:"DAQmx Create Virtual Channel.vi"("lines"=tag "Dev1/port0/line4") -> ("task out"=w2582:refnum<k21>, "error out"=w2583:errorcluster)  [unwired: 13 in]
              n1003 = call <vilib>:"DAQmx Start Task.vi"("task/channels in"=w2582, "error in"=w2583) -> ("task out"=w2585:refnum<k21>, "error out"=w2586:errorcluster)  [unwired: 12 in]
              n1004 = call-poly <vilib>:"DAQmx Write.vi"("task/channels in"=w2585, "data"=w2579, "error in"=w2586) -> ("task out"=w2590:refnum<k21>, "error out"=w2587:errorcluster)  [unwired: 10 in, 1 out]
              n1005 = call <vilib>:"DAQmx Stop Task.vi"("task/channels in"=w2590, "error in"=w2587) -> ("task out"=w2589:refnum<k21>, "error out"=w2588:errorcluster)  [unwired: 12 in]
              n1006 = call <vilib>:"DAQmx Clear Task.vi"("task in"=w2589, "error in"=w2588) -> ("error out"=w2581:errorcluster)  [unwired: 13 in]
              n1007 = call <vilib>:"Simple Error Handler.vi"("type of dialog (OK msg:1)"=w2584, "error in (no error)"=w2581) -> ()  [unwired: 3 in, 5 out]
            }
          }
          n1008 = Multiply(x=w2452, y=10.0) -> (x*y=w2460:dbl)
          n1009 = local write "Vol Ref"(w2460) -> ()
          n1010 = Multiply(x=w2449, y=10.0) -> (x*y=w2450:dbl)
          n1011 = stacked-sequence {
            tunnel: w2460 -> [w2535 _]
            tunnel: w2453 -> [w2514 _]
            frame #0 {
              w2513 = 2 ("y")
              n1012 = property on="P subarray" class="Arr (strict)"() -> ("Value"=w2537:dbl[])  [unwired: 2 in, 2 out]
              n1013 = property on="P T  index" class="DigNum (strict)"() -> ("Value"=w2515:i32)  [unwired: 2 in, 2 out]
              n1014 = Replace Array Subset(array=w2537, new element=w2535, index=w2515) -> (w2533:dbl[])
              n1015 = property on="T subarray 2" class="Arr (strict)"() -> ("Value"=w2524:dbl[])  [unwired: 2 in, 2 out]
              n1016 = Replace Array Subset(array=w2524, new element=w2514, index=w2515) -> (w2521:dbl[])
              n1017 = call-poly <vilib>:"Array To Matrix.vi"("Real 1D Array"=w2533) -> ("Real Matrix (Column Vector)"=w2540:T5)
              n1018 = Matrix Size(0:w2540) -> (1:w2539:i32, 2:w2538:i32)
              n1019 = call-poly <vilib>:"Array To Matrix.vi"("Real 1D Array"=w2521) -> ("Real Matrix (Column Vector)"=w2527:T5)
              n1020 = Matrix Size(0:w2527) -> (1:w2526:i32, 2:w2525:i32)
              n1021 = Increment(x=w2539) -> (x+1=w2528:i32)
              n1022 = Subtract(x=w2528, y=w2513) -> (x-y=w2529:i32)
              n1023 = Resize Matrix(1:w2538, 2:w2528, 4:w2540) -> (0:w2536:T5)
              n1024 = Increment(x=w2526) -> (x+1=w2516:i32)
              n1025 = Subtract(x=w2516, y=w2513) -> (x-y=w2517:i32)
              n1026 = Resize Matrix(1:w2525, 2:w2516, 4:w2527) -> (0:w2523:T5)
              n1027 = call-poly <vilib>:"Matrix To Array.vi"("Real Matrix"=w2536) -> ("Real 2D Array"=w2531:dbl[][])
              n1028 = call-poly <vilib>:"Matrix To Array.vi"("Real Matrix"=w2523) -> ("Real 2D Array"=w2519:dbl[][])
              n1029 = Reshape Array(w2531, w2528) -> (w2530:dbl[])
              n1030 = Reshape Array(w2519, w2516) -> (w2518:dbl[])
              n1031 = local write "P subarray"(w2530) -> ()
              n1032 = Reshape Array(w2530, w2529) -> (w2532:dbl[])
              n1033 = local write "T subarray 2"(w2518) -> ()
              n1034 = call <vilib>:"Mean.vi"("X"=w2532) -> ("mean"=→"P cinetica mean":dbl)  [unwired: 1 out]
              n1035 = Reshape Array(w2518, w2517) -> (w2520:dbl[])
              n1036 = call <vilib>:"Mean.vi"("X"=w2520) -> ("mean"=→"T cinetica mean 2":dbl)  [unwired: 1 out]
            }
            frame #1 {
              n1037 = property on="P T  index" class="DigNum (strict)"() -> ("Value"=w2542:i32)  [unwired: 2 in, 2 out]
              n1038 = Increment(x=w2542) -> (x+1=w2541:i32)
              n1039 = local write "P T  index"(w2541) -> ()
            }
          }
          n1040 = Merge Signals(w2460, w2453, w2454, w2450) -> (→"P-manual":dynamicdata)
          "N" <- w2465
        }
        n1041 = case shown="True" "Save manual" {
          selector: "Save manual" -> [_ w2389]
          frame False {
          }
          frame True {
            n1042 = feedback #3() -> (w2385:dbl)  [unwired: 1 in]
            n1043 = Equal To 0?(x=w2385) -> (x = 0?=w2391:bool)
            n1044 = stacked-sequence {
              tunnel: w2391 -> [_ w2407 _]
              tunnel: [_ w2406 _] -> w2387
              frame #0 {
                w2400 = i16 3 ("precision (6)")
                n1045 = property on="T fit" class="DigNum (strict)"() -> ("Value"=w2402:dbl)  [unwired: 2 in, 2 out]
                n1046 = property on="p fit" class="DigNum (strict)"() -> ("Value"=w2403:dbl)  [unwired: 2 in, 2 out]
                n1047 = property on="termopar K" class="DigNum (strict)"() -> ("Value"=w2401:dbl)  [unwired: 2 in, 2 out]
                n1048 = Number To Fractional String(number=w2402, precision (6)=w2400) -> (F-format string=→"T string":string)  [unwired: 2 in]
                n1049 = Number To Fractional String(number=w2403, precision (6)=w2400) -> (F-format string=→"P string":string)  [unwired: 2 in]
                n1050 = Number To Fractional String(number=w2401, precision (6)=w2400) -> (F-format string=→"termopar K":string)  [unwired: 2 in]
              }
              frame #1 {
                n1051 = case shown="True" w2407 {
                  tunnel: [TRUE ("y") FALSE ("y")] -> w2406
                  frame False {
                    n1052 = property on="path" class="Path"() -> ("Value"=w2411:path)  [unwired: 2 in, 2 out]
                    n1053 = property on="P string" class="Str"() -> ("Value"=w2410:string)  [unwired: 2 in, 2 out]
                    n1054 = Concatenate Strings(w2410, "\t") -> (w2408:string)
                    n1055 = Open/Create/Replace File(file path (use dialog)=w2411, operation (0:open)=T3."open") -> (refnum out=w2415:refnum<file>, error out=w2414:errorcluster)  [unwired: 2 in, 3 out]
                    n1056 = Set File Position(refnum=w2415, from (0:start)=enum16{"start", "end", "current"}."end", error in=w2414) -> (refnum out=w2417:refnum<file>, error out=w2418:errorcluster)  [unwired: 1 in]
                    n1057 = Write to Text File(file (use dialog)=w2417, text=w2408, error in=w2418) -> (refnum out=w2413:refnum<file>, error out=w2412:errorcluster)  [unwired: 2 out]
                    n1058 = Close File(refnum=w2413, error in=w2412) -> (error out=w2420:errorcluster)  [unwired: 1 out]
                    n1059 = call <vilib>:"Simple Error Handler.vi"("error in (no error)"=w2420) -> ()  [unwired: 1 in, 8 out]
                  }
                  frame True {
                    w2423 = "\t"
                    n1060 = property on="path" class="Path"() -> ("Value"=w2430:path)  [unwired: 2 in, 2 out]
                    n1061 = property on="Count SET" class="DigNum (strict)"() -> ("Value"=w2426:i32)  [unwired: 2 in, 2 out]
                    n1062 = Open/Create/Replace File(file path (use dialog)=w2430, operation (0:open)=T3."open") -> (refnum out=w2429:refnum<file>, error out=w2428:errorcluster)  [unwired: 2 in, 3 out]
                    n1063 = Increment(x=w2426) -> (x+1=w2427:i32)
                    "Set atual" <- w2427
                    n1064 = Set File Position(refnum=w2429, from (0:start)=enum16{"start", "end", "current"}."end", error in=w2428) -> (refnum out=w2438:refnum<file>, error out=w2439:errorcluster)  [unwired: 1 in]
                    n1065 = Number To Decimal String(number=w2427) -> (decimal integer string=w2431:string)  [unwired: 1 in]
                    n1066 = property on="termopar K" class="Str"() -> ("Value"=w2422:string)  [unwired: 2 in, 2 out]
                    n1067 = property on="T string" class="Str"() -> ("Value"=w2424:string)  [unwired: 2 in, 2 out]
                    n1068 = Concatenate Strings(w2424, w2423, w2422, "\r\n", w2431, w2423) -> (w2433:string)
                    n1069 = Write to Text File(file (use dialog)=w2438, text=w2433, error in=w2439) -> (refnum out=w2436:refnum<file>, error out=w2435:errorcluster)  [unwired: 2 out]
                    n1070 = Close File(refnum=w2436, error in=w2435) -> (error out=w2441:errorcluster)  [unwired: 1 out]
                    n1071 = call <vilib>:"Simple Error Handler.vi"("error in (no error)"=w2441) -> ()  [unwired: 1 in, 8 out]
                    "T" <- TRUE ("T")
                  }
                }
              }
              frame #2 {
                n1072 = property on="path" class="Path"() -> ("Value"=w2443:path)  [unwired: 2 in, 2 out]
                n1073 = property on="Set atual" class="DigNum (strict)"() -> ("Value"=w2442:i32)  [unwired: 2 in, 2 out]
                n1074 = local write "Count SET"(w2442) -> ()
                n1075 = Read from Text File(file (use dialog)=w2443, count=-1 ("Count  3")) -> (refnum out=w2445:refnum<file>, text=w2444:string, error out=w2446:errorcluster)  [unwired: 2 in, 1 out]
                n1076 = property on="String 2" class="Str"("Value"=w2444) -> ()  [unwired: 2 in, 2 out]
                n1077 = Close File(refnum=w2445, error in=w2446) -> (error out=w2448:errorcluster)  [unwired: 1 out]
                n1078 = call <vilib>:"Simple Error Handler.vi"("error in (no error)"=w2448) -> ()  [unwired: 1 in, 8 out]
              }
            }
            n1079 = Implies(1:w2387, 2:w2389) -> (0:w2388:bool)
            n1080 = Select(t=w2385, s=w2388, f=5.0 ("t")) -> (s? t:f=w2386:dbl)
            n1081 = case shown="1" w2386 {
              frame 0, Default {
              }
              frame 1 {
                "ZPf2" <- TRUE ("ZPf2")
              }
              frame 2 {
                "Pf2" <- TRUE ("Pf2")
              }
              frame 3 {
                "Pit" <- TRUE ("Pit")
              }
              frame 4 {
                n1082 = local write "T"(FALSE ("T")) -> ()
                "ZPit" <- TRUE ("ZPit")
              }
              frame 5 {
                w2398 = FALSE
                n1083 = local write "Pit"(w2398) -> ()
                n1084 = local write "ZPf2"(w2398) -> ()
                n1085 = local write "ZPit"(w2398) -> ()
                n1086 = local write "Pf2"(w2398) -> ()
              }
            }
            n1087 = Decrement(x=w2386) -> (x-1=w2392:dbl)
            n1088 = feedback-in #3(w2392) -> ()
          }
        }
        n1089 = case shown="True" w1772 {
          tunnel: [FALSE ("Save manual") w2384] -> w1774
          tunnel: "Save manual" -> [_ w2384]
          frame False {
          }
          frame True {
          }
        }
        n1090 = case shown="True" w1772 {
          tunnel: [FALSE w1792] -> w1775
          tunnel: w1774 -> [_ w1791]
          tunnel: w1773 -> [_ w1790]
          frame False {
          }
          frame True {
            n1091 = flat-sequence {
              tunnel: w1790 -> [w1813]
              tunnel: w1791 -> [w1814]
              tunnel: [w1814] -> w1811
              tunnel: [w1813] -> w1810
              tunnel: [w1821] -> w1809
              tunnel: [w1822] -> w1808
              tunnel: [w1823] -> w1807
              tunnel: [w1824] -> w1806
              tunnel: [w1825] -> w1805
              tunnel: [w1826] -> w1804
              tunnel: [w1827] -> w1803
              tunnel: [w1829] -> w1802
              tunnel: [w1830] -> w1801
              tunnel: [w1831] -> w1800
              tunnel: [w1832] -> w1799
              tunnel: [w1833] -> w1798
              tunnel: [w1828] -> w1797
              tunnel: [w1820] -> w1796
              tunnel: [w1819] -> w1795
              tunnel: [w1818] -> w1794
              tunnel: [w1817] -> w1793
              tunnel: w1811 -> [w1816]
              tunnel: w1810 -> [w1815]
              tunnel: w1809 -> [w2331]
              tunnel: w1808 -> [w2330]
              tunnel: w1807 -> [w2329]
              tunnel: w1806 -> [w2328]
              tunnel: w1805 -> [w2327]
              tunnel: w1804 -> [w2326]
              tunnel: w1803 -> [w2325]
              tunnel: w1802 -> [w2324]
              tunnel: w1801 -> [w2323]
              tunnel: w1800 -> [w2322]
              tunnel: w1799 -> [w2321]
              tunnel: w1798 -> [w2320]
              tunnel: w1797 -> [w2319]
              tunnel: w1796 -> [w2332]
              tunnel: w1795 -> [w2333]
              tunnel: w1794 -> [w2334]
              tunnel: [w2317] -> w1792
              tunnel: w1793 -> [w2317]
              tunnel: [TRUE] -> w1789
              frame #0 {
                n1092 = local write "graph RLC"(FALSE) -> ()
              }
              frame #1 {
                n1093 = case shown="True" w1816 {
                  tunnel: [_ w1868] -> w1817
                  tunnel: w1815 -> [_ w1850]
                  tunnel: [_ w1849] -> w1818
                  tunnel: [_ w1848] -> w1819
                  tunnel: [_ w1847] -> w1820
                  tunnel: [_ w1846] -> w1821
                  tunnel: [_ w1845] -> w1822
                  tunnel: [_ w1844] -> w1823
                  tunnel: [_ w1843] -> w1824
                  tunnel: [_ w1842] -> w1825
                  tunnel: [_ w1841] -> w1826
                  tunnel: [_ w1840] -> w1827
                  tunnel: [_ w1839] -> w1828
                  tunnel: [_ w1838] -> w1829
                  tunnel: [_ w1837] -> w1830
                  tunnel: [_ w1836] -> w1831
                  tunnel: [_ w1835] -> w1832
                  tunnel: [_ w1834] -> w1833
                  frame False {
                  }
                  frame True {
                    n1094 = for {
                      N: 5 -> [_]
                      tunnel: TRUE -> [w1891]
                      tunnel: FALSE -> [w1890]
                      tunnel: [w1889] -> w1868
                      tunnel: [w1888] -> w1866 mode=indexing
                      tunnel: [w1887] -> w1865 mode=indexing
                      tunnel: [w1886] -> w1864 mode=indexing
                      tunnel: [w1885] -> w1863 mode=indexing
                      tunnel: [w1884] -> w1862 mode=indexing
                      tunnel: [w1883] -> w1861 mode=indexing
                      tunnel: [w1882] -> w1860 mode=indexing
                      tunnel: [w1881] -> w1859 mode=indexing
                      tunnel: [w1880] -> w1858 mode=indexing
                      tunnel: [w1879] -> w1857 mode=indexing
                      tunnel: [w1878] -> w1856 mode=indexing
                      tunnel: [w1877] -> w1855 mode=indexing
                      tunnel: [w1876] -> w1854 mode=indexing
                      tunnel: [w1875] -> w1853 mode=indexing
                      tunnel: [w1874] -> w1852 mode=indexing
                      tunnel: [w1873] -> w1851 mode=indexing
                      tunnel: w1850 -> [w1872]
                      n1095 = property on="path RLC_completo" class="Path"() -> ("Value"=w1871:path)  [unwired: 2 in, 2 out]
                      n1096 = stacked-sequence {
                        tunnel: w1891 -> [_ w1916 w1941 w1966 w1991 w2016 w2041 w2066 w2089 w2114 w2141 w2164 w2191 w2216 w2241 w2264 w2291 _]
                        tunnel: w1890 -> [w1892 _ _ _ _ _ _ _ _ _ _ _ _ _ _ _ _ w2315]
                        tunnel: [_ _ _ _ _ _ _ _ _ _ _ _ _ _ _ _ _ TRUE] -> w1889
                        tunnel: [_ w1915 _ _ _ _ _ _ _ _ _ _ _ _ _ _ _ _] -> w1888
                        tunnel: [_ _ w1940 _ _ _ _ _ _ _ _ _ _ _ _ _ _ _] -> w1887
                        tunnel: [_ _ _ w1965 _ _ _ _ _ _ _ _ _ _ _ _ _ _] -> w1886
                        tunnel: [_ _ _ _ w1990 _ _ _ _ _ _ _ _ _ _ _ _ _] -> w1885
                        tunnel: [_ _ _ _ _ w2015 _ _ _ _ _ _ _ _ _ _ _ _] -> w1884
                        tunnel: [_ _ _ _ _ _ w2040 _ _ _ _ _ _ _ _ _ _ _] -> w1883
                        tunnel: [_ _ _ _ _ _ _ w2065 _ _ _ _ _ _ _ _ _ _] -> w1882
                        tunnel: [_ _ _ _ _ _ _ _ w2091 _ _ _ _ _ _ _ _ _] -> w1881
                        tunnel: [_ _ _ _ _ _ _ _ _ w2116 _ _ _ _ _ _ _ _] -> w1880
                        tunnel: [_ _ _ _ _ _ _ _ _ _ w2140 _ _ _ _ _ _ _] -> w1879
                        tunnel: [_ _ _ _ _ _ _ _ _ _ _ w2166 _ _ _ _ _ _] -> w1878
                        tunnel: [_ _ _ _ _ _ _ _ _ _ _ _ w2190 _ _ _ _ _] -> w1877
                        tunnel: [_ _ _ _ _ _ _ _ _ _ _ _ _ w2215 _ _ _ _] -> w1876
                        tunnel: [_ _ _ _ _ _ _ _ _ _ _ _ _ _ w2240 _ _ _] -> w1875
                        tunnel: [_ _ _ _ _ _ _ _ _ _ _ _ _ _ _ w2266 _ _] -> w1874
                        tunnel: [_ _ _ _ _ _ _ _ _ _ _ _ _ _ _ _ w2290 _] -> w1873
                        tunnel: w1872 -> [_ w1918 w1944 w1968 w1993 w2018 w2043 w2068 w2093 w2118 w2143 w2168 w2193 w2218 w2243 w2268 w2293 _]
                        tunnel: w1871 -> [w1894 w1917 w1943 w1967 w1992 w2017 w2042 w2067 w2092 w2117 w2142 w2167 w2192 w2217 w2242 w2267 w2292 _]
                        frame #0 {
                          w1895 = "\t"
                          n1097 = local write "C-50-L"(w1892) -> ()
                          n1098 = local write "C-50-N"(w1892) -> ()
                          n1099 = local write "Z-50-L"(w1892) -> ()
                          n1100 = local write "Z-50-N"(w1892) -> ()
                          n1101 = local write "C-1K-L"(w1892) -> ()
                          n1102 = local write "C-1K-N"(w1892) -> ()
                          n1103 = local write "Z-1K-N"(w1892) -> ()
                          n1104 = local write "Z-1K-L"(w1892) -> ()
                          n1105 = local write "Z-100-L"(w1892) -> ()
                          n1106 = local write "C-10K-L"(w1892) -> ()
                          n1107 = local write "C-100-N"(w1892) -> ()
                          n1108 = local write "C-10K-N"(w1892) -> ()
                          n1109 = local write "Z-10K-N"(w1892) -> ()
                          n1110 = local write "Z-10K-L"(w1892) -> ()
                          n1111 = local write "Z-100-N"(w1892) -> ()
                          n1112 = local write "C-100-L"(w1892) -> ()
                          n1113 = Open/Create/Replace File(file path (use dialog)=w1894, operation (0:open)=T3."open") -> (refnum out=w1908:refnum<file>, error out=w1907:errorcluster)  [unwired: 2 in, 3 out]
                          n1114 = Get Date/Time String(date format (0)=enum16{"short", "long", "abbreviated"}."short", want seconds? (F)=TRUE) -> (date string=w1900:string, time string=w1899:string)  [unwired: 1 in]
                          n1115 = feedback #4() -> (w1893:dbl)  [unwired: 1 in]
                          n1116 = local write "SET 2"(w1893) -> ()
                          n1117 = Set File Position(refnum=w1908, from (0:start)=enum16{"start", "end", "current"}."end", error in=w1907) -> (refnum out=w1910:refnum<file>, error out=w1911:errorcluster)  [unwired: 1 in]
                          n1118 = Number To Fractional String(number=w1893, precision (6)=i16 2) -> (F-format string=w1898:string)  [unwired: 2 in]
                          n1119 = Add(x=w1893, y=0.2) -> (x+y=w1904:dbl)
                          n1120 = feedback-in #4(w1904) -> ()
                          n1121 = Concatenate Strings(w1898, w1895, w1900, w1895, w1899, w1895) -> (w1897:string)
                          n1122 = Write to Text File(file (use dialog)=w1910, text=w1897, error in=w1911) -> (refnum out=w1906:refnum<file>, error out=w1905:errorcluster)  [unwired: 1 in, 1 out]
                          n1123 = Close File(refnum=w1906, error in=w1905) -> (error out=w1913:errorcluster)  [unwired: 1 out]
                          n1124 = call <vilib>:"Simple Error Handler.vi"("error in (no error)"=w1913) -> ()  [unwired: 1 in, 8 out]
                        }
                        frame #1 {
                          w1919 = "\t"
                          w1936 = i16 4 ("width (-)")
                          n1125 = local write "C-50-L"(w1916) -> ()
                          n1126 = Wait (ms)(milliseconds to wait=u32 5000) -> ()  [unwired: 1 out]
                          n1127 = Open/Create/Replace File(file path (use dialog)=w1917, operation (0:open)=T3."open") -> (refnum out=w1928:refnum<file>, error out=w1927:errorcluster)  [unwired: 2 in, 3 out]
                          n1128 = Set File Position(refnum=w1928, from (0:start)=enum16{"start", "end", "current"}."end", error in=w1927) -> (refnum out=w1930:refnum<file>, error out=w1931:errorcluster)  [unwired: 1 in]
                          n1129 = call "RLC_read.vi"("Path"=w1918, "String"="cmd /c rlc_read_cAL.py") -> ("MEASURE A"=w1915:dbl, "MEASURE V [V]"=w1935:dbl, "MEASURE B"=w1914:dbl, "MEASURE I [A]"=w1934:dbl)  [unwired: 2 out]
                          n1130 = Number To Engineering String(2:w1936, 4:w1934) -> (0:w1920:string)  [unwired: 2 in]
                          n1131 = local write "MEASURE A"(w1915) -> ()
                          n1132 = local write "MEASURE B"(w1914) -> ()
                          n1133 = Number To Engineering String(2:w1936, 4:w1935) -> (0:w1921:string)  [unwired: 2 in]
                          n1134 = Number To Engineering String(2:w1936, 4:w1915) -> (0:w1923:string)  [unwired: 2 in]
                          n1135 = Number To Engineering String(2:w1936, 4:w1914) -> (0:w1922:string)  [unwired: 2 in]
                          n1136 = Concatenate Strings(w1923, w1919, w1922, w1919, w1921, w1919, w1920, w1919) -> (w1924:string)
                          n1137 = Write to Text File(file (use dialog)=w1930, text=w1924, error in=w1931) -> (refnum out=w1926:refnum<file>, error out=w1925:errorcluster)  [unwired: 1 in, 1 out]
                          n1138 = Close File(refnum=w1926, error in=w1925) -> (error out=w1933:errorcluster)  [unwired: 1 out]
                          n1139 = call <vilib>:"Simple Error Handler.vi"("error in (no error)"=w1933) -> ()  [unwired: 1 in, 8 out]
                        }
                        frame #2 {
                          w1947 = "\t"
                          w1961 = i16 4 ("width (-)")
                          n1140 = local write "C-50-N"(w1941) -> ()
                          n1141 = Wait (ms)(milliseconds to wait=u32 5000) -> ()  [unwired: 1 out]
                          n1142 = Open/Create/Replace File(file path (use dialog)=w1943, operation (0:open)=T3."open") -> (refnum out=w1955:refnum<file>, error out=w1954:errorcluster)  [unwired: 2 in, 3 out]
                          n1143 = Set File Position(refnum=w1955, from (0:start)=enum16{"start", "end", "current"}."end", error in=w1954) -> (refnum out=w1957:refnum<file>, error out=w1958:errorcluster)  [unwired: 1 in]
                          n1144 = call "RLC_read.vi"("Path"=w1944, "String"="cmd /c rlc_read_cAN.py") -> ("MEASURE A"=w1940:dbl, "MEASURE V [V]"=w1946:dbl, "MEASURE B"=w1939:dbl, "MEASURE I [A]"=w1945:dbl)  [unwired: 2 out]
                          n1145 = Number To Engineering String(2:w1961, 4:w1945) -> (0:w1948:string)  [unwired: 2 in]
                          n1146 = local write "MEASURE A 2"(w1940) -> ()
                          n1147 = local write "MEASURE B 2"(w1939) -> ()
                          n1148 = Number To Engineering String(2:w1961, 4:w1946) -> (0:w1949:string)  [unwired: 2 in]
                          n1149 = Number To Engineering String(2:w1961, 4:w1940) -> (0:w1951:string)  [unwired: 2 in]
                          n1150 = Number To Engineering String(2:w1961, 4:w1939) -> (0:w1950:string)  [unwired: 2 in]
                          n1151 = Concatenate Strings(w1951, w1947, w1950, w1947, w1949, w1947, w1948, w1947) -> (w1942:string)
                          n1152 = Write to Text File(file (use dialog)=w1957, text=w1942, error in=w1958) -> (refnum out=w1953:refnum<file>, error out=w1952:errorcluster)  [unwired: 1 in, 1 out]
                          n1153 = Close File(refnum=w1953, error in=w1952) -> (error out=w1960:errorcluster)  [unwired: 1 out]
                          n1154 = call <vilib>:"Simple Error Handler.vi"("error in (no error)"=w1960) -> ()  [unwired: 1 in, 8 out]
                        }
                        frame #3 {
                          w1971 = "\t"
                          w1986 = i16 4 ("width (-)")
                          n1155 = Wait (ms)(milliseconds to wait=u32 5000) -> ()  [unwired: 1 out]
                          n1156 = local write "C-100-L"(w1966) -> ()
                          n1157 = Open/Create/Replace File(file path (use dialog)=w1967, operation (0:open)=T3."open") -> (refnum out=w1980:refnum<file>, error out=w1979:errorcluster)  [unwired: 2 in, 3 out]
                          n1158 = Set File Position(refnum=w1980, from (0:start)=enum16{"start", "end", "current"}."end", error in=w1979) -> (refnum out=w1982:refnum<file>, error out=w1983:errorcluster)  [unwired: 1 in]
                          n1159 = call "RLC_read.vi"("Path"=w1968, "String"="cmd /c rlc_read_cBL.py") -> ("MEASURE A"=w1965:dbl, "MEASURE V [V]"=w1970:dbl, "MEASURE B"=w1964:dbl, "MEASURE I [A]"=w1969:dbl)  [unwired: 2 out]
                          n1160 = Number To Engineering String(2:w1986, 4:w1969) -> (0:w1972:string)  [unwired: 2 in]
                          n1161 = local write "MEASURE A 3"(w1965) -> ()
                          n1162 = local write "MEASURE B 3"(w1964) -> ()
                          n1163 = Number To Engineering String(2:w1986, 4:w1970) -> (0:w1973:string)  [unwired: 2 in]
                          n1164 = Number To Engineering String(2:w1986, 4:w1965) -> (0:w1975:string)  [unwired: 2 in]
                          n1165 = Number To Engineering String(2:w1986, 4:w1964) -> (0:w1974:string)  [unwired: 2 in]
                          n1166 = Concatenate Strings(w1975, w1971, w1974, w1971, w1973, w1971, w1972, w1971) -> (w1976:string)
                          n1167 = Write to Text File(file (use dialog)=w1982, text=w1976, error in=w1983) -> (refnum out=w1978:refnum<file>, error out=w1977:errorcluster)  [unwired: 1 in, 1 out]
                          n1168 = Close File(refnum=w1978, error in=w1977) -> (error out=w1985:errorcluster)  [unwired: 1 out]
                          n1169 = call <vilib>:"Simple Error Handler.vi"("error in (no error)"=w1985) -> ()  [unwired: 1 in, 8 out]
                        }
                        frame #4 {
                          w1996 = "\t"
                          w2011 = i16 4 ("width (-)")
                          n1170 = Wait (ms)(milliseconds to wait=u32 5000) -> ()  [unwired: 1 out]
                          n1171 = local write "C-100-N"(w1991) -> ()
                          n1172 = Open/Create/Replace File(file path (use dialog)=w1992, operation (0:open)=T3."open") -> (refnum out=w2005:refnum<file>, error out=w2004:errorcluster)  [unwired: 2 in, 3 out]
                          n1173 = Set File Position(refnum=w2005, from (0:start)=enum16{"start", "end", "current"}."end", error in=w2004) -> (refnum out=w2007:refnum<file>, error out=w2008:errorcluster)  [unwired: 1 in]
                          n1174 = call "RLC_read.vi"("Path"=w1993, "String"="cmd /c rlc_read_cBN.py") -> ("MEASURE A"=w1990:dbl, "MEASURE V [V]"=w1995:dbl, "MEASURE B"=w1989:dbl, "MEASURE I [A]"=w1994:dbl)  [unwired: 2 out]
                          n1175 = Number To Engineering String(2:w2011, 4:w1994) -> (0:w1997:string)  [unwired: 2 in]
                          n1176 = local write "MEASURE A 4"(w1990) -> ()
                          n1177 = local write "MEASURE B 4"(w1989) -> ()
                          n1178 = Number To Engineering String(2:w2011, 4:w1995) -> (0:w1998:string)  [unwired: 2 in]
                          n1179 = Number To Engineering String(2:w2011, 4:w1990) -> (0:w2000:string)  [unwired: 2 in]
                          n1180 = Number To Engineering String(2:w2011, 4:w1989) -> (0:w1999:string)  [unwired: 2 in]
                          n1181 = Concatenate Strings(w2000, w1996, w1999, w1996, w1998, w1996, w1997, w1996) -> (w2001:string)
                          n1182 = Write to Text File(file (use dialog)=w2007, text=w2001, error in=w2008) -> (refnum out=w2003:refnum<file>, error out=w2002:errorcluster)  [unwired: 1 in, 1 out]
                          n1183 = Close File(refnum=w2003, error in=w2002) -> (error out=w2010:errorcluster)  [unwired: 1 out]
                          n1184 = call <vilib>:"Simple Error Handler.vi"("error in (no error)"=w2010) -> ()  [unwired: 1 in, 8 out]
                        }
                        frame #5 {
                          w2036 = "\t"
                          w2021 = i16 4 ("width (-)")
                          n1185 = local write "C-1K-L"(w2016) -> ()
                          n1186 = Wait (ms)(milliseconds to wait=u32 5000) -> ()  [unwired: 1 out]
                          n1187 = Open/Create/Replace File(file path (use dialog)=w2017, operation (0:open)=T3."open") -> (refnum out=w2027:refnum<file>, error out=w2028:errorcluster)  [unwired: 2 in, 3 out]
                          n1188 = Set File Position(refnum=w2027, from (0:start)=enum16{"start", "end", "current"}."end", error in=w2028) -> (refnum out=w2025:refnum<file>, error out=w2024:errorcluster)  [unwired: 1 in]
                          n1189 = call "RLC_read.vi"("Path"=w2018, "String"="cmd /c rlc_read_cCL.py") -> ("MEASURE A"=w2015:dbl, "MEASURE V [V]"=w2020:dbl, "MEASURE B"=w2014:dbl, "MEASURE I [A]"=w2019:dbl)  [unwired: 2 out]
                          n1190 = Number To Engineering String(2:w2021, 4:w2019) -> (0:w2035:string)  [unwired: 2 in]
                          n1191 = local write "MEASURE A 5"(w2015) -> ()
                          n1192 = local write "MEASURE B 5"(w2014) -> ()
                          n1193 = Number To Engineering String(2:w2021, 4:w2020) -> (0:w2034:string)  [unwired: 2 in]
                          n1194 = Number To Engineering String(2:w2021, 4:w2015) -> (0:w2032:string)  [unwired: 2 in]
                          n1195 = Number To Engineering String(2:w2021, 4:w2014) -> (0:w2033:string)  [unwired: 2 in]
                          n1196 = Concatenate Strings(w2032, w2036, w2033, w2036, w2034, w2036, w2035, w2036) -> (w2031:string)
                          n1197 = Write to Text File(file (use dialog)=w2025, text=w2031, error in=w2024) -> (refnum out=w2029:refnum<file>, error out=w2030:errorcluster)  [unwired: 1 in, 1 out]
                          n1198 = Close File(refnum=w2029, error in=w2030) -> (error out=w2022:errorcluster)  [unwired: 1 out]
                          n1199 = call <vilib>:"Simple Error Handler.vi"("error in (no error)"=w2022) -> ()  [unwired: 1 in, 8 out]
                        }
                        frame #6 {
                          w2061 = "\t"
                          w2046 = i16 4 ("width (-)")
                          n1200 = local write "C-1K-N"(w2041) -> ()
                          n1201 = Wait (ms)(milliseconds to wait=u32 5000) -> ()  [unwired: 1 out]
                          n1202 = Open/Create/Replace File(file path (use dialog)=w2042, operation (0:open)=T3."open") -> (refnum out=w2052:refnum<file>, error out=w2053:errorcluster)  [unwired: 2 in, 3 out]
                          n1203 = Set File Position(refnum=w2052, from (0:start)=enum16{"start", "end", "current"}."end", error in=w2053) -> (refnum out=w2050:refnum<file>, error out=w2049:errorcluster)  [unwired: 1 in]
                          n1204 = call "RLC_read.vi"("Path"=w2043, "String"="cmd /c rlc_read_cCN.py") -> ("MEASURE A"=w2040:dbl, "MEASURE V [V]"=w2045:dbl, "MEASURE B"=w2039:dbl, "MEASURE I [A]"=w2044:dbl)  [unwired: 2 out]
                          n1205 = Number To Engineering String(2:w2046, 4:w2044) -> (0:w2060:string)  [unwired: 2 in]
                          n1206 = local write "MEASURE A 6"(w2040) -> ()
                          n1207 = local write "MEASURE B 6"(w2039) -> ()
                          n1208 = Number To Engineering String(2:w2046, 4:w2045) -> (0:w2059:string)  [unwired: 2 in]
                          n1209 = Number To Engineering String(2:w2046, 4:w2040) -> (0:w2057:string)  [unwired: 2 in]
                          n1210 = Number To Engineering String(2:w2046, 4:w2039) -> (0:w2058:string)  [unwired: 2 in]
                          n1211 = Concatenate Strings(w2057, w2061, w2058, w2061, w2059, w2061, w2060, w2061) -> (w2056:string)
                          n1212 = Write to Text File(file (use dialog)=w2050, text=w2056, error in=w2049) -> (refnum out=w2054:refnum<file>, error out=w2055:errorcluster)  [unwired: 1 in, 1 out]
                          n1213 = Close File(refnum=w2054, error in=w2055) -> (error out=w2047:errorcluster)  [unwired: 1 out]
                          n1214 = call <vilib>:"Simple Error Handler.vi"("error in (no error)"=w2047) -> ()  [unwired: 1 in, 8 out]
                        }
                        frame #7 {
                          w2071 = "\t"
                          w2086 = i16 4 ("width (-)")
                          n1215 = Wait (ms)(milliseconds to wait=u32 5000) -> ()  [unwired: 1 out]
                          n1216 = local write "C-10K-L"(w2066) -> ()
                          n1217 = Open/Create/Replace File(file path (use dialog)=w2067, operation (0:open)=T3."open") -> (refnum out=w2080:refnum<file>, error out=w2079:errorcluster)  [unwired: 2 in, 3 out]
                          n1218 = Set File Position(refnum=w2080, from (0:start)=enum16{"start", "end", "current"}."end", error in=w2079) -> (refnum out=w2082:refnum<file>, error out=w2083:errorcluster)  [unwired: 1 in]
                          n1219 = call "RLC_read.vi"("Path"=w2068, "String"="cmd /c rlc_read_cDL.py") -> ("MEASURE A"=w2065:dbl, "MEASURE V [V]"=w2070:dbl, "MEASURE B"=w2064:dbl, "MEASURE I [A]"=w2069:dbl)  [unwired: 2 out]
                          n1220 = Number To Engineering String(2:w2086, 4:w2069) -> (0:w2072:string)  [unwired: 2 in]
                          n1221 = local write "MEASURE A 7"(w2065) -> ()
                          n1222 = local write "MEASURE B 7"(w2064) -> ()
                          n1223 = Number To Engineering String(2:w2086, 4:w2070) -> (0:w2073:string)  [unwired: 2 in]
                          n1224 = Number To Engineering String(2:w2086, 4:w2065) -> (0:w2075:string)  [unwired: 2 in]
                          n1225 = Number To Engineering String(2:w2086, 4:w2064) -> (0:w2074:string)  [unwired: 2 in]
                          n1226 = Concatenate Strings(w2075, w2071, w2074, w2071, w2073, w2071, w2072, w2071) -> (w2076:string)
                          n1227 = Write to Text File(file (use dialog)=w2082, text=w2076, error in=w2083) -> (refnum out=w2078:refnum<file>, error out=w2077:errorcluster)  [unwired: 1 in, 1 out]
                          n1228 = Close File(refnum=w2078, error in=w2077) -> (error out=w2085:errorcluster)  [unwired: 1 out]
                          n1229 = call <vilib>:"Simple Error Handler.vi"("error in (no error)"=w2085) -> ()  [unwired: 1 in, 8 out]
                        }
                        frame #8 {
                          w2096 = "\t"
                          w2111 = i16 4 ("width (-)")
                          n1230 = Wait (ms)(milliseconds to wait=u32 5000) -> ()  [unwired: 1 out]
                          n1231 = local write "C-10K-N"(w2089) -> ()
                          n1232 = Open/Create/Replace File(file path (use dialog)=w2092, operation (0:open)=T3."open") -> (refnum out=w2105:refnum<file>, error out=w2104:errorcluster)  [unwired: 2 in, 3 out]
                          n1233 = Set File Position(refnum=w2105, from (0:start)=enum16{"start", "end", "current"}."end", error in=w2104) -> (refnum out=w2107:refnum<file>, error out=w2108:errorcluster)  [unwired: 1 in]
                          n1234 = call "RLC_read.vi"("Path"=w2093, "String"="cmd /c rlc_read_cDN.py") -> ("MEASURE A"=w2091:dbl, "MEASURE V [V]"=w2095:dbl, "MEASURE B"=w2090:dbl, "MEASURE I [A]"=w2094:dbl)  [unwired: 2 out]
                          n1235 = Number To Engineering String(2:w2111, 4:w2094) -> (0:w2097:string)  [unwired: 2 in]
                          n1236 = local write "MEASURE A 8"(w2091) -> ()
                          n1237 = local write "MEASURE B 8"(w2090) -> ()
                          n1238 = Number To Engineering String(2:w2111, 4:w2095) -> (0:w2098:string)  [unwired: 2 in]
                          n1239 = Number To Engineering String(2:w2111, 4:w2091) -> (0:w2100:string)  [unwired: 2 in]
                          n1240 = Number To Engineering String(2:w2111, 4:w2090) -> (0:w2099:string)  [unwired: 2 in]
                          n1241 = Concatenate Strings(w2100, w2096, w2099, w2096, w2098, w2096, w2097, w2096) -> (w2101:string)
                          n1242 = Write to Text File(file (use dialog)=w2107, text=w2101, error in=w2108) -> (refnum out=w2103:refnum<file>, error out=w2102:errorcluster)  [unwired: 1 in, 1 out]
                          n1243 = Close File(refnum=w2103, error in=w2102) -> (error out=w2110:errorcluster)  [unwired: 1 out]
                          n1244 = call <vilib>:"Simple Error Handler.vi"("error in (no error)"=w2110) -> ()  [unwired: 1 in, 8 out]
                        }
                        frame #9 {
                          w2121 = "\t"
                          w2136 = i16 4 ("width (-)")
                          n1245 = local write "Z-50-L"(w2114) -> ()
                          n1246 = Wait (ms)(milliseconds to wait=u32 5000) -> ()  [unwired: 1 out]
                          n1247 = Open/Create/Replace File(file path (use dialog)=w2117, operation (0:open)=T3."open") -> (refnum out=w2130:refnum<file>, error out=w2129:errorcluster)  [unwired: 2 in, 3 out]
                          n1248 = Set File Position(refnum=w2130, from (0:start)=enum16{"start", "end", "current"}."end", error in=w2129) -> (refnum out=w2132:refnum<file>, error out=w2133:errorcluster)  [unwired: 1 in]
                          n1249 = call "RLC_read.vi"("Path"=w2118, "String"="cmd /c rlc_read_ZAL.py") -> ("MEASURE A"=w2116:dbl, "MEASURE V [V]"=w2120:dbl, "MEASURE B"=w2115:dbl, "MEASURE I [A]"=w2119:dbl)  [unwired: 2 out]
                          n1250 = Number To Engineering String(2:w2136, 4:w2119) -> (0:w2122:string)  [unwired: 2 in]
                          n1251 = local write "MEASURE A 9"(w2116) -> ()
                          n1252 = local write "MEASURE B 9"(w2115) -> ()
                          n1253 = Number To Engineering String(2:w2136, 4:w2120) -> (0:w2123:string)  [unwired: 2 in]
                          n1254 = Number To Engineering String(2:w2136, 4:w2116) -> (0:w2125:string)  [unwired: 2 in]
                          n1255 = Number To Engineering String(2:w2136, 4:w2115) -> (0:w2124:string)  [unwired: 2 in]
                          n1256 = Concatenate Strings(w2125, w2121, w2124, w2121, w2123, w2121, w2122, w2121) -> (w2126:string)
                          n1257 = Write to Text File(file (use dialog)=w2132, text=w2126, error in=w2133) -> (refnum out=w2128:refnum<file>, error out=w2127:errorcluster)  [unwired: 1 in, 1 out]
                          n1258 = Close File(refnum=w2128, error in=w2127) -> (error out=w2135:errorcluster)  [unwired: 1 out]
                          n1259 = call <vilib>:"Simple Error Handler.vi"("error in (no error)"=w2135) -> ()  [unwired: 1 in, 8 out]
                        }
                        frame #10 {
                          w2146 = "\t"
                          w2161 = i16 4 ("width (-)")
                          n1260 = local write "Z-50-N"(w2141) -> ()
                          n1261 = Wait (ms)(milliseconds to wait=u32 5000) -> ()  [unwired: 1 out]
                          n1262 = Open/Create/Replace File(file path (use dialog)=w2142, operation (0:open)=T3."open") -> (refnum out=w2155:refnum<file>, error out=w2154:errorcluster)  [unwired: 2 in, 3 out]
                          n1263 = Set File Position(refnum=w2155, from (0:start)=enum16{"start", "end", "current"}."end", error in=w2154) -> (refnum out=w2157:refnum<file>, error out=w2158:errorcluster)  [unwired: 1 in]
                          n1264 = call "RLC_read.vi"("Path"=w2143, "String"="cmd /c rlc_read_ZAN.py") -> ("MEASURE A"=w2140:dbl, "MEASURE V [V]"=w2145:dbl, "MEASURE B"=w2139:dbl, "MEASURE I [A]"=w2144:dbl)  [unwired: 2 out]
                          n1265 = Number To Engineering String(2:w2161, 4:w2144) -> (0:w2147:string)  [unwired: 2 in]
                          n1266 = local write "MEASURE A 10"(w2140) -> ()
                          n1267 = local write "MEASURE B 10"(w2139) -> ()
                          n1268 = Number To Engineering String(2:w2161, 4:w2145) -> (0:w2148:string)  [unwired: 2 in]
                          n1269 = Number To Engineering String(2:w2161, 4:w2140) -> (0:w2150:string)  [unwired: 2 in]
                          n1270 = Number To Engineering String(2:w2161, 4:w2139) -> (0:w2149:string)  [unwired: 2 in]
                          n1271 = Concatenate Strings(w2150, w2146, w2149, w2146, w2148, w2146, w2147, w2146) -> (w2151:string)
                          n1272 = Write to Text File(file (use dialog)=w2157, text=w2151, error in=w2158) -> (refnum out=w2153:refnum<file>, error out=w2152:errorcluster)  [unwired: 1 in, 1 out]
                          n1273 = Close File(refnum=w2153, error in=w2152) -> (error out=w2160:errorcluster)  [unwired: 1 out]
                          n1274 = call <vilib>:"Simple Error Handler.vi"("error in (no error)"=w2160) -> ()  [unwired: 1 in, 8 out]
                        }
                        frame #11 {
                          w2171 = "\t"
                          w2186 = i16 4 ("width (-)")
                          n1275 = Wait (ms)(milliseconds to wait=u32 5000) -> ()  [unwired: 1 out]
                          n1276 = local write "Z-100-L"(w2164) -> ()
                          n1277 = Open/Create/Replace File(file path (use dialog)=w2167, operation (0:open)=T3."open") -> (refnum out=w2180:refnum<file>, error out=w2179:errorcluster)  [unwired: 2 in, 3 out]
                          n1278 = Set File Position(refnum=w2180, from (0:start)=enum16{"start", "end", "current"}."end", error in=w2179) -> (refnum out=w2182:refnum<file>, error out=w2183:errorcluster)  [unwired: 1 in]
                          n1279 = call "RLC_read.vi"("Path"=w2168, "String"="cmd /c rlc_read_ZBL.py") -> ("MEASURE A"=w2166:dbl, "MEASURE V [V]"=w2170:dbl, "MEASURE B"=w2165:dbl, "MEASURE I [A]"=w2169:dbl)  [unwired: 2 out]
                          n1280 = Number To Engineering String(2:w2186, 4:w2169) -> (0:w2172:string)  [unwired: 2 in]
                          n1281 = local write "MEASURE A 11"(w2166) -> ()
                          n1282 = local write "MEASURE B 11"(w2165) -> ()
                          n1283 = Number To Engineering String(2:w2186, 4:w2170) -> (0:w2173:string)  [unwired: 2 in]
                          n1284 = Number To Engineering String(2:w2186, 4:w2166) -> (0:w2175:string)  [unwired: 2 in]
                          n1285 = Number To Engineering String(2:w2186, 4:w2165) -> (0:w2174:string)  [unwired: 2 in]
                          n1286 = Concatenate Strings(w2175, w2171, w2174, w2171, w2173, w2171, w2172, w2171) -> (w2176:string)
                          n1287 = Write to Text File(file (use dialog)=w2182, text=w2176, error in=w2183) -> (refnum out=w2178:refnum<file>, error out=w2177:errorcluster)  [unwired: 1 in, 1 out]
                          n1288 = Close File(refnum=w2178, error in=w2177) -> (error out=w2185:errorcluster)  [unwired: 1 out]
                          n1289 = call <vilib>:"Simple Error Handler.vi"("error in (no error)"=w2185) -> ()  [unwired: 1 in, 8 out]
                        }
                        frame #12 {
                          w2196 = "\t"
                          w2211 = i16 4 ("width (-)")
                          n1290 = Wait (ms)(milliseconds to wait=u32 5000) -> ()  [unwired: 1 out]
                          n1291 = local write "Z-100-N"(w2191) -> ()
                          n1292 = Open/Create/Replace File(file path (use dialog)=w2192, operation (0:open)=T3."open") -> (refnum out=w2205:refnum<file>, error out=w2204:errorcluster)  [unwired: 2 in, 3 out]
                          n1293 = Set File Position(refnum=w2205, from (0:start)=enum16{"start", "end", "current"}."end", error in=w2204) -> (refnum out=w2207:refnum<file>, error out=w2208:errorcluster)  [unwired: 1 in]
                          n1294 = call "RLC_read.vi"("Path"=w2193, "String"="cmd /c rlc_read_ZBN.py") -> ("MEASURE A"=w2190:dbl, "MEASURE V [V]"=w2195:dbl, "MEASURE B"=w2189:dbl, "MEASURE I [A]"=w2194:dbl)  [unwired: 2 out]
                          n1295 = Number To Engineering String(2:w2211, 4:w2194) -> (0:w2197:string)  [unwired: 2 in]
                          n1296 = local write "MEASURE A 12"(w2190) -> ()
                          n1297 = local write "MEASURE B 12"(w2189) -> ()
                          n1298 = Number To Engineering String(2:w2211, 4:w2195) -> (0:w2198:string)  [unwired: 2 in]
                          n1299 = Number To Engineering String(2:w2211, 4:w2190) -> (0:w2200:string)  [unwired: 2 in]
                          n1300 = Number To Engineering String(2:w2211, 4:w2189) -> (0:w2199:string)  [unwired: 2 in]
                          n1301 = Concatenate Strings(w2200, w2196, w2199, w2196, w2198, w2196, w2197, w2196) -> (w2201:string)
                          n1302 = Write to Text File(file (use dialog)=w2207, text=w2201, error in=w2208) -> (refnum out=w2203:refnum<file>, error out=w2202:errorcluster)  [unwired: 1 in, 1 out]
                          n1303 = Close File(refnum=w2203, error in=w2202) -> (error out=w2210:errorcluster)  [unwired: 1 out]
                          n1304 = call <vilib>:"Simple Error Handler.vi"("error in (no error)"=w2210) -> ()  [unwired: 1 in, 8 out]
                        }
                        frame #13 {
                          w2221 = "\t"
                          w2236 = i16 4 ("width (-)")
                          n1305 = local write "Z-1K-L"(w2216) -> ()
                          n1306 = Wait (ms)(milliseconds to wait=u32 5000) -> ()  [unwired: 1 out]
                          n1307 = Open/Create/Replace File(file path (use dialog)=w2217, operation (0:open)=T3."open") -> (refnum out=w2230:refnum<file>, error out=w2229:errorcluster)  [unwired: 2 in, 3 out]
                          n1308 = Set File Position(refnum=w2230, from (0:start)=enum16{"start", "end", "current"}."end", error in=w2229) -> (refnum out=w2232:refnum<file>, error out=w2233:errorcluster)  [unwired: 1 in]
                          n1309 = call "RLC_read.vi"("Path"=w2218, "String"="cmd /c rlc_read_ZCL.py") -> ("MEASURE A"=w2215:dbl, "MEASURE V [V]"=w2220:dbl, "MEASURE B"=w2214:dbl, "MEASURE I [A]"=w2219:dbl)  [unwired: 2 out]
                          n1310 = Number To Engineering String(2:w2236, 4:w2219) -> (0:w2222:string)  [unwired: 2 in]
                          n1311 = local write "MEASURE A 13"(w2215) -> ()
                          n1312 = local write "MEASURE B 13"(w2214) -> ()
                          n1313 = Number To Engineering String(2:w2236, 4:w2220) -> (0:w2223:string)  [unwired: 2 in]
                          n1314 = Number To Engineering String(2:w2236, 4:w2215) -> (0:w2225:string)  [unwired: 2 in]
                          n1315 = Number To Engineering String(2:w2236, 4:w2214) -> (0:w2224:string)  [unwired: 2 in]
                          n1316 = Concatenate Strings(w2225, w2221, w2224, w2221, w2223, w2221, w2222, w2221) -> (w2226:string)
                          n1317 = Write to Text File(file (use dialog)=w2232, text=w2226, error in=w2233) -> (refnum out=w2228:refnum<file>, error out=w2227:errorcluster)  [unwired: 1 in, 1 out]
                          n1318 = Close File(refnum=w2228, error in=w2227) -> (error out=w2235:errorcluster)  [unwired: 1 out]
                          n1319 = call <vilib>:"Simple Error Handler.vi"("error in (no error)"=w2235) -> ()  [unwired: 1 in, 8 out]
                        }
                        frame #14 {
                          w2246 = "\t"
                          w2261 = i16 4 ("width (-)")
                          n1320 = local write "Z-1K-N"(w2241) -> ()
                          n1321 = Wait (ms)(milliseconds to wait=u32 5000) -> ()  [unwired: 1 out]
                          n1322 = Open/Create/Replace File(file path (use dialog)=w2242, operation (0:open)=T3."open") -> (refnum out=w2255:refnum<file>, error out=w2254:errorcluster)  [unwired: 2 in, 3 out]
                          n1323 = Set File Position(refnum=w2255, from (0:start)=enum16{"start", "end", "current"}."end", error in=w2254) -> (refnum out=w2257:refnum<file>, error out=w2258:errorcluster)  [unwired: 1 in]
                          n1324 = call "RLC_read.vi"("Path"=w2243, "String"="cmd /c rlc_read_ZCN.py") -> ("MEASURE A"=w2240:dbl, "MEASURE V [V]"=w2245:dbl, "MEASURE B"=w2239:dbl, "MEASURE I [A]"=w2244:dbl)  [unwired: 2 out]
                          n1325 = Number To Engineering String(2:w2261, 4:w2244) -> (0:w2247:string)  [unwired: 2 in]
                          n1326 = local write "MEASURE A 14"(w2240) -> ()
                          n1327 = local write "MEASURE B 14"(w2239) -> ()
                          n1328 = Number To Engineering String(2:w2261, 4:w2245) -> (0:w2248:string)  [unwired: 2 in]
                          n1329 = Number To Engineering String(2:w2261, 4:w2240) -> (0:w2250:string)  [unwired: 2 in]
                          n1330 = Number To Engineering String(2:w2261, 4:w2239) -> (0:w2249:string)  [unwired: 2 in]
                          n1331 = Concatenate Strings(w2250, w2246, w2249, w2246, w2248, w2246, w2247, w2246) -> (w2251:string)
                          n1332 = Write to Text File(file (use dialog)=w2257, text=w2251, error in=w2258) -> (refnum out=w2253:refnum<file>, error out=w2252:errorcluster)  [unwired: 1 in, 1 out]
                          n1333 = Close File(refnum=w2253, error in=w2252) -> (error out=w2260:errorcluster)  [unwired: 1 out]
                          n1334 = call <vilib>:"Simple Error Handler.vi"("error in (no error)"=w2260) -> ()  [unwired: 1 in, 8 out]
                        }
                        frame #15 {
                          w2271 = "\t"
                          w2286 = i16 4 ("width (-)")
                          n1335 = Wait (ms)(milliseconds to wait=u32 5000) -> ()  [unwired: 1 out]
                          n1336 = local write "Z-10K-L"(w2264) -> ()
                          n1337 = Open/Create/Replace File(file path (use dialog)=w2267, operation (0:open)=T3."open") -> (refnum out=w2280:refnum<file>, error out=w2279:errorcluster)  [unwired: 2 in, 3 out]
                          n1338 = Set File Position(refnum=w2280, from (0:start)=enum16{"start", "end", "current"}."end", error in=w2279) -> (refnum out=w2282:refnum<file>, error out=w2283:errorcluster)  [unwired: 1 in]
                          n1339 = call "RLC_read.vi"("Path"=w2268, "String"="cmd /c rlc_read_ZDL.py") -> ("MEASURE A"=w2266:dbl, "MEASURE V [V]"=w2270:dbl, "MEASURE B"=w2265:dbl, "MEASURE I [A]"=w2269:dbl)  [unwired: 2 out]
                          n1340 = Number To Engineering String(2:w2286, 4:w2269) -> (0:w2272:string)  [unwired: 2 in]
                          n1341 = local write "MEASURE A 15"(w2266) -> ()
                          n1342 = local write "MEASURE B 15"(w2265) -> ()
                          n1343 = Number To Engineering String(2:w2286, 4:w2270) -> (0:w2273:string)  [unwired: 2 in]
                          n1344 = Number To Engineering String(2:w2286, 4:w2266) -> (0:w2275:string)  [unwired: 2 in]
                          n1345 = Number To Engineering String(2:w2286, 4:w2265) -> (0:w2274:string)  [unwired: 2 in]
                          n1346 = Concatenate Strings(w2275, w2271, w2274, w2271, w2273, w2271, w2272, w2271) -> (w2276:string)
                          n1347 = Write to Text File(file (use dialog)=w2282, text=w2276, error in=w2283) -> (refnum out=w2278:refnum<file>, error out=w2277:errorcluster)  [unwired: 1 in, 1 out]
                          n1348 = Close File(refnum=w2278, error in=w2277) -> (error out=w2285:errorcluster)  [unwired: 1 out]
                          n1349 = call <vilib>:"Simple Error Handler.vi"("error in (no error)"=w2285) -> ()  [unwired: 1 in, 8 out]
                        }
                        frame #16 {
                          w2297 = "\t"
                          w2312 = i16 4 ("width (-)")
                          n1350 = Wait (ms)(milliseconds to wait=u32 5000) -> ()  [unwired: 1 out]
                          n1351 = local write "Z-10K-N"(w2291) -> ()
                          n1352 = Open/Create/Replace File(file path (use dialog)=w2292, operation (0:open)=T3."open") -> (refnum out=w2306:refnum<file>, error out=w2305:errorcluster)  [unwired: 2 in, 3 out]
                          n1353 = Set File Position(refnum=w2306, from (0:start)=enum16{"start", "end", "current"}."end", error in=w2305) -> (refnum out=w2308:refnum<file>, error out=w2309:errorcluster)  [unwired: 1 in]
                          n1354 = call "RLC_read.vi"("Path"=w2293, "String"="cmd /c rlc_read_ZDN.py") -> ("MEASURE A"=w2290:dbl, "MEASURE V [V]"=w2296:dbl, "MEASURE B"=w2289:dbl, "MEASURE I [A]"=w2295:dbl)  [unwired: 2 out]
                          n1355 = Number To Engineering String(2:w2312, 4:w2295) -> (0:w2298:string)  [unwired: 2 in]
                          n1356 = local write "MEASURE A 16"(w2290) -> ()
                          n1357 = local write "MEASURE B 16"(w2289) -> ()
                          n1358 = Number To Engineering String(2:w2312, 4:w2296) -> (0:w2299:string)  [unwired: 2 in]
                          n1359 = Number To Engineering String(2:w2312, 4:w2290) -> (0:w2301:string)  [unwired: 2 in]
                          n1360 = Number To Engineering String(2:w2312, 4:w2289) -> (0:w2300:string)  [unwired: 2 in]
                          n1361 = Concatenate Strings(w2301, w2297, w2300, w2297, w2299, w2297, w2298, w2297, "\r\n") -> (w2302:string)
                          n1362 = Write to Text File(file (use dialog)=w2308, text=w2302, error in=w2309) -> (refnum out=w2304:refnum<file>, error out=w2303:errorcluster)  [unwired: 1 in, 1 out]
                          n1363 = Close File(refnum=w2304, error in=w2303) -> (error out=w2311:errorcluster)  [unwired: 1 out]
                          n1364 = call <vilib>:"Simple Error Handler.vi"("error in (no error)"=w2311) -> ()  [unwired: 1 in, 8 out]
                        }
                        frame #17 {
                          n1365 = local write "Z-50-N"(w2315) -> ()
                          n1366 = local write "Z-50-L"(w2315) -> ()
                          n1367 = local write "C-1K-N"(w2315) -> ()
                          n1368 = local write "C-50-N"(w2315) -> ()
                          n1369 = local write "C-50-L"(w2315) -> ()
                          n1370 = local write "Z-1K-N"(w2315) -> ()
                          n1371 = local write "C-1K-L"(w2315) -> ()
                          n1372 = local write "Z-1K-L"(w2315) -> ()
                          n1373 = local write "Z-100-L"(w2315) -> ()
                          n1374 = local write "C-10K-L"(w2315) -> ()
                          n1375 = local write "Z-10K-L"(w2315) -> ()
                          n1376 = local write "C-10K-N"(w2315) -> ()
                          n1377 = local write "Z-10K-N"(w2315) -> ()
                          n1378 = local write "C-100-N"(w2315) -> ()
                          n1379 = local write "C-100-L"(w2315) -> ()
                          n1380 = local write "Z-100-N"(w2315) -> ()
                        }
                      }
                    }
                    n1381 = call <vilib>:"Mean.vi"("X"=w1866) -> ("mean"=w1849:dbl)  [unwired: 1 out]
                    n1382 = call <vilib>:"Mean.vi"("X"=w1865) -> ("mean"=w1848:dbl)  [unwired: 1 out]
                    n1383 = call <vilib>:"Mean.vi"("X"=w1864) -> ("mean"=w1847:dbl)  [unwired: 1 out]
                    n1384 = call <vilib>:"Mean.vi"("X"=w1863) -> ("mean"=w1846:dbl)  [unwired: 1 out]
                    n1385 = call <vilib>:"Mean.vi"("X"=w1862) -> ("mean"=w1845:dbl)  [unwired: 1 out]
                    n1386 = call <vilib>:"Mean.vi"("X"=w1861) -> ("mean"=w1844:dbl)  [unwired: 1 out]
                    n1387 = call <vilib>:"Mean.vi"("X"=w1860) -> ("mean"=w1843:dbl)  [unwired: 1 out]
                    n1388 = call <vilib>:"Mean.vi"("X"=w1859) -> ("mean"=w1842:dbl)  [unwired: 1 out]
                    n1389 = call <vilib>:"Mean.vi"("X"=w1858) -> ("mean"=w1841:dbl)  [unwired: 1 out]
                    n1390 = call <vilib>:"Mean.vi"("X"=w1857) -> ("mean"=w1840:dbl)  [unwired: 1 out]
                    n1391 = call <vilib>:"Mean.vi"("X"=w1856) -> ("mean"=w1839:dbl)  [unwired: 1 out]
                    n1392 = call <vilib>:"Mean.vi"("X"=w1855) -> ("mean"=w1838:dbl)  [unwired: 1 out]
                    n1393 = call <vilib>:"Mean.vi"("X"=w1854) -> ("mean"=w1837:dbl)  [unwired: 1 out]
                    n1394 = call <vilib>:"Mean.vi"("X"=w1853) -> ("mean"=w1836:dbl)  [unwired: 1 out]
                    n1395 = call <vilib>:"Mean.vi"("X"=w1852) -> ("mean"=w1835:dbl)  [unwired: 1 out]
                    n1396 = call <vilib>:"Mean.vi"("X"=w1851) -> ("mean"=w1834:dbl)  [unwired: 1 out]
                    n1397 = local write "mean"(w1849) -> ()
                    n1398 = local write "mean 2"(w1848) -> ()
                    n1399 = local write "mean 3"(w1847) -> ()
                    n1400 = local write "mean 4"(w1846) -> ()
                    n1401 = local write "mean 5"(w1845) -> ()
                    n1402 = local write "mean 6"(w1844) -> ()
                    n1403 = local write "mean 7"(w1843) -> ()
                    n1404 = local write "mean 8"(w1842) -> ()
                    n1405 = local write "mean 9"(w1841) -> ()
                    n1406 = local write "mean 10"(w1840) -> ()
                    n1407 = local write "mean 11"(w1839) -> ()
                    n1408 = local write "mean 12"(w1838) -> ()
                    n1409 = local write "mean 13"(w1837) -> ()
                    n1410 = local write "mean 14"(w1836) -> ()
                    n1411 = local write "mean 15"(w1835) -> ()
                    n1412 = local write "mean 16"(w1834) -> ()
                  }
                }
              }
              frame #2 {
                n1413 = case shown="True" w2317 {
                  tunnel: w2334 -> [_ w2350]
                  tunnel: w2333 -> [_ w2349]
                  tunnel: w2332 -> [_ w2348]
                  tunnel: w2331 -> [_ w2347]
                  tunnel: w2330 -> [_ w2346]
                  tunnel: w2329 -> [_ w2345]
                  tunnel: w2328 -> [_ w2344]
                  tunnel: w2327 -> [_ w2343]
                  tunnel: w2326 -> [_ w2342]
                  tunnel: w2325 -> [_ w2341]
                  tunnel: w2324 -> [_ w2340]
                  tunnel: w2323 -> [_ w2339]
                  tunnel: w2322 -> [_ w2338]
                  tunnel: w2321 -> [_ w2337]
                  tunnel: w2320 -> [_ w2336]
                  tunnel: w2319 -> [_ w2335]
                  frame False {
                  }
                  frame True {
                    w2365 = "\t"
                    w2382 = i16 4 ("precision (6)")
                    n1414 = property on="SET" class="DigNum (strict)"() -> ("Value"=w2351:i32)  [unwired: 2 in, 2 out]
                    n1415 = Number To Engineering String(2:w2382, 4:w2350) -> (0:w2380:string)  [unwired: 2 in]
                    n1416 = Number To Engineering String(2:w2382, 4:w2349) -> (0:w2379:string)  [unwired: 2 in]
                    n1417 = Number To Engineering String(2:w2382, 4:w2348) -> (0:w2378:string)  [unwired: 2 in]
                    n1418 = Number To Engineering String(2:w2382, 4:w2347) -> (0:w2377:string)  [unwired: 2 in]
                    n1419 = Number To Engineering String(2:w2382, 4:w2346) -> (0:w2376:string)  [unwired: 2 in]
                    n1420 = Number To Engineering String(2:w2382, 4:w2345) -> (0:w2375:string)  [unwired: 2 in]
                    n1421 = Number To Engineering String(2:w2382, 4:w2344) -> (0:w2374:string)  [unwired: 2 in]
                    n1422 = Number To Engineering String(2:w2382, 4:w2343) -> (0:w2373:string)  [unwired: 2 in]
                    n1423 = Number To Engineering String(2:w2382, 4:w2342) -> (0:w2372:string)  [unwired: 2 in]
                    n1424 = Number To Engineering String(2:w2382, 4:w2341) -> (0:w2371:string)  [unwired: 2 in]
                    n1425 = Number To Engineering String(2:w2382, 4:w2335) -> (0:w2370:string)  [unwired: 2 in]
                    n1426 = Number To Engineering String(2:w2382, 4:w2340) -> (0:w2369:string)  [unwired: 2 in]
                    n1427 = Number To Engineering String(2:w2382, 4:w2339) -> (0:w2368:string)  [unwired: 2 in]
                    n1428 = Number To Engineering String(2:w2382, 4:w2338) -> (0:w2367:string)  [unwired: 2 in]
                    n1429 = Number To Engineering String(2:w2382, 4:w2337) -> (0:w2366:string)  [unwired: 2 in]
                    n1430 = Number To Engineering String(2:w2382, 4:w2336) -> (0:w2364:string)  [unwired: 2 in]
                    n1431 = Number To Decimal String(number=w2351) -> (decimal integer string=w2381:string)  [unwired: 1 in]
                    n1432 = property on="path RLC_mean" class="Path"() -> ("Value"=w2352:path)  [unwired: 2 in, 2 out]
                    n1433 = Open/Create/Replace File(file path (use dialog)=w2352, operation (0:open)=T3."open") -> (refnum out=w2357:refnum<file>, error out=w2356:errorcluster)  [unwired: 2 in, 3 out]
                    n1434 = Concatenate Strings(w2381, w2365, w2380, w2365, w2379, w2365, w2378, w2365, w2377, w2365, w2376, w2365, w2375, w2365, w2374, w2365, w2373, w2365, w2372, w2365, w2371, w2365, w2370, w2365, w2369, w2365, w2368, w2365, w2367, w2365, w2366, w2365, w2364, "\r\n") -> (w2353:string)
                    n1435 = Set File Position(refnum=w2357, from (0:start)=enum16{"start", "end", "current"}."end", error in=w2356) -> (refnum out=w2359:refnum<file>, error out=w2360:errorcluster)  [unwired: 1 in]
                    n1436 = Write to Text File(file (use dialog)=w2359, text=w2353, error in=w2360) -> (refnum out=w2355:refnum<file>, error out=w2354:errorcluster)  [unwired: 1 in, 1 out]
                    n1437 = Close File(refnum=w2355, error in=w2354) -> (error out=w2362:errorcluster)  [unwired: 1 out]
                    n1438 = call <vilib>:"Simple Error Handler.vi"("error in (no error)"=w2362) -> ()  [unwired: 1 in, 8 out]
                  }
                }
              }
            }
            n1439 = local write "graph RLC"(w1789) -> ()
          }
        }
        n1440 = call <vilib>:"Linear Fit.vi"("Y"=w1762, "X"=w1766) -> ("Best Linear Fit"=w1764:dbl[], "slope"=→"bar/N":dbl)  [unwired: 9 in, 3 out]
        n1441 = Bundle(w1766, w1762) -> (w1769:cluster{i32[], dbl[]})  [unwired: 1 in]
        n1442 = call <vilib>:"General Polynomial Fit.vi"("Y"=w1771, "polynomial order"=w1787, "X"=w1766) -> ("Best Polynomial Fit"=w1783:dbl[], "Polynomial Coefficients"=w1784:dbl[])  [unwired: 9 in, 2 out]
        "Polynomial Coefficients 2" <- w1784
        n1443 = call <vilib>:"General Polynomial Fit.vi"("Y"=w1762, "polynomial order"=w1787, "X"=w1780) -> ("Best Polynomial Fit"=w1765:dbl[], "Polynomial Coefficients"=w1778:dbl[])  [unwired: 9 in, 2 out]
        "Polynomial Coefficients" <- w1778
        n1444 = Bundle(w1766, "Best Polynomial Fit"=w1765) -> (w1768:cluster{i32[], "Best Polynomial Fit":dbl[]})  [unwired: 1 in]
        n1445 = Build Array(w1771, w1783) -> (→"Linear Model Graph 2":dbl[][])
        n1446 = Index Array(array=w1778, index=0) -> (element=→"p fit":dbl)
        n1447 = Index Array(array=w1784, index=0) -> (element=→"T fit":dbl)
        n1448 = Build Array(w1762, w1765, w1764) -> (→"Linear Model Graph":dbl[][])
        n1449 = Bundle(w1766, "Best Linear Fit"=w1764) -> (w1767:cluster{i32[], "Best Linear Fit":dbl[]})  [unwired: 1 in]
        n1450 = Build Array(w1769, w1768, w1767) -> ()  [unwired: 1 out]
      }
    }
    n1451 = case shown="True" "Close RLC 2" {
      tunnel: w37 -> [_ w167]
      frame False {
      }
      frame True {
        n1452 = call "RLC_close.vi"("Path"=w167) -> ("String"=w168:string)  [unwired: 10 in]
        n1453 = local write "RLC300 - digimess"(w168) -> ()
      }
    }
    n1454 = case shown="True" "Open Button 2" {
      frame False {
      }
      frame True {
        n1455 = property on="Sample name" class="Str"() -> ("Value"=w1741:string)  [unwired: 2 in, 2 out]
        n1456 = property on="File name" class="Str"() -> ("Value"=w1742:string)  [unwired: 2 in, 2 out]
        n1457 = property on="Nota" class="Str"() -> ("Value"=w1740:string)  [unwired: 2 in, 2 out]
        n1458 = call "Open file.vi"("Nota 01"=w1740, "Sample name"=w1741, "File name"=w1742) -> ("path open old"=w1739:path)  [unwired: 8 in]
        n1459 = local write "path"(w1739) -> ()
      }
    }
    n1460 = case shown="True" "Refresh Button 2" {
      frame False {
      }
      frame True {
        n1461 = property on="Waveform Chart" class="WFChart (strict)"("History Data"=dynamicdata[] []) -> ()  [unwired: 2 in, 2 out]
      }
    }
    n1462 = case shown="True" "Open Button" {
      frame False {
      }
      frame True {
        n1463 = flat-sequence {
          tunnel: ["Sample name"] -> w1745
          tunnel: ["Nota"] -> w1744
          tunnel: [w1747] -> w1743
          tunnel: w1745 -> [w1760]
          tunnel: w1744 -> [w1759]
          tunnel: w1743 -> [w1754]
          frame #0 {
            n1464 = local write "Count SET"(0 ("Count SET")) -> ()
            n1465 = local write "Set atual"(0 ("Count  3")) -> ()
            n1466 = call "File_data_new.vi"("Nota 01"="Nota", "Sample name"="Sample name", "File name"="File name") -> ("path"=w1747:path)  [unwired: 8 in]
            "path" <- w1747
          }
          frame #1 {
            w1755 = FALSE
            n1467 = Strip Path(path=w1754) -> (stripped path=w1753:path, name=w1752:string)
            n1468 = local write "Pf2"(w1755) -> ()
            n1469 = local write "ZPit"(w1755) -> ()
            n1470 = local write "Pit"(w1755) -> ()
            n1471 = local write "ZPf2"(w1755) -> ()
            n1472 = local write "T"(w1755) -> ()
            n1473 = Concatenate Strings(w1752, "_cinetica" ("string")) -> (w1757:string)
            n1474 = call "File_data_cinetica.vi"("path in"=w1753, "Nota 01"=w1759, "Sample name"=w1760, "File name"=w1757) -> ("path"=→"path 2_cinetica":path)  [unwired: 7 in]
          }
        }
      }
    }
    n1475 = local write "Manual Ctrl"(w50) -> ()
    n1476 = Or(x=w40, y=w39) -> (x .or. y?=w41:bool)
    n1477 = Or(x=w41, y="Refresh Button") -> (x .or. y?=w43:bool)
    n1478 = case shown="True" w43 {
      frame False {
      }
      frame True {
        n1479 = stacked-sequence {
          frame #0 {
            n1480 = property on="Waveform Chart P 2" class="WFChart (strict)"("History Data"=dbl[][] []) -> ()  [unwired: 2 in, 2 out]
          }
          frame #1 {
            n1481 = property on="path RLC_mean" class="Path"() -> ("Value"=w73:path)  [unwired: 2 in, 2 out]
            n1482 = Open/Create/Replace File(file path (use dialog)=w73, operation (0:open)=T3."open", access (0:read/write)=enum16{"read/write", "read-only", "write-only"}."read-only") -> (refnum out=w77:refnum<file>, error out=w76:errorcluster)  [unwired: 3 in, 1 out]
            n1483 = Read from Text File(file (use dialog)=w77, error in=w76) -> (refnum out=w82:refnum<file>, text=w78:string, error out=w81:errorcluster)  [unwired: 2 in, 1 out]
            n1484 = Close File(refnum=w82, error in=w81) -> ()  [unwired: 2 out]
            n1485 = Search/Split String(string=w78, search string/char (-)="SET\tDATE\tTIME\t\tP (BAR)\tT (ºC)\tC-50-L\tC-50-N\tC-100-L\tC-100-N\tC-1K-L\tC-1K-N\tC-10K-L\tC-10K-N\tZ-50-L\tZ-50-N\tZ-100-L\tZ-100-N\tZ-1K-L\tZ-1K-N\tZ-10K-L\tZ-10K-N") -> (match + rest of string=w83:string)  [unwired: 1 in, 2 out]
            n1486 = String Subset(string=w83, offset (0)=150) -> (substring=w90:string)  [unwired: 1 in]
            n1487 = Spreadsheet String To Array(format string="%#g", spreadsheet string=w90) -> (array=w89:dbl[][])  [unwired: 2 in]
            n1488 = Transpose Matrix(1:w89) -> (0:w103:dbl[][])
            n1489 = Index Array(array=w103, index (row)=1 ("index (row) 4")) -> (element=w104:dbl[])  [unwired: 1 in]
            n1490 = Index Array(array=w103, index (row)=2 ("index (row) 5")) -> (element=w105:dbl[])  [unwired: 1 in]
            n1491 = Index Array(array=w103, index (row)=3 ("index (row) 2")) -> (element=w106:dbl[])  [unwired: 1 in]
            n1492 = Index Array(array=w103, index (row)=4 ("index (row) 3")) -> (element=w107:dbl[])  [unwired: 1 in]
            n1493 = Index Array(array=w103, index (row)=5 ("index (row) 4")) -> (element=w108:dbl[])  [unwired: 1 in]
            n1494 = Index Array(array=w103, index (row)=6 ("index (row) 5")) -> (element=w109:dbl[])  [unwired: 1 in]
            n1495 = Index Array(array=w103, index (row)=7 ("index (row) 2")) -> (element=w110:dbl[])  [unwired: 1 in]
            n1496 = Index Array(array=w103, index (row)=8 ("index (row) 3")) -> (element=w111:dbl[])  [unwired: 1 in]
            n1497 = Index Array(array=w103, index (row)=9 ("index (row) 4")) -> (element=w72:dbl[])  [unwired: 1 in]
            n1498 = Index Array(array=w103, index (row)=10 ("index (row) 5")) -> (element=w71:dbl[])  [unwired: 1 in]
            n1499 = Index Array(array=w103, index (row)=11 ("index (row) 2")) -> (element=w70:dbl[])  [unwired: 1 in]
            n1500 = Index Array(array=w103, index (row)=12 ("index (row) 3")) -> (element=w69:dbl[])  [unwired: 1 in]
            n1501 = Index Array(array=w103, index (row)=13 ("index (row) 4")) -> (element=w68:dbl[])  [unwired: 1 in]
            n1502 = Index Array(array=w103, index (row)=14 ("index (row) 5")) -> (element=w67:dbl[])  [unwired: 1 in]
            n1503 = Index Array(array=w103, index (row)=15 ("index (row) 2")) -> (element=w66:dbl[])  [unwired: 1 in]
            n1504 = Index Array(array=w103, index (row)=16 ("index (row) 3")) -> (element=w65:dbl[])  [unwired: 1 in]
            n1505 = Build Array(w104, w105, w106, w107, w108, w109, w110, w111, w72, w71, w70, w69, w68, w67, w66, w65) -> (w64:dbl[][])
            n1506 = Transpose Matrix(1:w64) -> (0:→"Waveform Chart P 2":dbl[][])
          }
        }
      }
    }
  }
  n1507 = local write "path 2_cinetica"(path "C:/H2_Painel/painel_auto/cinetica.txt" ("path")) -> ()
  n1508 = local write "path RLC_completo"(path "C:/H2_Painel/painel_auto/RLC_full.txt" ("path RLC_mean")) -> ()
  n1509 = local write "path RLC_mean"(path "C:/H2_Painel/painel_auto/RLC_mean.txt" ("path RLC_mean")) -> ()
  n1510 = local write "path"(path "C:/H2_Painel/painel_auto/Arquivo_Padrao.txt" ("path")) -> ()
  n1511 = local write "Array"(dbl[] [0.5, 1.0, 2.0, 3.0, 4.0, 4.0, 4.0, 4.0, 4.0, 4.0, 4.0, 5.0, 5.0, 5.0, 7.0, 10.0, 15.0, 20.0, 25.0, 25.0, 25.0, 30.0, 40.0, 50.0, 60.0, 70.0] ("Array")) -> ()
